vi "Autonomous Independent.vi"() -> ()   [LabVIEW 2017]
doc: "This VI is called when autonomous begins, and will automatically be terminated when autonomous ends. You can carry out timed or sensor driven robot movement independently without needing to return to the caller."
uses:
  <vilib>/Rock Robotics/WPI/Utilities/WPI_GetSetVariantRefNum.vi
  <vilib>/Rock Robotics/Network Tables/NT Read String.vi
  <vilib>/Rock Robotics/Network Tables/NT Write Numeric Array.vi
  Robot Global Data.vi
  <vilib>/Rock Robotics/WPI/Solenoid/Deprecated/WPI_SolenoidSetBool.vi
  <vilib>/addons/control/pid/pid.llb/PID (DBL).vi
  <vilib>/addons/control/pid/NI_PID_pid.lvlib
panel:
  in  "Testing":T1(array[cluster])=[{"Left In/s"=0.0, "Right In/s"=0.0, "Duration"=0.5, "SOL A"=FALSE, "SOL B"=TRUE, "Lift Up"=TRUE, "Lift Down"=FALSE, "Intake In"=FALSE, "Intake Out"=FALSE, "Left Distance"=1.0, "Right Distance"=1.0, "Encoder Reset"=TRUE, "Wrist Up"=FALSE, "Wrist Down"=FALSE, "Lift Target"=0.0, "Wrist Target"=0.0}, {"Left In/s"=-1.0, "Right In/s"=-0.975, "Duration"=5.0, "SOL A"=FALSE, "SOL B"=TRUE, "Lift Up"=FALSE, "Lift Down"=FALSE, "Intake In"=FALSE, "Intake Out"=FALSE, "Left Distance"=300.0, "Right Distance"=300.0, "Encoder Reset"=FALSE, "Wrist Up"=FALSE, "Wrist Down"=FALSE, "Lift Target"=0.0, "Wrist Target"=0.0}, {"Left In/s"=0.0, "Right In/s"=0.0, "Duration"=0.5, "SOL A"=FALSE, "SOL B"=TRUE, "Lift Up"=FALSE, "Lift Down"=FALSE, "Intake In"=FALSE, "Intake Out"=FALSE, "Left Distance"=0.0, "Right Distance"=0.0, "Encoder Reset"=TRUE, "Wrist Up"=FALSE, "Wrist Down"=FALSE, "Lift Target"=0.0, "Wrist Target"=0.0}, {"Left In/s"=1.0, "Right In/s"=-0.975, "Duration"=5.0, "SOL A"=FALSE, "SOL B"=TRUE, "Lift Up"=FALSE, "Lift Down"=FALSE, "Intake In"=FALSE, "Intake Out"=FALSE, "Left Distance"=24.0, "Right Distance"=24.0, "Encoder Reset"=FALSE, "Wrist Up"=FALSE, "Wrist Down"=FALSE, "Lift Target"=0.0, "Wrist Target"=0.0}, {"Left In/s"=0.0, "Right In/s"=0.0, "Duration"=5.0, "SOL A"=FALSE, "SOL B"=TRUE, "Lift Up"=TRUE, "Lift Down"=FALSE, "Intake In"=FALSE, "Intake Out"=FALSE, "Left Distance"=10.0, "Right Distance"=10.0, "Encoder Reset"=FALSE, "Wrist Up"=FALSE, "Wrist Down"=FALSE, "Lift Target"=0.0, "Wrist Target"=0.0}, {"Left In/s"=0.0, "Right In/s"=0.0, "Duration"=0.75, "SOL A"=FALSE, "SOL B"=TRUE, "Lift Up"=FALSE, "Lift Down"=FALSE, "Intake In"=FALSE, "Intake Out"=TRUE, "Left Distance"=10.0, "Right Distance"=10.0, "Encoder Reset"=FALSE, "Wrist Up"=FALSE, "Wrist Down"=FALSE, "Lift Target"=0.0, "Wrist Target"=0.0}]
  in  "Right LLL":T2(array[cluster])=[{"Left Joystick"=1.0, "Right Joystick"=1.0, "Duration"=5.0, "SOL A"=FALSE, "SOL B"=FALSE, "Lift Up"=FALSE, "Lift Down"=FALSE, "Intake In"=FALSE, "Intake Out"=FALSE, "Left Distance"=252.0, "Right Distance"=252.0, "Encoder Reset"=FALSE, "Wrist Up"=FALSE, "Wrist Down"=FALSE}, {"Left Joystick"=-0.75, "Right Joystick"=0.75, "Duration"=2.0, "SOL A"=FALSE, "SOL B"=FALSE, "Lift Up"=FALSE, "Lift Down"=FALSE, "Intake In"=FALSE, "Intake Out"=FALSE, "Left Distance"=31.5, "Right Distance"=31.5, "Encoder Reset"=FALSE, "Wrist Up"=FALSE, "Wrist Down"=FALSE}]
  in  "Right RLR":T2(array[cluster])=[{"Left Joystick"=1.0, "Right Joystick"=1.0, "Duration"=5.0, "SOL A"=FALSE, "SOL B"=FALSE, "Lift Up"=FALSE, "Lift Down"=FALSE, "Intake In"=FALSE, "Intake Out"=FALSE, "Left Distance"=252.0, "Right Distance"=252.0, "Encoder Reset"=FALSE, "Wrist Up"=FALSE, "Wrist Down"=FALSE}, {"Left Joystick"=-0.75, "Right Joystick"=0.75, "Duration"=2.0, "SOL A"=FALSE, "SOL B"=FALSE, "Lift Up"=FALSE, "Lift Down"=FALSE, "Intake In"=FALSE, "Intake Out"=FALSE, "Left Distance"=31.5, "Right Distance"=31.5, "Encoder Reset"=FALSE, "Wrist Up"=FALSE, "Wrist Down"=FALSE}]
  in  "Right LRL":T2(array[cluster])=[{"Left Joystick"=1.0, "Right Joystick"=1.0, "Duration"=5.0, "SOL A"=FALSE, "SOL B"=FALSE, "Lift Up"=FALSE, "Lift Down"=FALSE, "Intake In"=FALSE, "Intake Out"=FALSE, "Left Distance"=252.0, "Right Distance"=252.0, "Encoder Reset"=FALSE, "Wrist Up"=FALSE, "Wrist Down"=FALSE}, {"Left Joystick"=-0.75, "Right Joystick"=0.75, "Duration"=2.0, "SOL A"=FALSE, "SOL B"=FALSE, "Lift Up"=FALSE, "Lift Down"=FALSE, "Intake In"=FALSE, "Intake Out"=FALSE, "Left Distance"=31.5, "Right Distance"=31.5, "Encoder Reset"=FALSE, "Wrist Up"=FALSE, "Wrist Down"=FALSE}]
  in  "Right RRR":T2(array[cluster])=[{"Left Joystick"=1.0, "Right Joystick"=1.0, "Duration"=5.0, "SOL A"=FALSE, "SOL B"=FALSE, "Lift Up"=FALSE, "Lift Down"=FALSE, "Intake In"=FALSE, "Intake Out"=FALSE, "Left Distance"=252.0, "Right Distance"=252.0, "Encoder Reset"=FALSE, "Wrist Up"=FALSE, "Wrist Down"=FALSE}, {"Left Joystick"=-0.75, "Right Joystick"=0.75, "Duration"=2.0, "SOL A"=FALSE, "SOL B"=FALSE, "Lift Up"=FALSE, "Lift Down"=FALSE, "Intake In"=FALSE, "Intake Out"=FALSE, "Left Distance"=31.5, "Right Distance"=31.5, "Encoder Reset"=FALSE, "Wrist Up"=FALSE, "Wrist Down"=FALSE}]
  in  "Center LLL":T2(array[cluster])=[{"Left Joystick"=1.0, "Right Joystick"=1.0, "Duration"=5.0, "SOL A"=FALSE, "SOL B"=FALSE, "Lift Up"=FALSE, "Lift Down"=FALSE, "Intake In"=FALSE, "Intake Out"=FALSE, "Left Distance"=252.0, "Right Distance"=252.0, "Encoder Reset"=FALSE, "Wrist Up"=FALSE, "Wrist Down"=FALSE}, {"Left Joystick"=-0.75, "Right Joystick"=0.75, "Duration"=2.0, "SOL A"=FALSE, "SOL B"=FALSE, "Lift Up"=FALSE, "Lift Down"=FALSE, "Intake In"=FALSE, "Intake Out"=FALSE, "Left Distance"=31.5, "Right Distance"=31.5, "Encoder Reset"=FALSE, "Wrist Up"=FALSE, "Wrist Down"=FALSE}]
  in  "Center RLR":T2(array[cluster])=[{"Left Joystick"=1.0, "Right Joystick"=1.0, "Duration"=5.0, "SOL A"=FALSE, "SOL B"=FALSE, "Lift Up"=FALSE, "Lift Down"=FALSE, "Intake In"=FALSE, "Intake Out"=FALSE, "Left Distance"=252.0, "Right Distance"=252.0, "Encoder Reset"=FALSE, "Wrist Up"=FALSE, "Wrist Down"=FALSE}, {"Left Joystick"=-0.75, "Right Joystick"=0.75, "Duration"=2.0, "SOL A"=FALSE, "SOL B"=FALSE, "Lift Up"=FALSE, "Lift Down"=FALSE, "Intake In"=FALSE, "Intake Out"=FALSE, "Left Distance"=31.5, "Right Distance"=31.5, "Encoder Reset"=FALSE, "Wrist Up"=FALSE, "Wrist Down"=FALSE}]
  in  "Center LRL":T2(array[cluster])=[{"Left Joystick"=1.0, "Right Joystick"=1.0, "Duration"=5.0, "SOL A"=FALSE, "SOL B"=FALSE, "Lift Up"=FALSE, "Lift Down"=FALSE, "Intake In"=FALSE, "Intake Out"=FALSE, "Left Distance"=252.0, "Right Distance"=252.0, "Encoder Reset"=FALSE, "Wrist Up"=FALSE, "Wrist Down"=FALSE}, {"Left Joystick"=-0.75, "Right Joystick"=0.75, "Duration"=2.0, "SOL A"=FALSE, "SOL B"=FALSE, "Lift Up"=FALSE, "Lift Down"=FALSE, "Intake In"=FALSE, "Intake Out"=FALSE, "Left Distance"=31.5, "Right Distance"=31.5, "Encoder Reset"=FALSE, "Wrist Up"=FALSE, "Wrist Down"=FALSE}]
  in  "Center RRR":T2(array[cluster])=[{"Left Joystick"=1.0, "Right Joystick"=1.0, "Duration"=5.0, "SOL A"=FALSE, "SOL B"=FALSE, "Lift Up"=FALSE, "Lift Down"=FALSE, "Intake In"=FALSE, "Intake Out"=FALSE, "Left Distance"=252.0, "Right Distance"=252.0, "Encoder Reset"=FALSE, "Wrist Up"=FALSE, "Wrist Down"=FALSE}, {"Left Joystick"=-0.75, "Right Joystick"=0.75, "Duration"=2.0, "SOL A"=FALSE, "SOL B"=FALSE, "Lift Up"=FALSE, "Lift Down"=FALSE, "Intake In"=FALSE, "Intake Out"=FALSE, "Left Distance"=31.5, "Right Distance"=31.5, "Encoder Reset"=FALSE, "Wrist Up"=FALSE, "Wrist Down"=FALSE}]
  in  "Left RLR":T2(array[cluster])=[{"Left Joystick"=1.0, "Right Joystick"=1.0, "Duration"=5.0, "SOL A"=FALSE, "SOL B"=FALSE, "Lift Up"=FALSE, "Lift Down"=FALSE, "Intake In"=FALSE, "Intake Out"=FALSE, "Left Distance"=252.0, "Right Distance"=252.0, "Encoder Reset"=FALSE, "Wrist Up"=FALSE, "Wrist Down"=FALSE}, {"Left Joystick"=-0.75, "Right Joystick"=0.75, "Duration"=2.0, "SOL A"=FALSE, "SOL B"=FALSE, "Lift Up"=FALSE, "Lift Down"=FALSE, "Intake In"=FALSE, "Intake Out"=FALSE, "Left Distance"=31.5, "Right Distance"=31.5, "Encoder Reset"=FALSE, "Wrist Up"=FALSE, "Wrist Down"=FALSE}]
  in  "Left LRL":T2(array[cluster])=[{"Left Joystick"=1.0, "Right Joystick"=1.0, "Duration"=5.0, "SOL A"=FALSE, "SOL B"=FALSE, "Lift Up"=FALSE, "Lift Down"=FALSE, "Intake In"=FALSE, "Intake Out"=FALSE, "Left Distance"=252.0, "Right Distance"=252.0, "Encoder Reset"=FALSE, "Wrist Up"=FALSE, "Wrist Down"=FALSE}, {"Left Joystick"=-0.75, "Right Joystick"=0.75, "Duration"=2.0, "SOL A"=FALSE, "SOL B"=FALSE, "Lift Up"=FALSE, "Lift Down"=FALSE, "Intake In"=FALSE, "Intake Out"=FALSE, "Left Distance"=31.5, "Right Distance"=31.5, "Encoder Reset"=FALSE, "Wrist Up"=FALSE, "Wrist Down"=FALSE}]
  in  "Left RRR":T2(array[cluster])=[{"Left Joystick"=1.0, "Right Joystick"=1.0, "Duration"=5.0, "SOL A"=FALSE, "SOL B"=FALSE, "Lift Up"=FALSE, "Lift Down"=FALSE, "Intake In"=FALSE, "Intake Out"=FALSE, "Left Distance"=252.0, "Right Distance"=252.0, "Encoder Reset"=FALSE, "Wrist Up"=FALSE, "Wrist Down"=FALSE}, {"Left Joystick"=-0.75, "Right Joystick"=0.75, "Duration"=2.0, "SOL A"=FALSE, "SOL B"=FALSE, "Lift Up"=FALSE, "Lift Down"=FALSE, "Intake In"=FALSE, "Intake Out"=FALSE, "Left Distance"=31.5, "Right Distance"=31.5, "Encoder Reset"=FALSE, "Wrist Up"=FALSE, "Wrist Down"=FALSE}]
  in  "Left LLL":T2(array[cluster])=[{"Left Joystick"=1.0, "Right Joystick"=1.0, "Duration"=5.0, "SOL A"=FALSE, "SOL B"=FALSE, "Lift Up"=FALSE, "Lift Down"=FALSE, "Intake In"=FALSE, "Intake Out"=FALSE, "Left Distance"=60.0, "Right Distance"=60.0, "Encoder Reset"=FALSE, "Wrist Up"=FALSE, "Wrist Down"=FALSE}, {"Left Joystick"=-0.75, "Right Joystick"=0.75, "Duration"=2.0, "SOL A"=FALSE, "SOL B"=FALSE, "Lift Up"=FALSE, "Lift Down"=FALSE, "Intake In"=FALSE, "Intake Out"=FALSE, "Left Distance"=31.5, "Right Distance"=31.5, "Encoder Reset"=FALSE, "Wrist Up"=FALSE, "Wrist Down"=FALSE}]
  # "Be sure to right-click and choose Data Operations>>Make Current Value default if you want to save the array values with the VI"
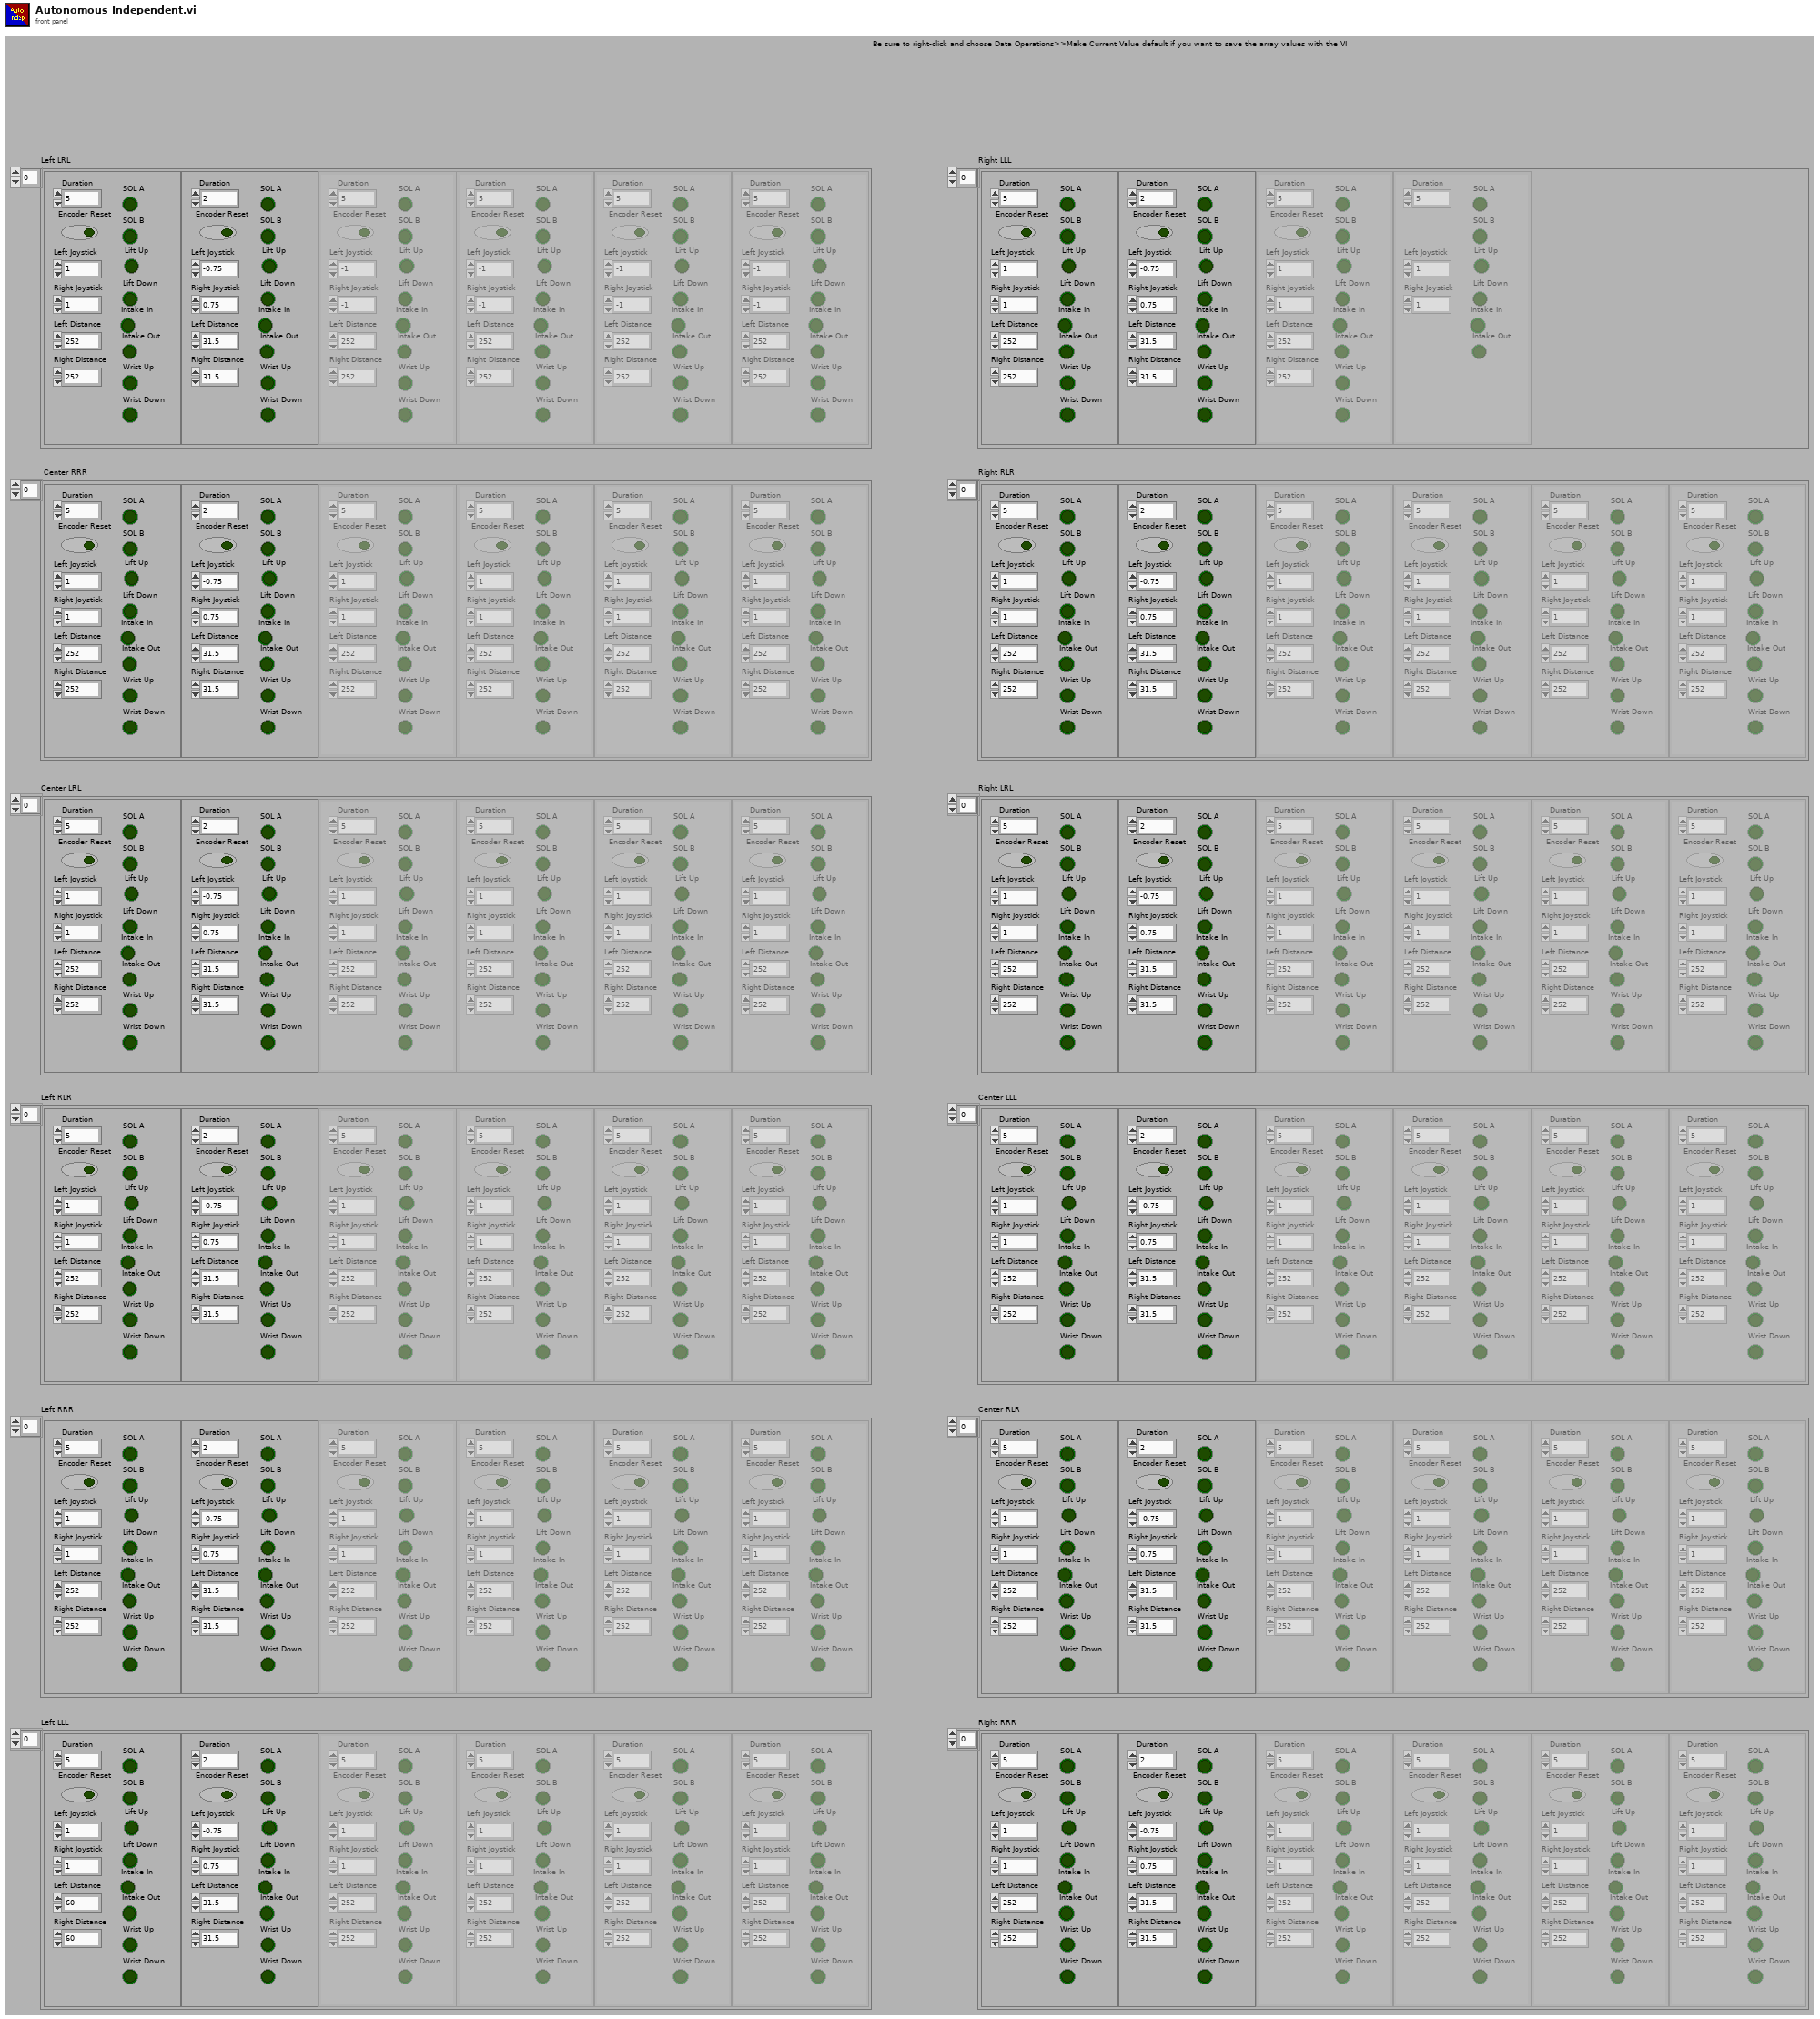
[diagram p1: front panel]
types:
  T1 = cluster{"Left In/s":dbl, "Right In/s":dbl, "Duration":dbl, "SOL A":bool, "SOL B":bool, "Lift Up":bool, "Lift Down":bool, "Intake In":bool, "Intake Out":bool, "Left Distance":dbl, "Right Distance":dbl, "Encoder Reset":bool, "Wrist Up":bool, "Wrist Down":bool, "Lift Target":dbl, "Wrist Target":dbl}[]
  T2 = cluster{"Left Joystick":dbl, "Right Joystick":dbl, "Duration":dbl, "SOL A":bool, "SOL B":bool, "Lift Up":bool, "Lift Down":bool, "Intake In":bool, "Intake Out":bool, "Left Distance":dbl, "Right Distance":dbl, "Encoder Reset":bool, "Wrist Up":bool, "Wrist Down":bool}[]
  T3 = typedef "WPI_JoystickDevRef.ctl" = cluster{"Device":T4}
  T4 = typedef "WPI_JoystickDeviceEnum.ctl" = enum16{"USB 0", "USB 1", "USB 2", "USB 3", "USB 4", "USB 5"}
  T5 = cluster{"proportional gain (Kc)":dbl, "integral time (Ti, min)":dbl, "derivative time (Td, min)":dbl}
  T6 = typedef "WPI_RobotDriveDevRef.ctl" = cluster{"DevStatus":errorcluster, "Motors[]":T7[], "Square Inputs":bool, "Max Output":dbl}
  T7 = typedef "WPI_MotorControlDeviceRef.ctl" = cluster{"DeviceStatus":errorcluster, "Type":T8, "PWM":cluster{"PWM Channel":T9, "DeadBand":T10}, "CAN":cluster{"Device Number":u8, "SetOutput VI Ref":variant, "GetOutput VI Ref":variant, "Enable VI Ref":variant, "Disable VI Ref":variant, "Data":variant}, "Invert":bool, "DIO PWM":cluster{"PWM \"Enable\" Channel":T9, "DIOChannel":T11, "PWM Rate":dbl}}
  T8 = typedef "WPI_MotorControlType.ctl" = enum16{"PWM", "CAN", "DIO PWM"}
  T9 = typedef "FPGA_DIOPWMChannel.ctl" = enum8{"PWM 0", "PWM 1", "PWM 2", "PWM 3", "PWM 4", "PWM 5", "PWM 6", "PWM 7", "PWM 8", "PWM 9", "PWM MXP 0", "PWM MXP 1", "PWM MXP 2", "PWM MXP 3", "PWM MXP 4", "PWM MXP 5", "PWM MXP 6", "PWM MXP 7", "PWM MXP 8", "PWM MXP 9", "Invalid"}
  T10 = typedef "WPI_PWMDeadband.ctl" = cluster{"Name":string, "maxPositivePwm":i32, "minPositivePwm":i32, "centerPwm":i32, "maxNegativePwm":i32, "minNegativePwm":i32, "angularRange":u16}
  T11 = typedef "FPGA_DIOChannel.ctl" = enum8{"DIO 0", "DIO 1", "DIO 2", "DIO 3", "DIO 4", "DIO 5", "DIO 6", "DIO 7", "DIO 8", "DIO 9", "DIO MXP 0", "DIO MXP 1", "DIO MXP 2", "DIO MXP 3", "DIO MXP 4", "DIO MXP 5", "DIO MXP 6", "DIO MXP 7", "DIO MXP 8", "DIO MXP 9", "DIO MXP 10", "DIO MXP 11", "DIO MXP 12", "DIO MXP 13", "DIO MXP 14", "DIO MXP 15", "SPI Port CS1", "SPI Port CS2", "SPI Port CS3", "SPI Port MISO", "SPI Port MOSI", "Invalid"}
  T12 = typedef "WPI_SolenoidDevRef.ctl" = cluster{"DevStatus":errorcluster, "Pneumatics Control Module":u8, "Forward Solenoid Channel":T13, "Reverse Solenoid Channel":T13}
  T13 = typedef "WPI_SolenoidChannel.ctl" = enum8{"Solenoid 0", "Solenoid 1", "Solenoid 2", "Solenoid 3", "Solenoid 4", "Solenoid 5", "Solenoid 6", "Solenoid 7", "Invalid"}
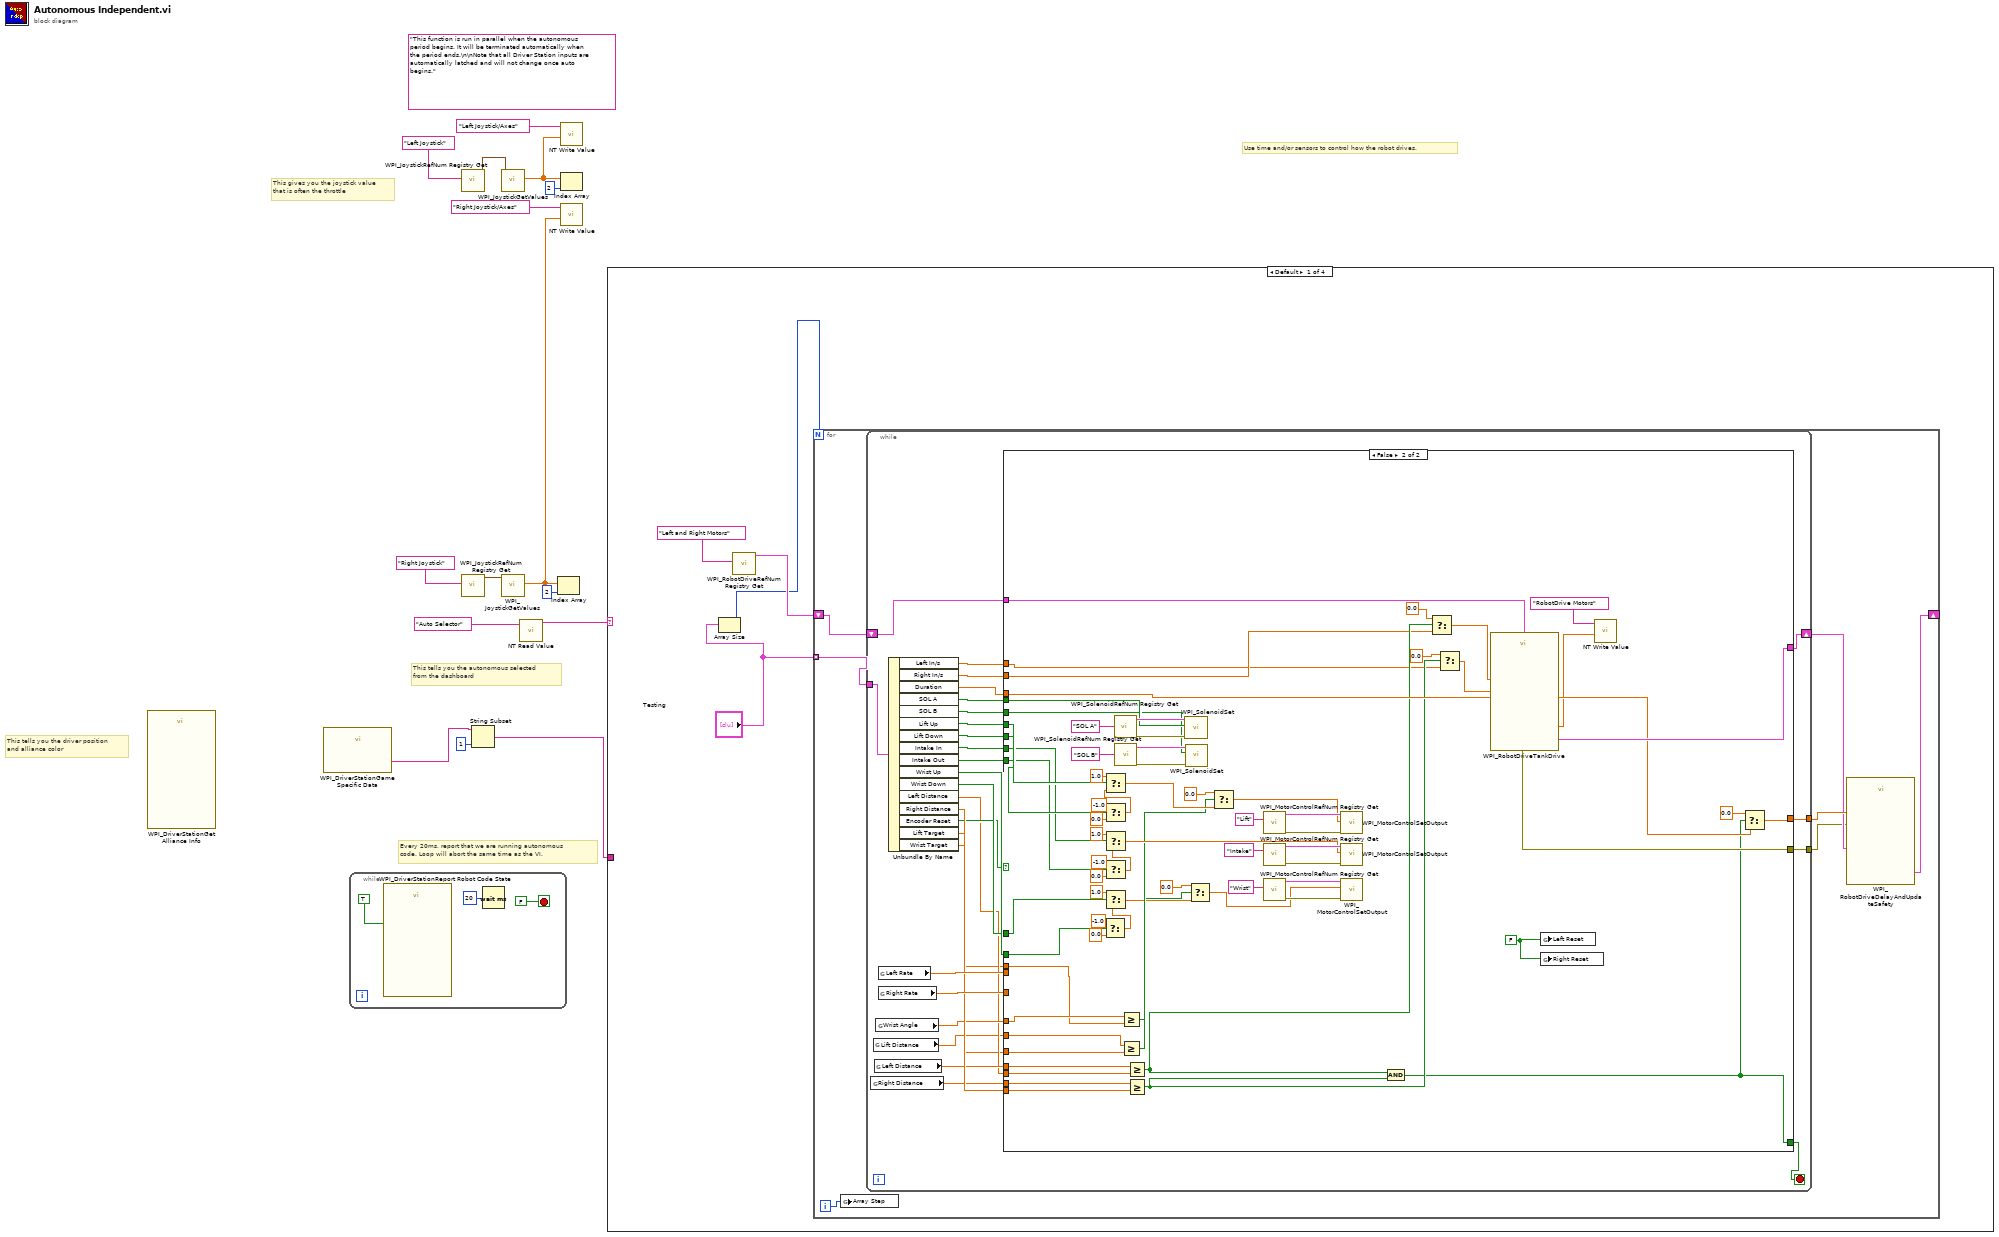
[diagram p0: block diagram]
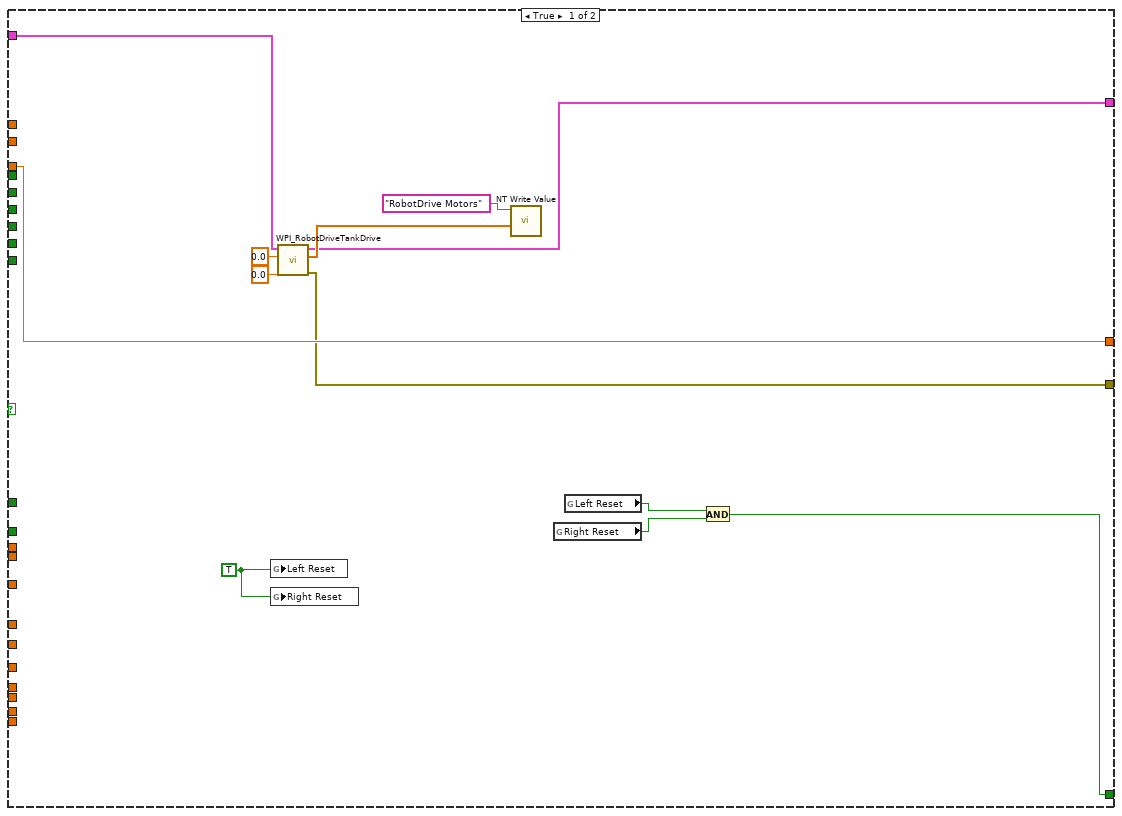
[diagram p2: hidden frame]
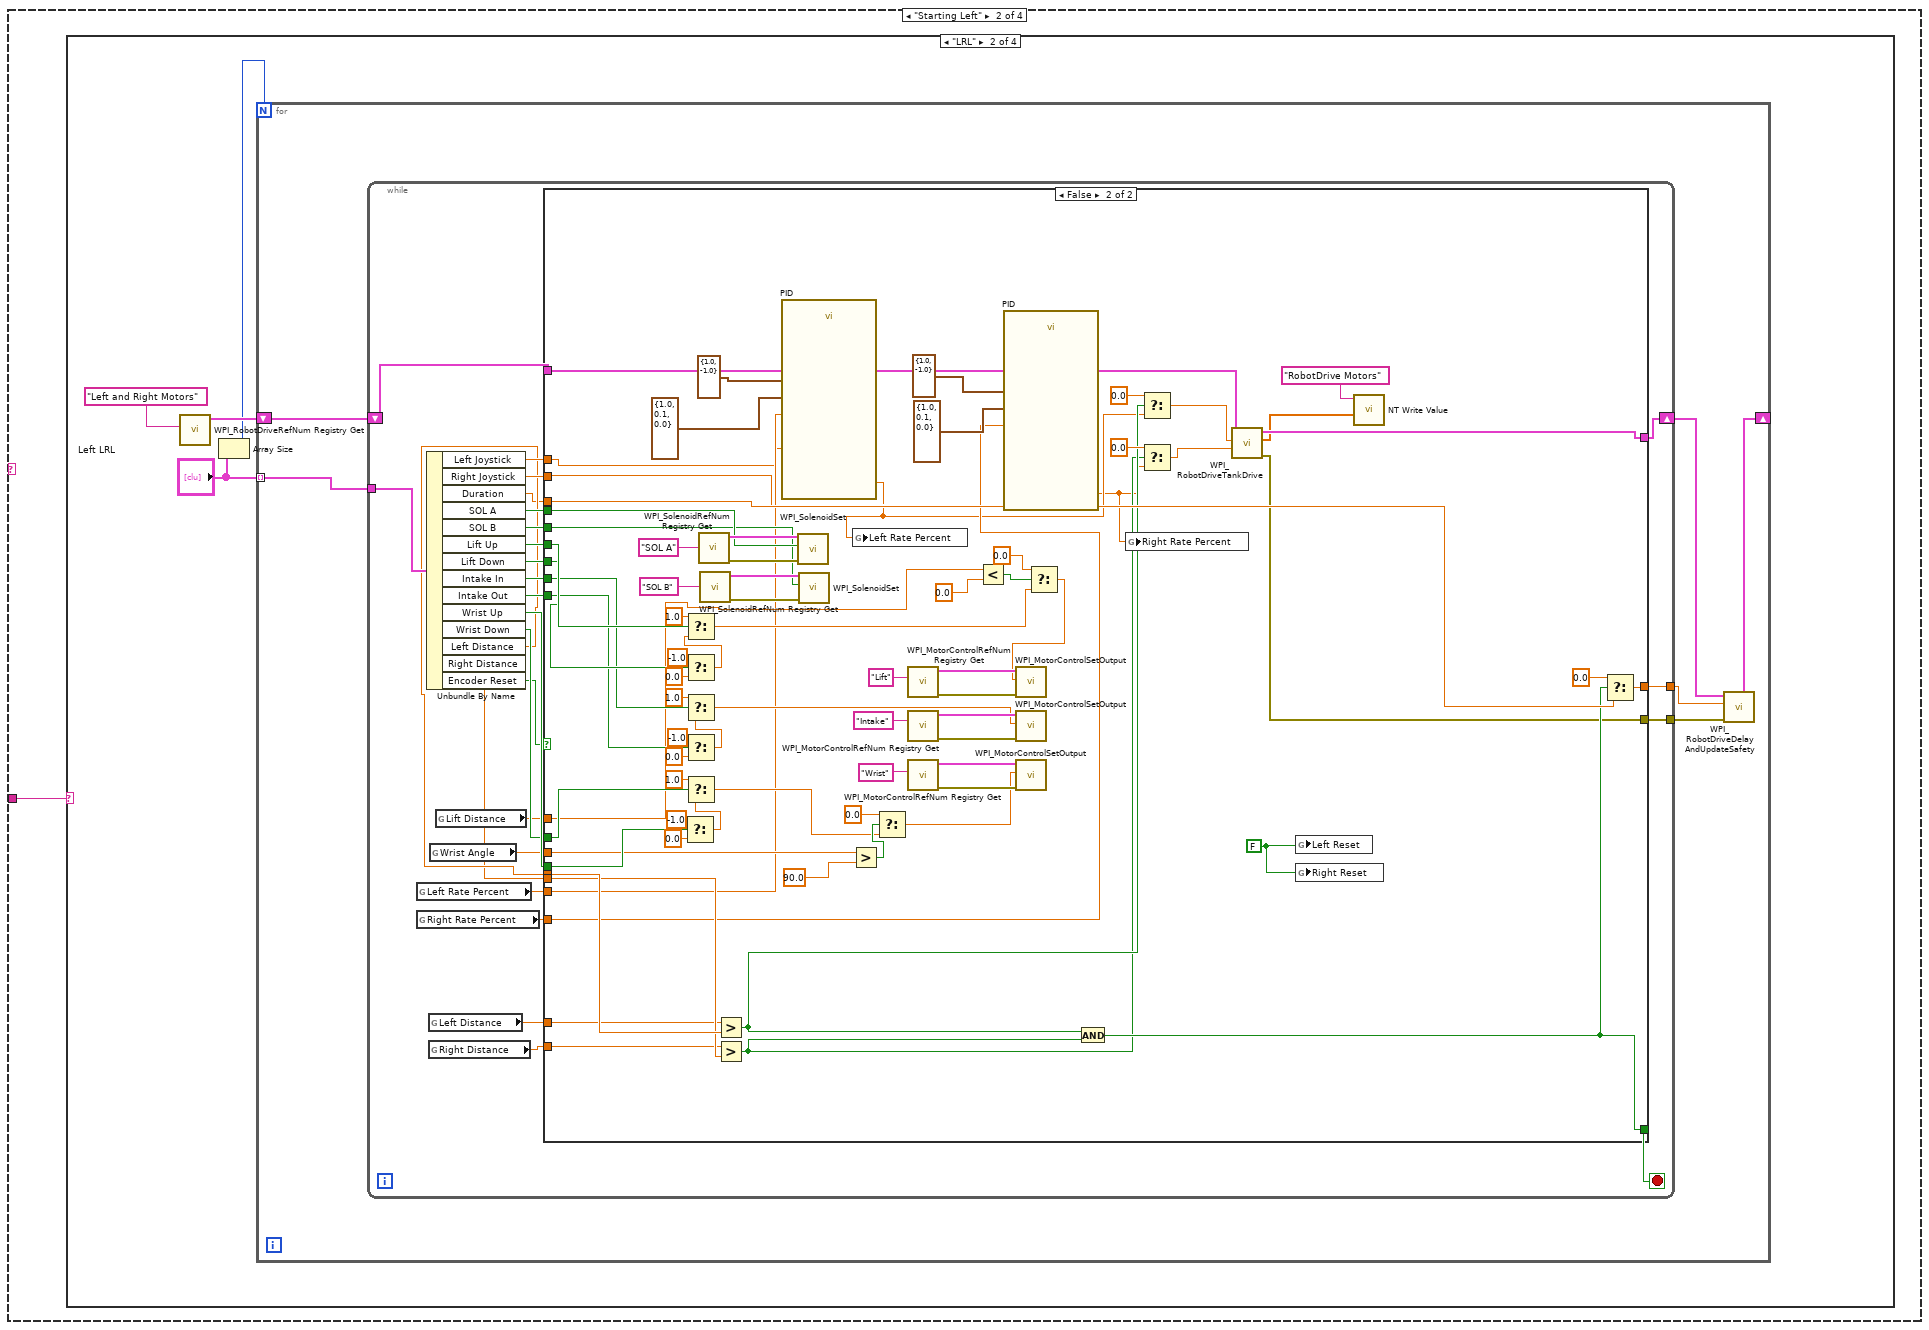
[diagram p3: hidden frame]
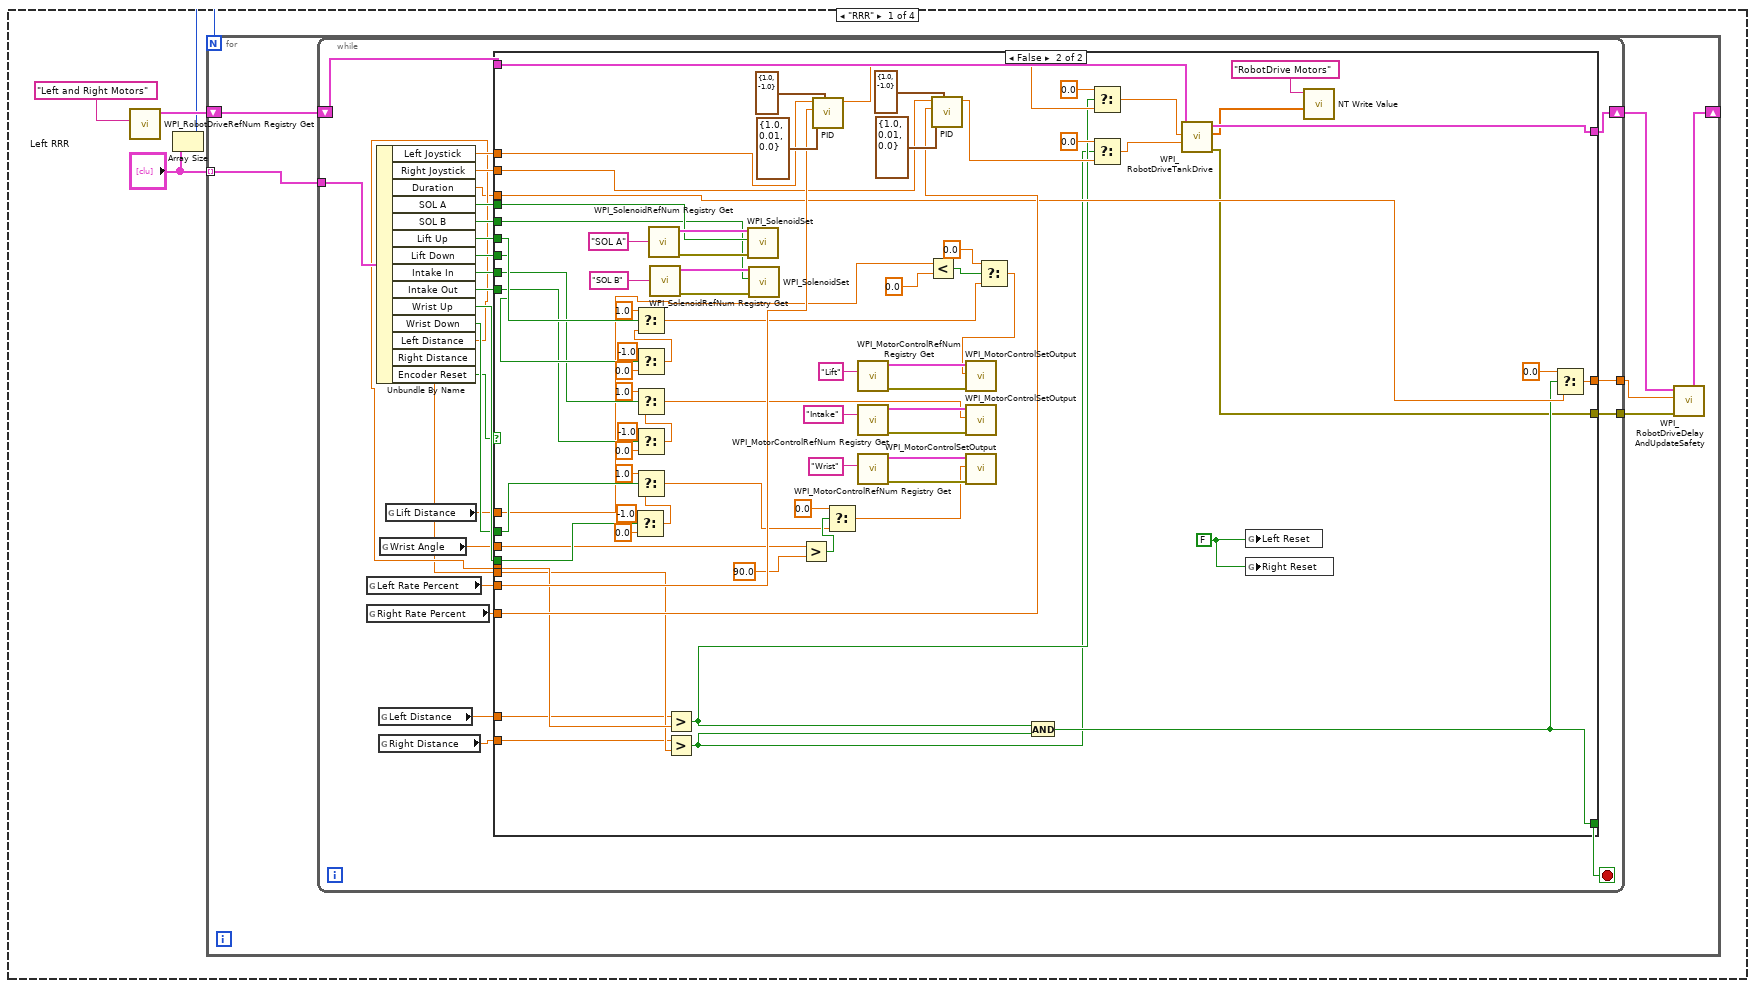
[diagram p4: hidden frame]
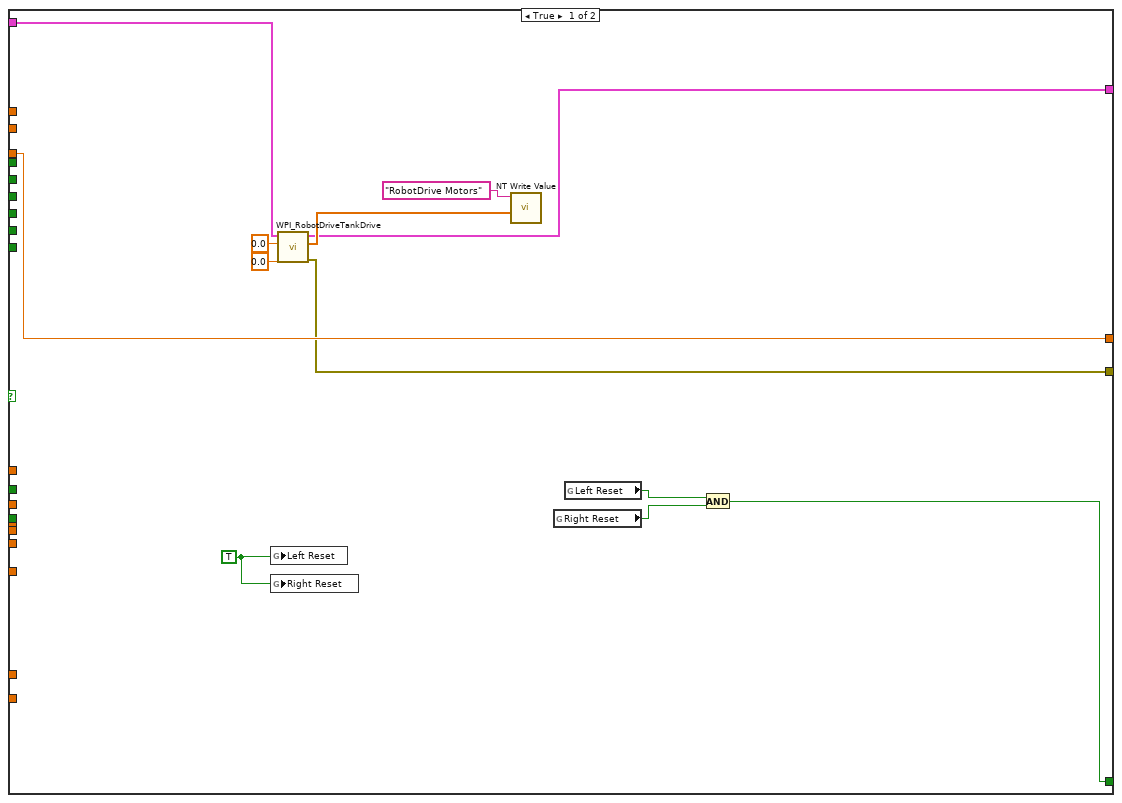
[diagram p5: hidden frame]
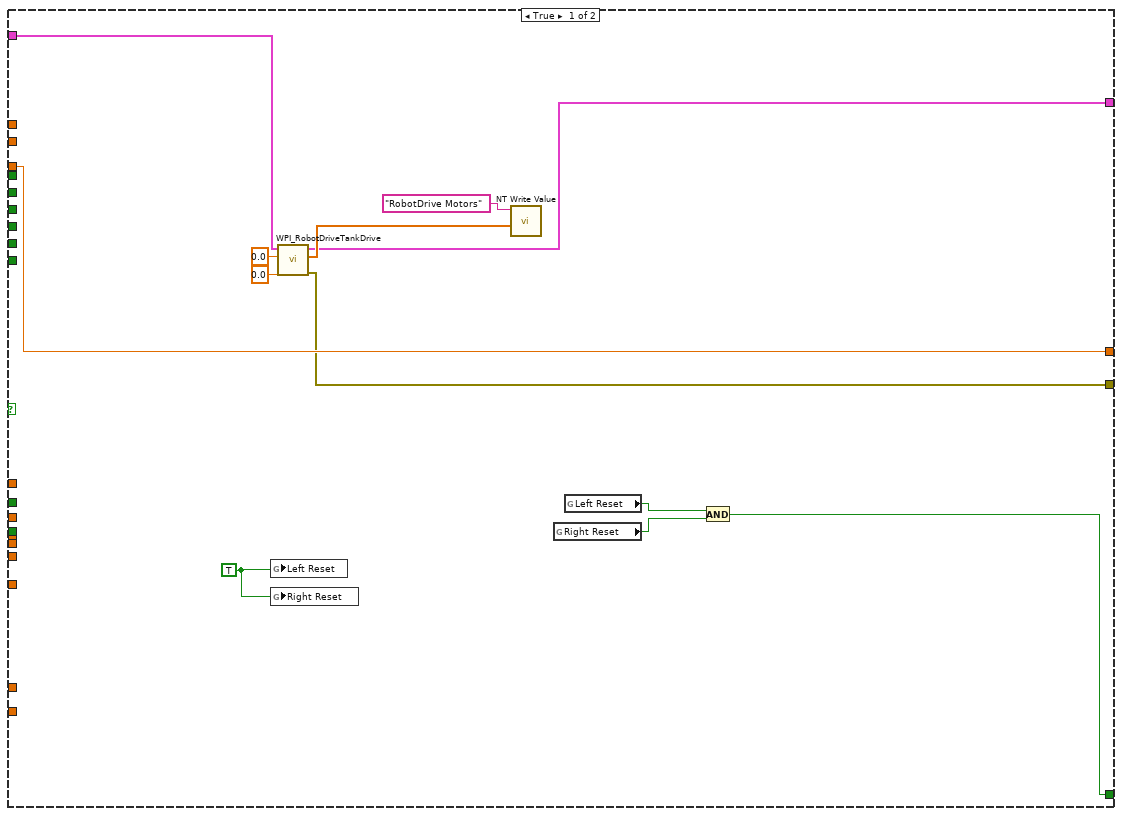
[diagram p6: hidden frame]
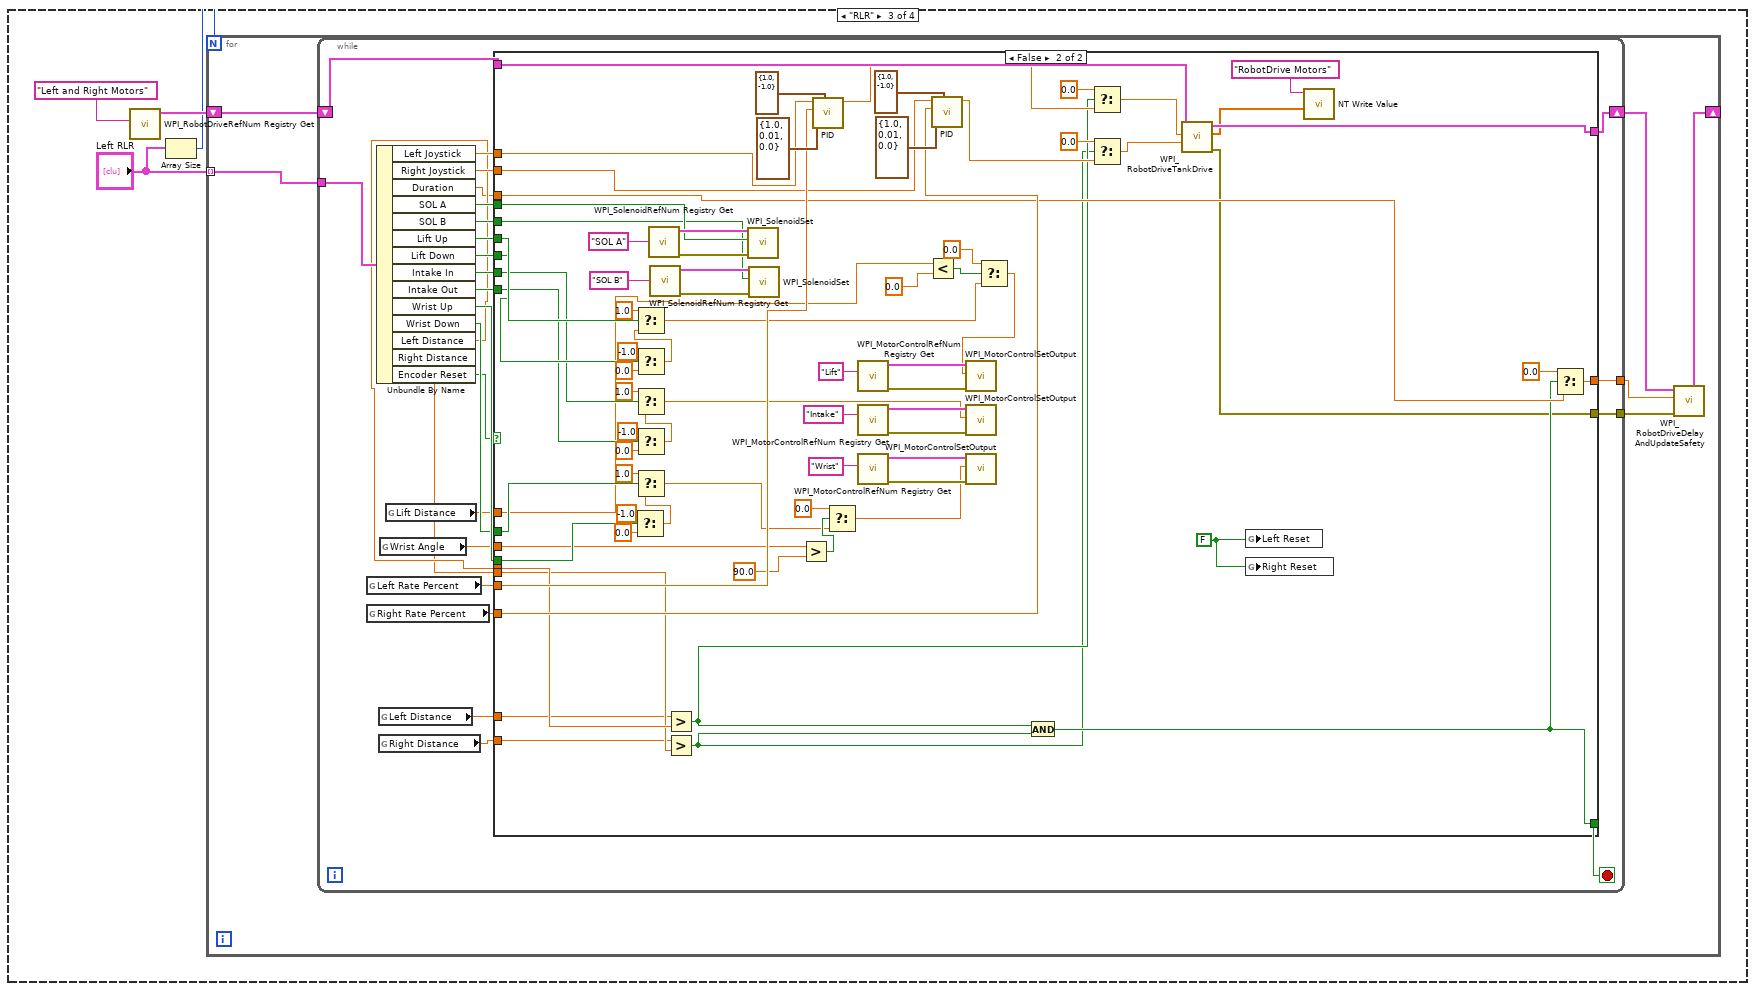
[diagram p7: hidden frame]
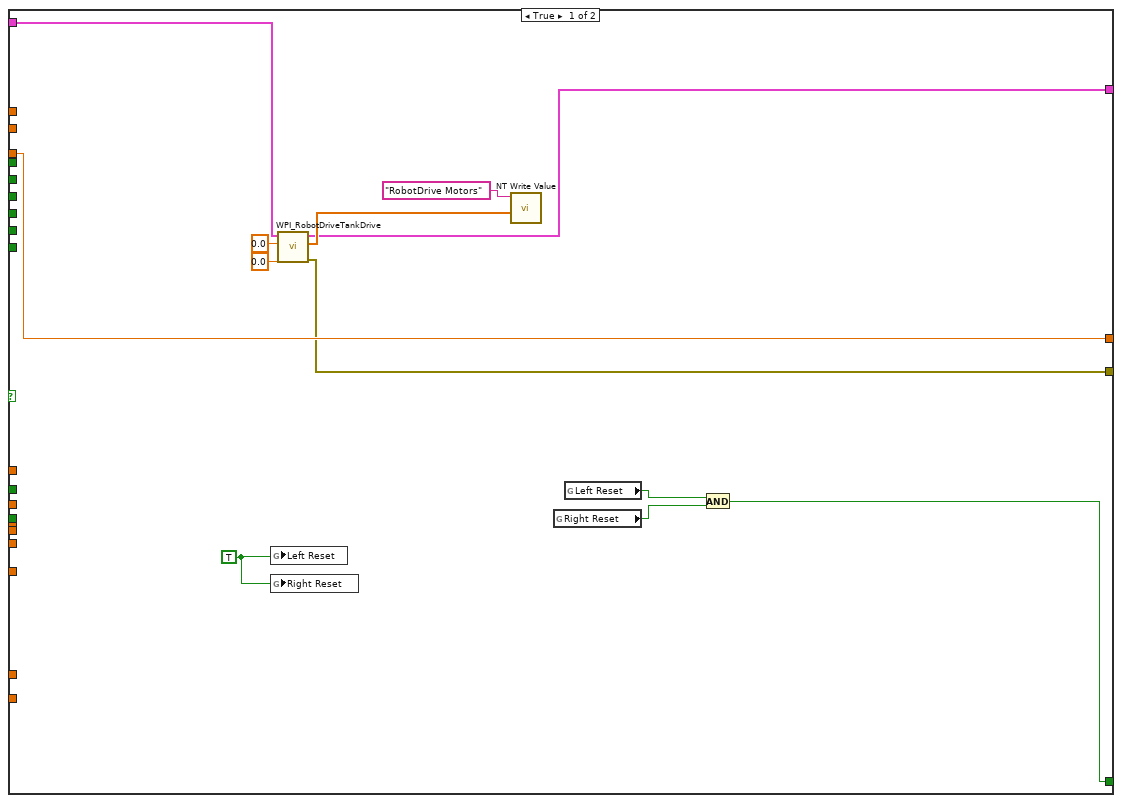
[diagram p8: hidden frame]
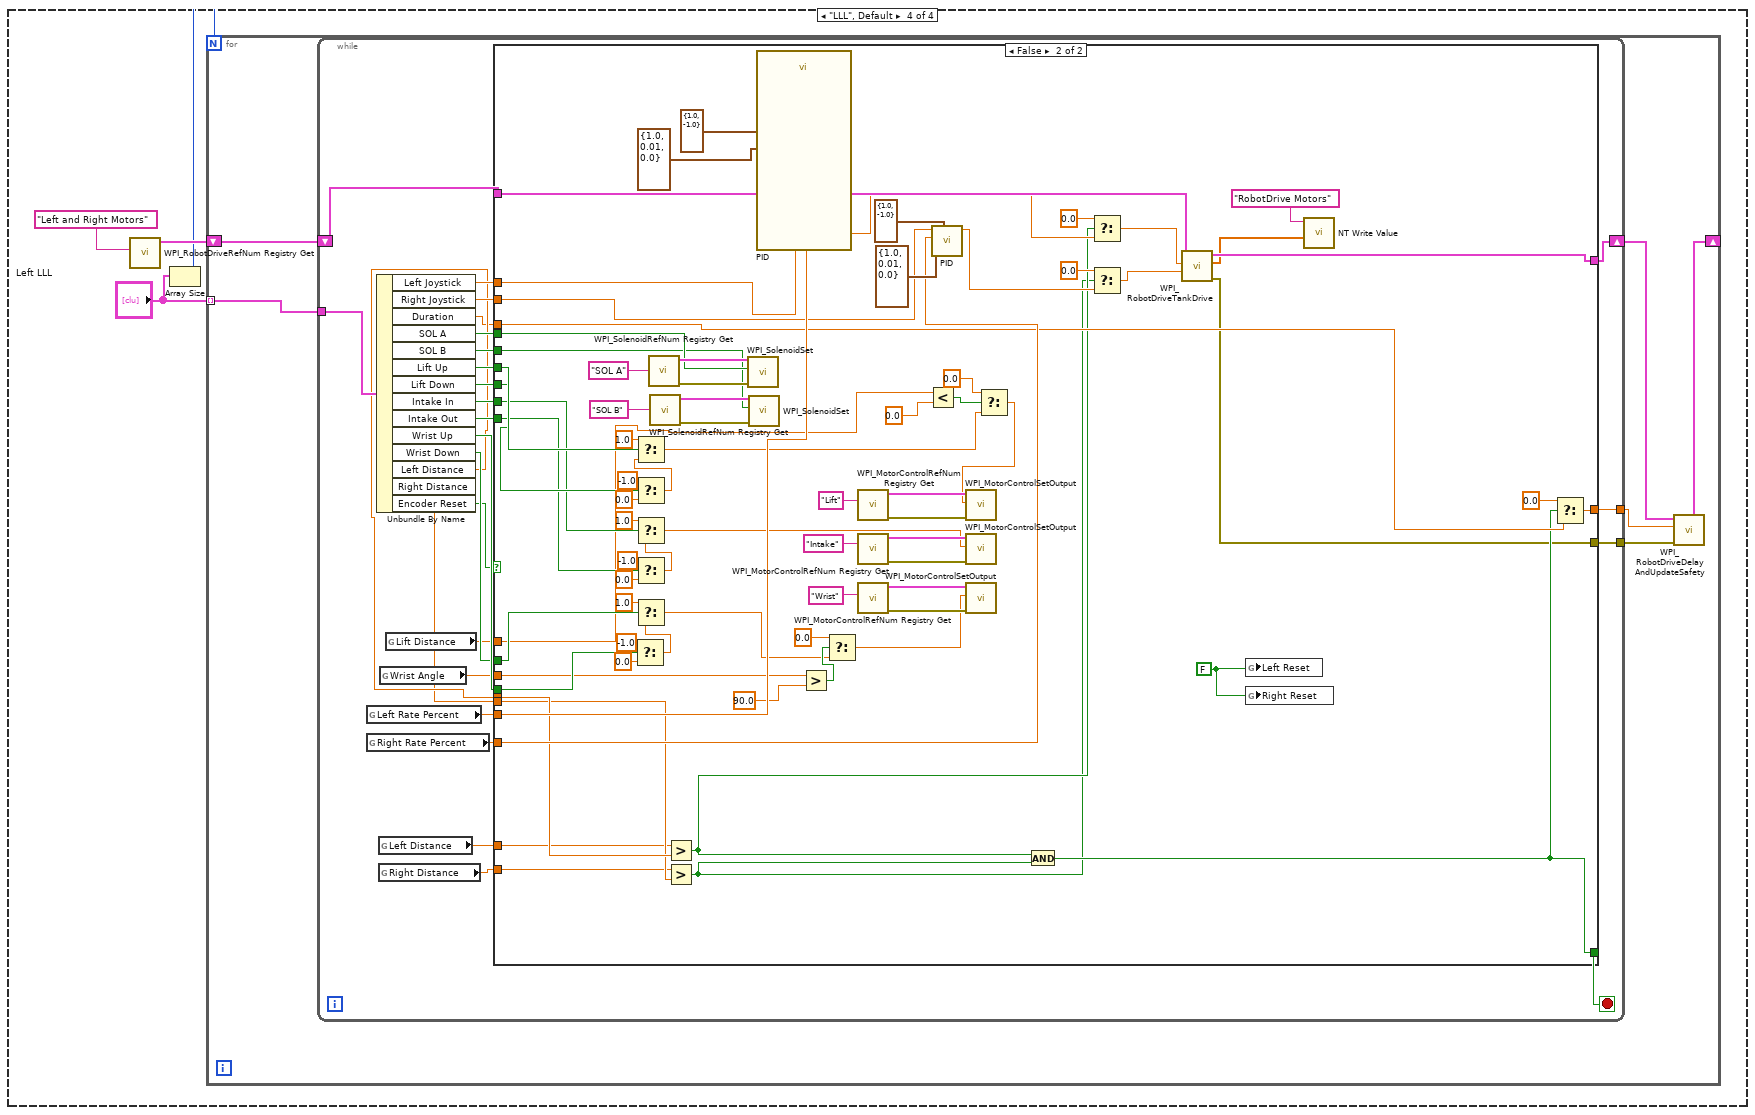
[diagram p9: hidden frame]
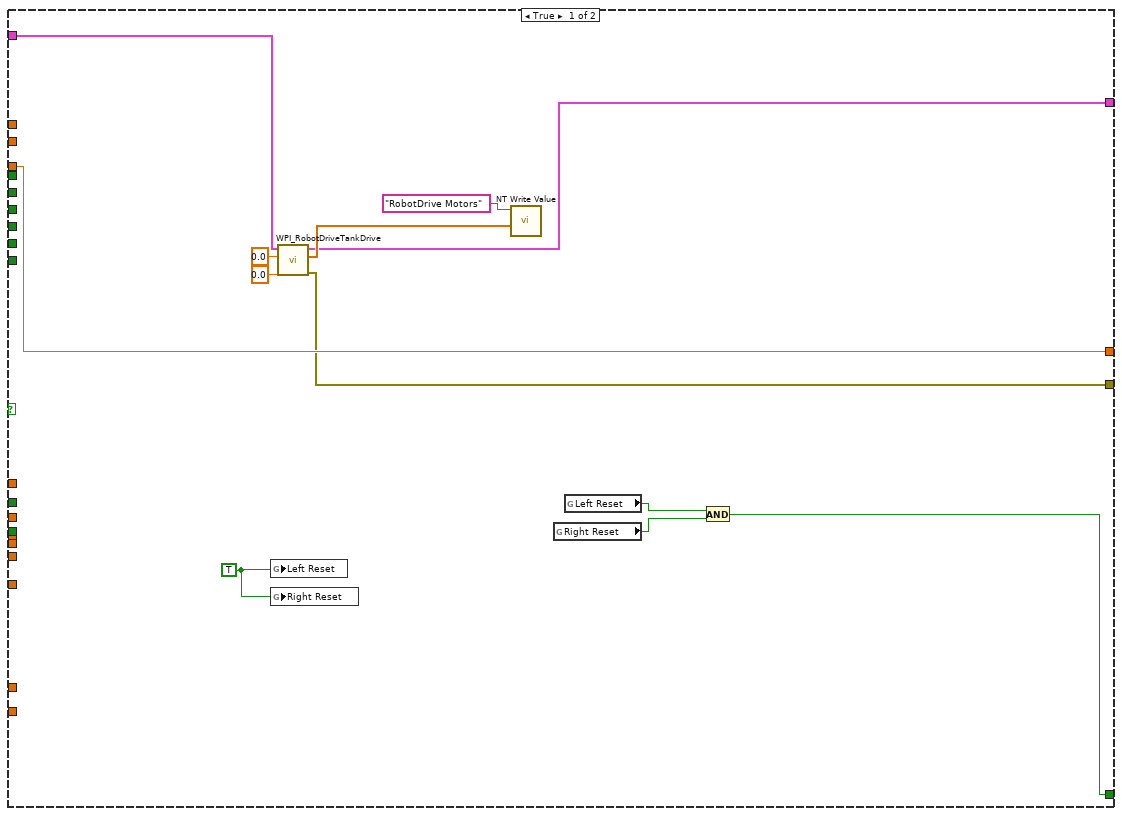
[diagram p10: hidden frame]
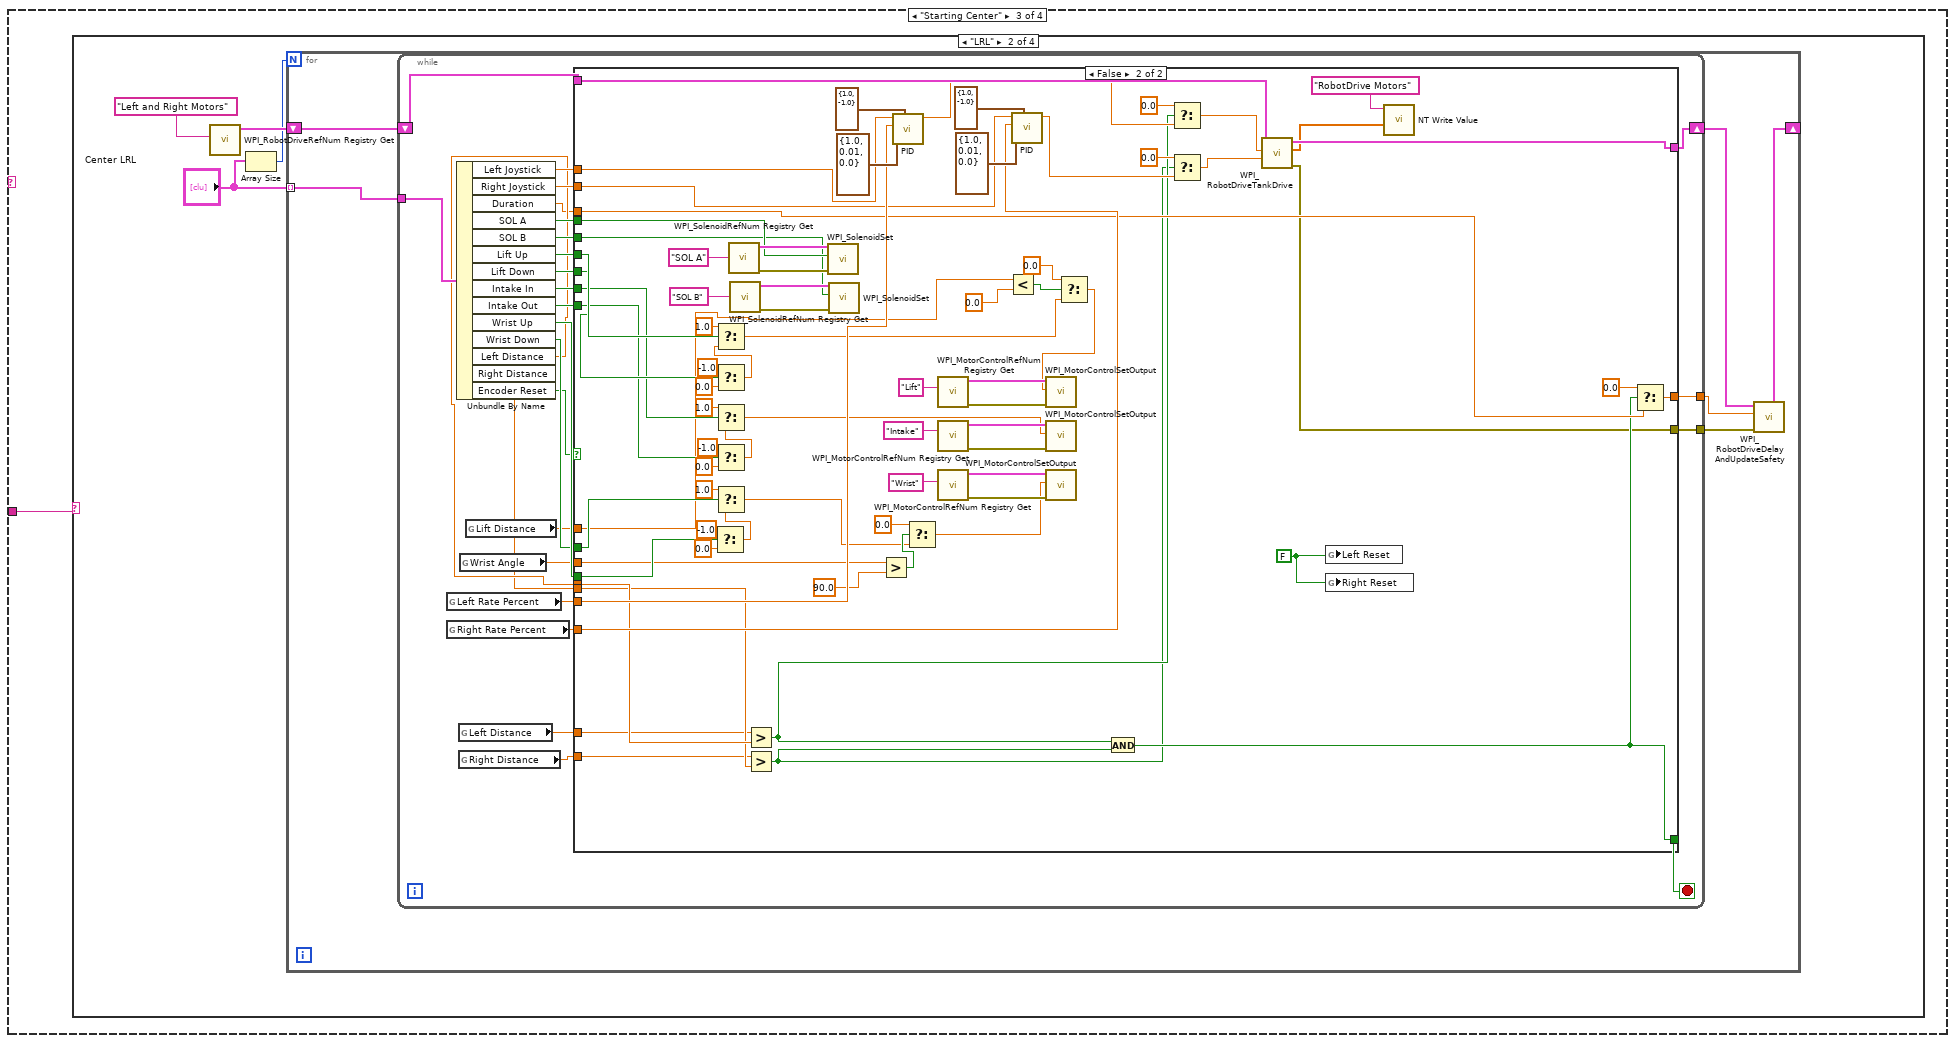
[diagram p11: hidden frame]
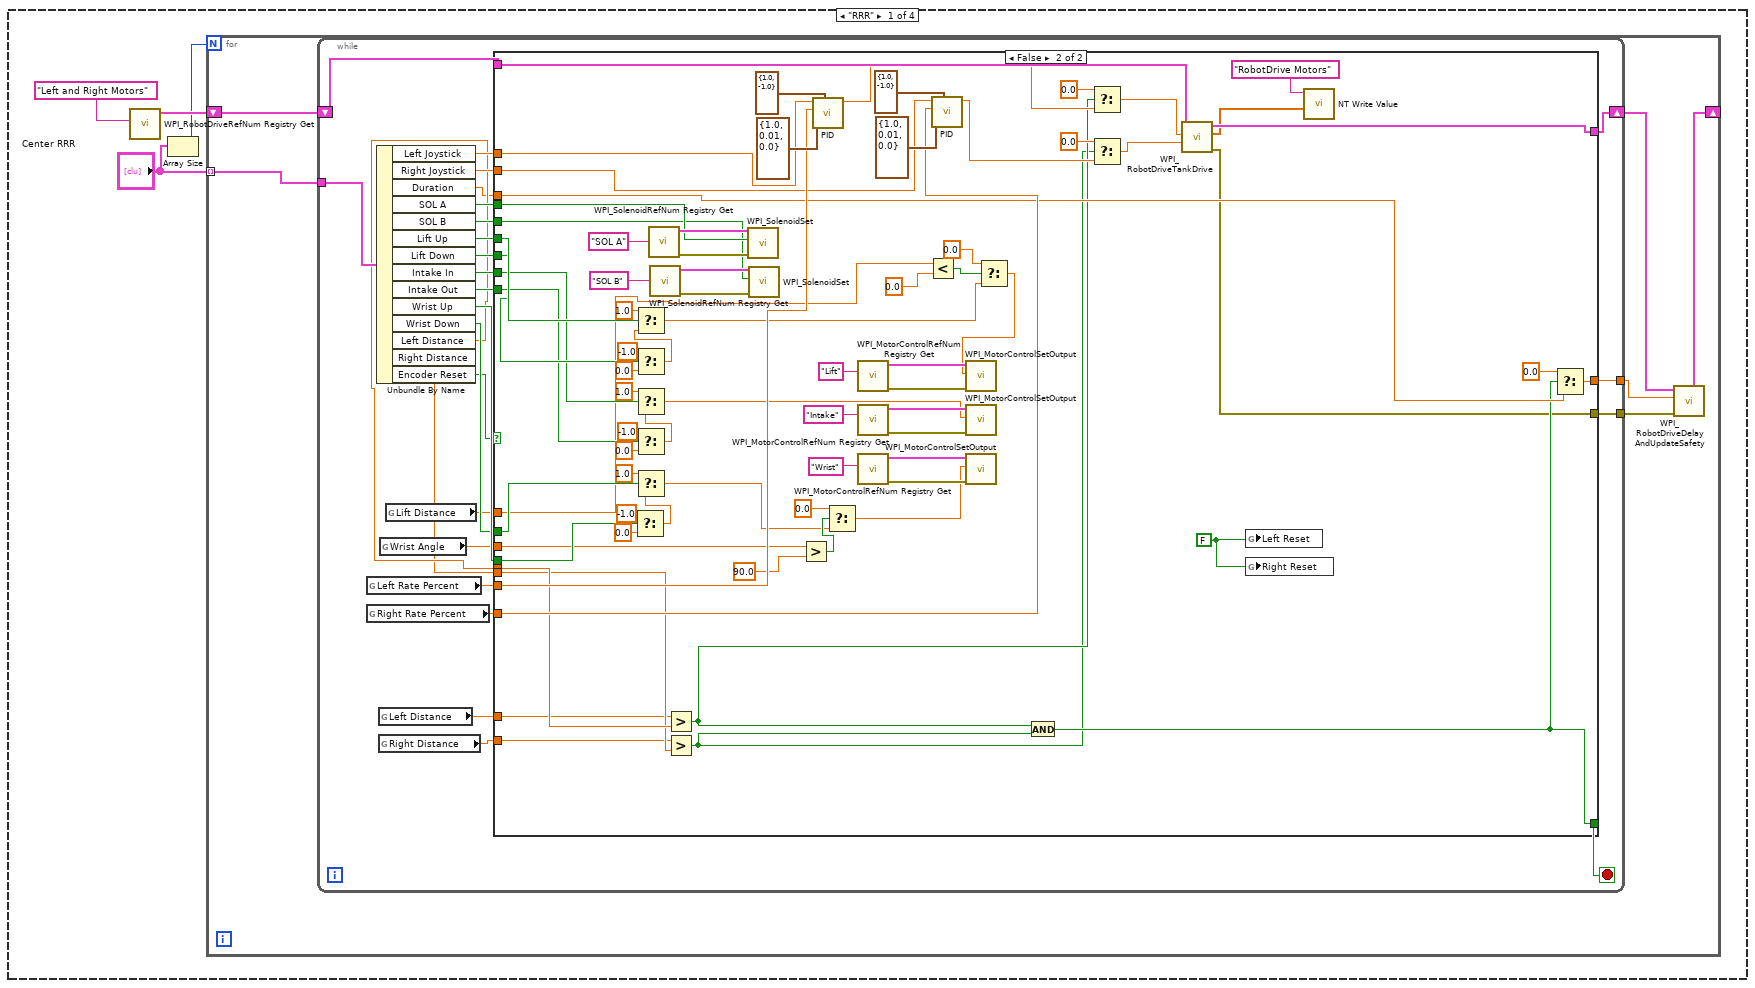
[diagram p12: hidden frame]
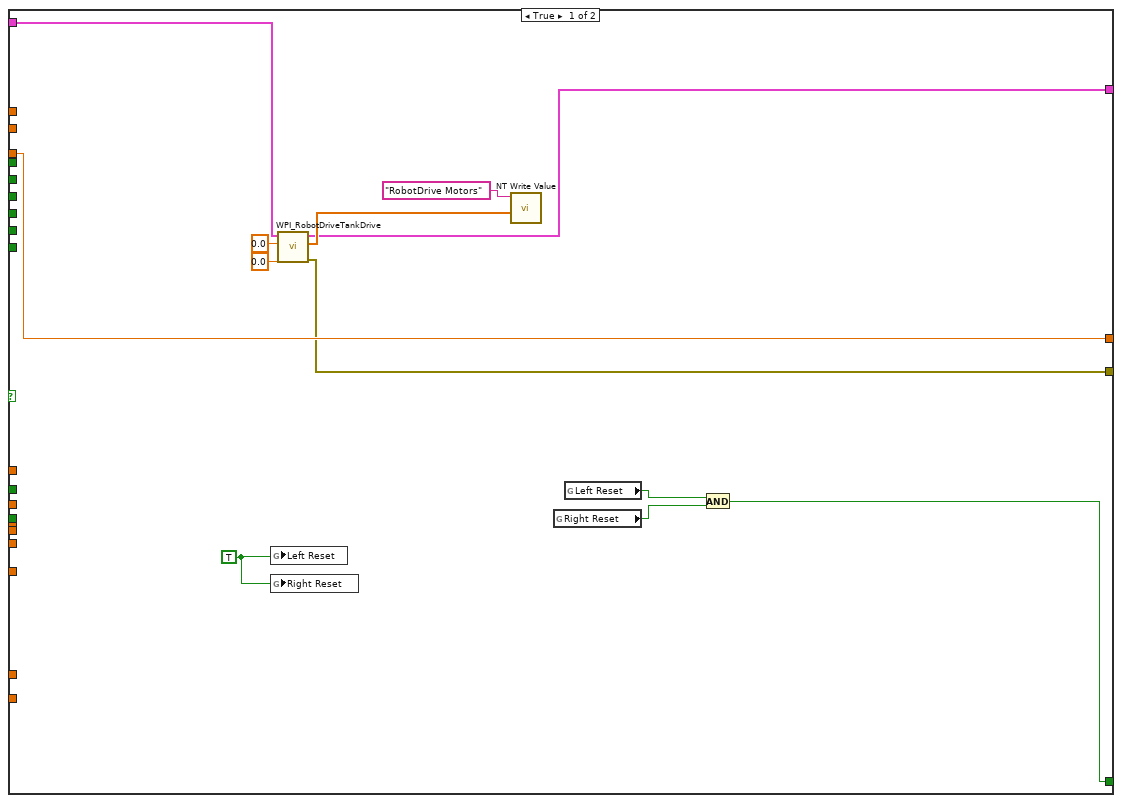
[diagram p13: hidden frame]
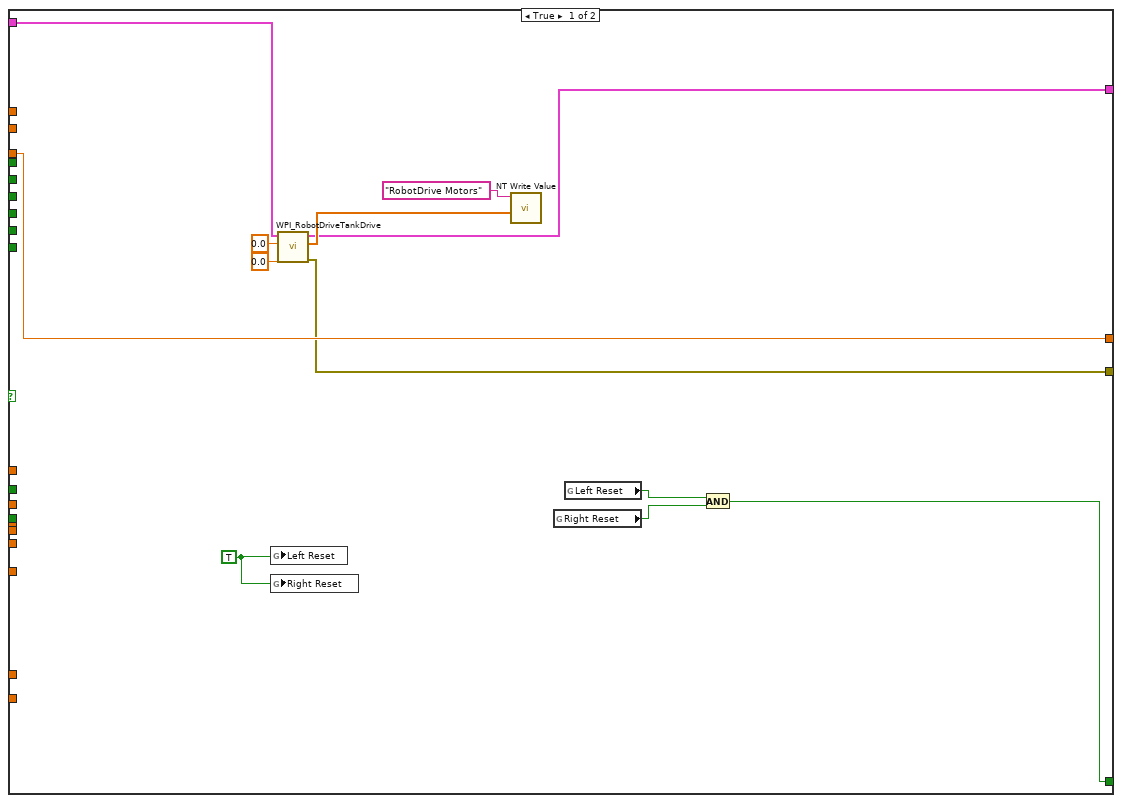
[diagram p14: hidden frame]
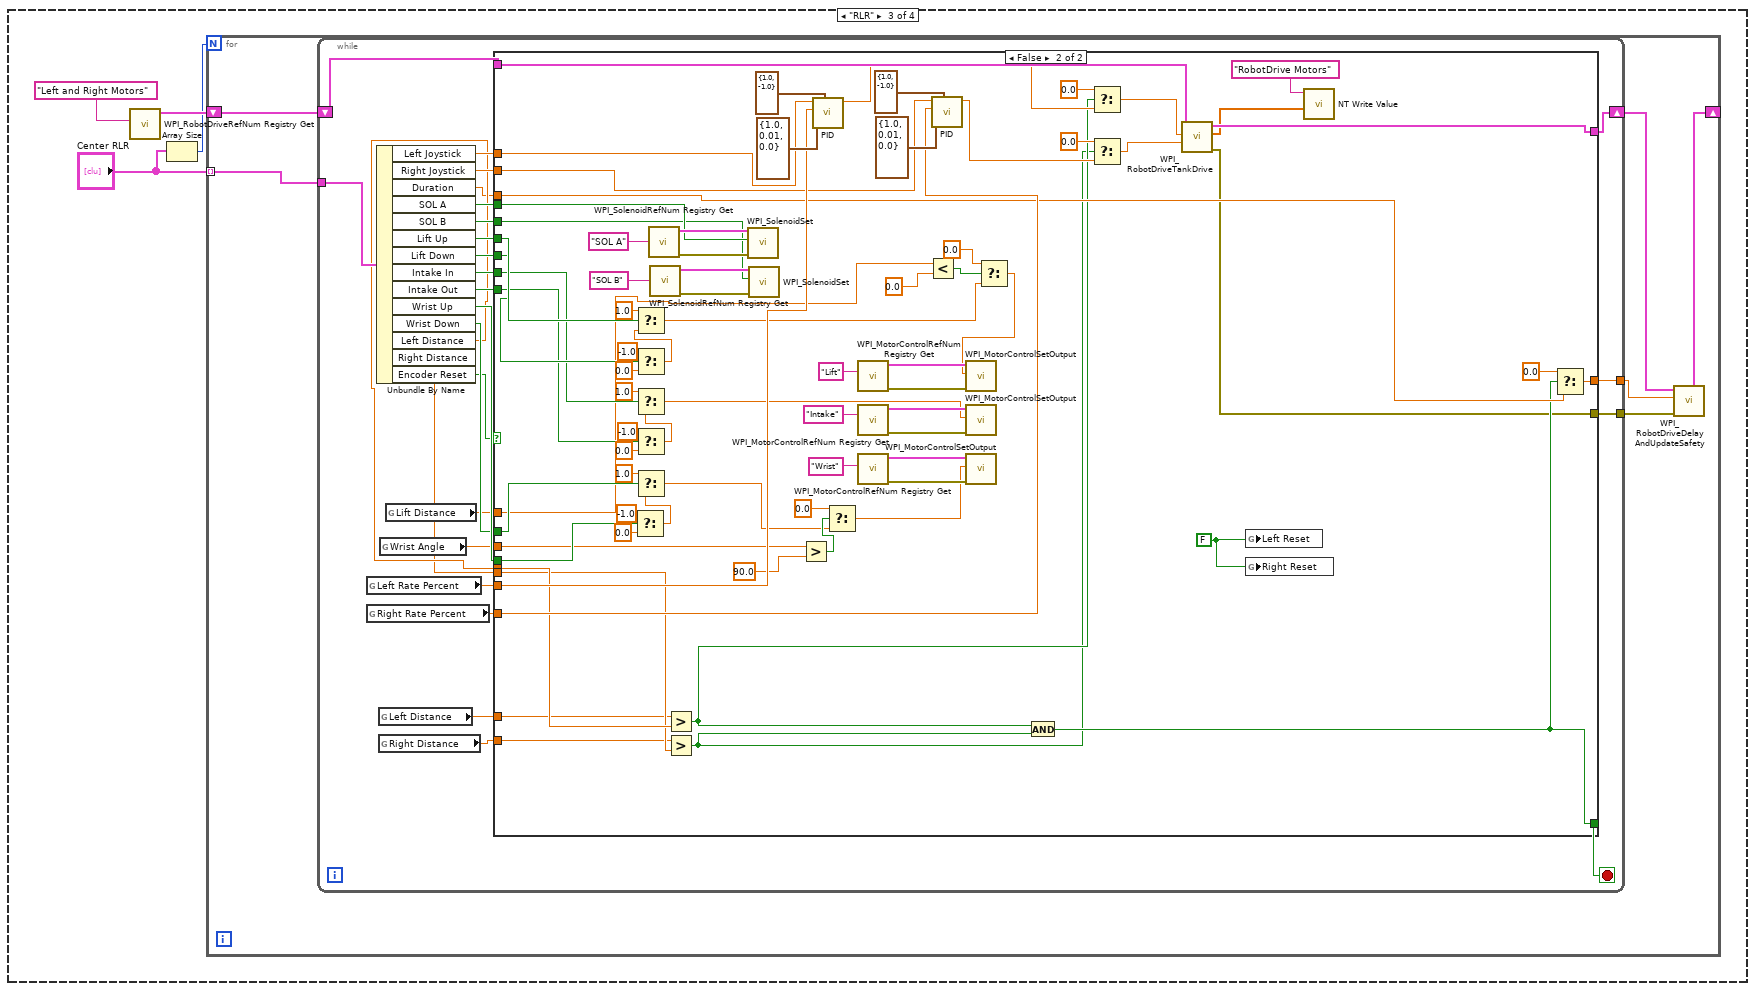
[diagram p15: hidden frame]
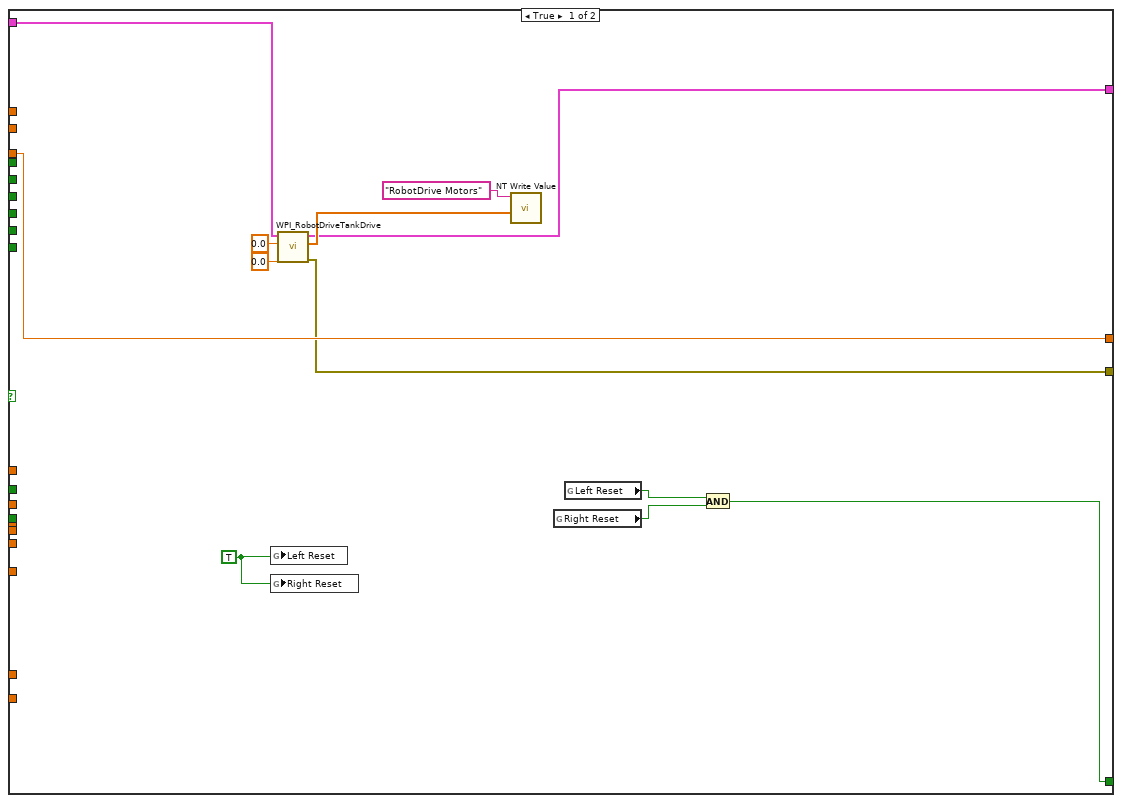
[diagram p16: hidden frame]
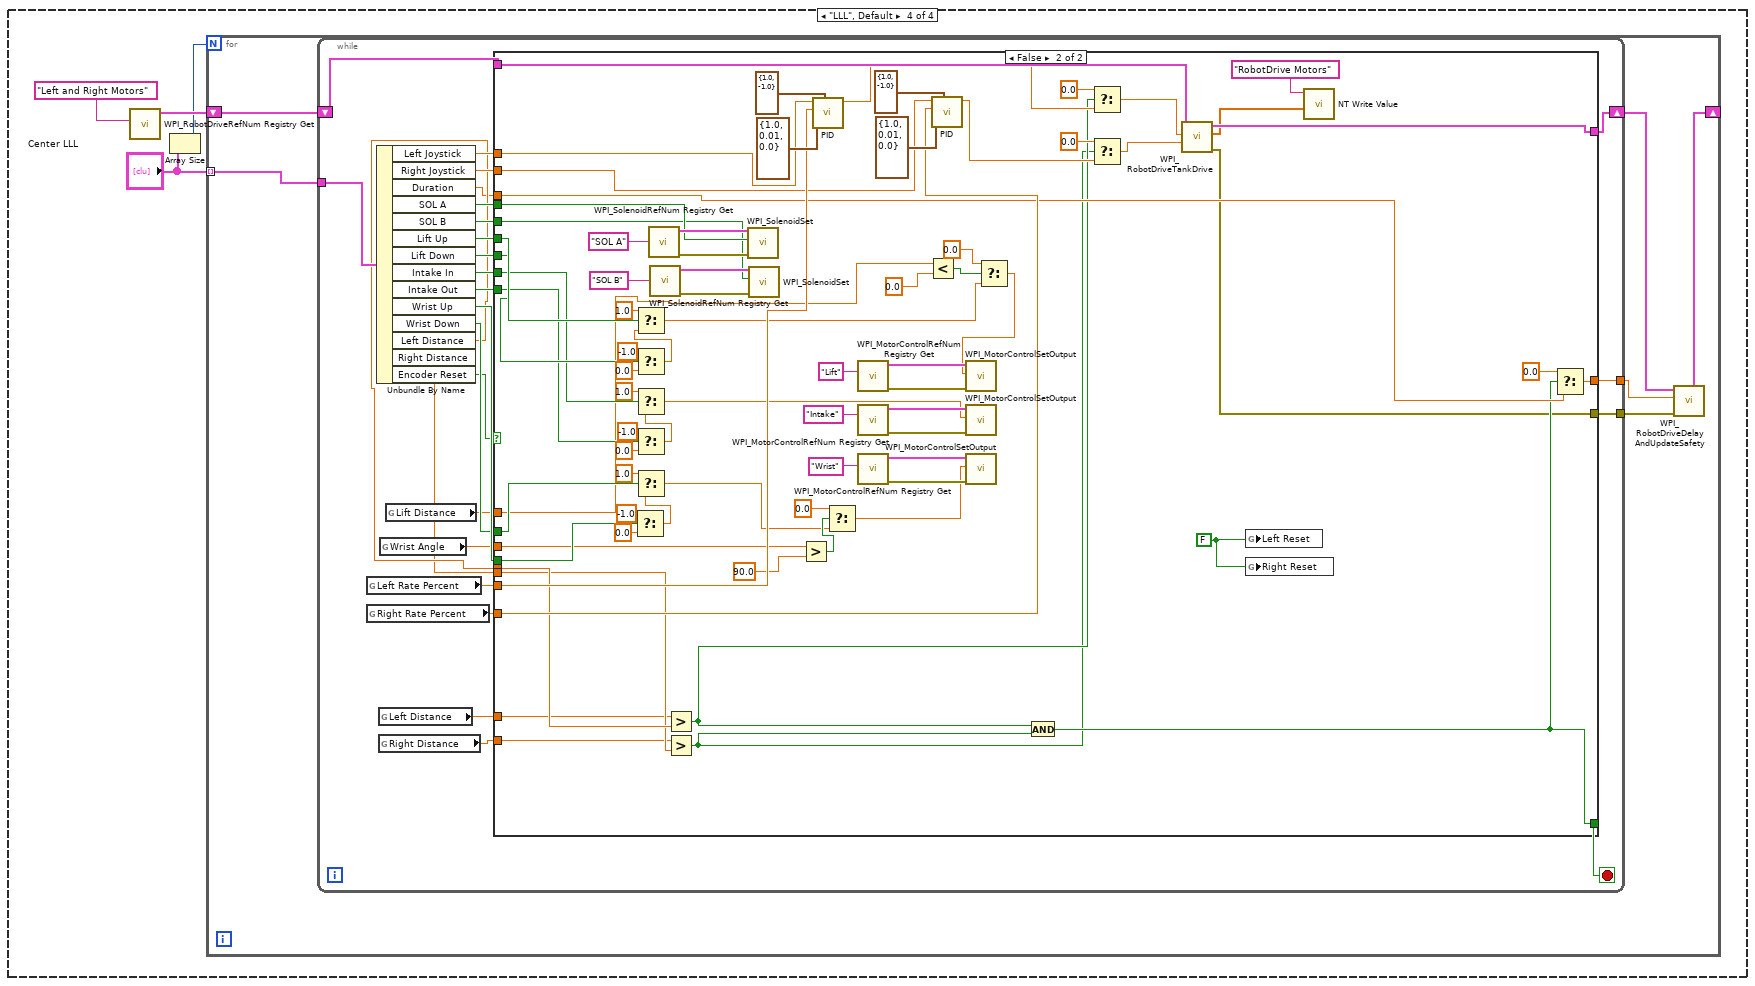
[diagram p17: hidden frame]
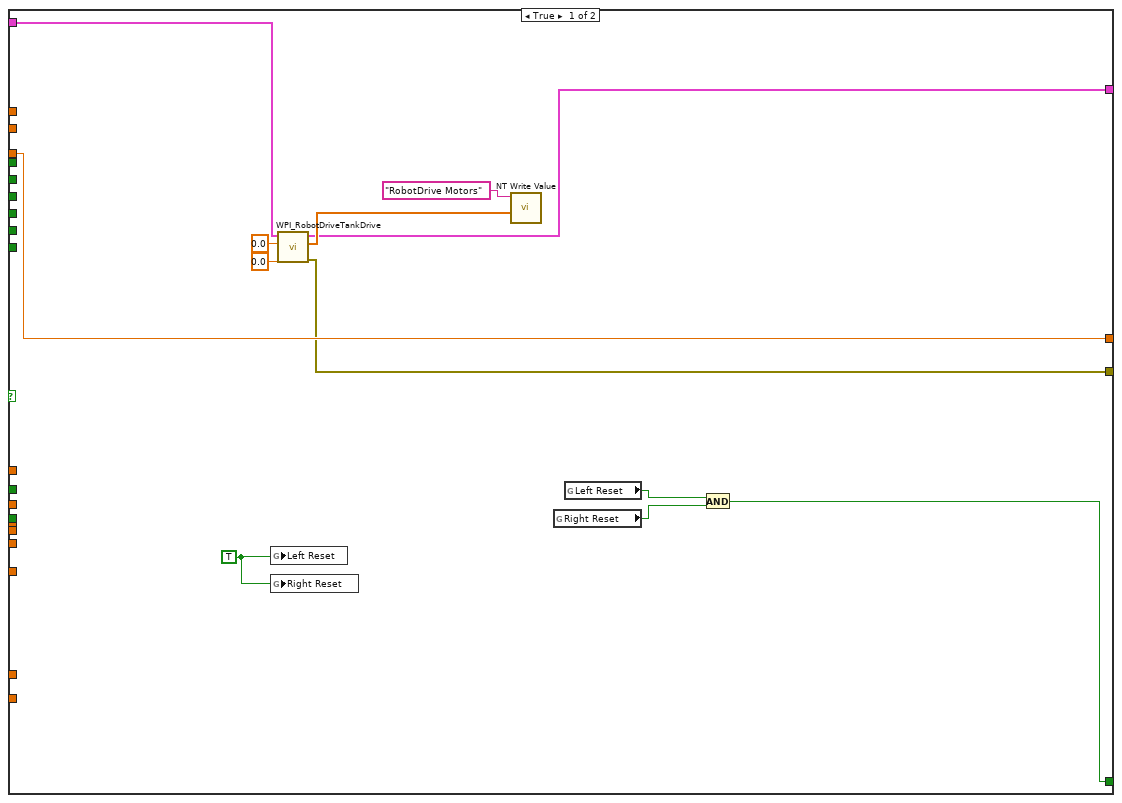
[diagram p18: hidden frame]
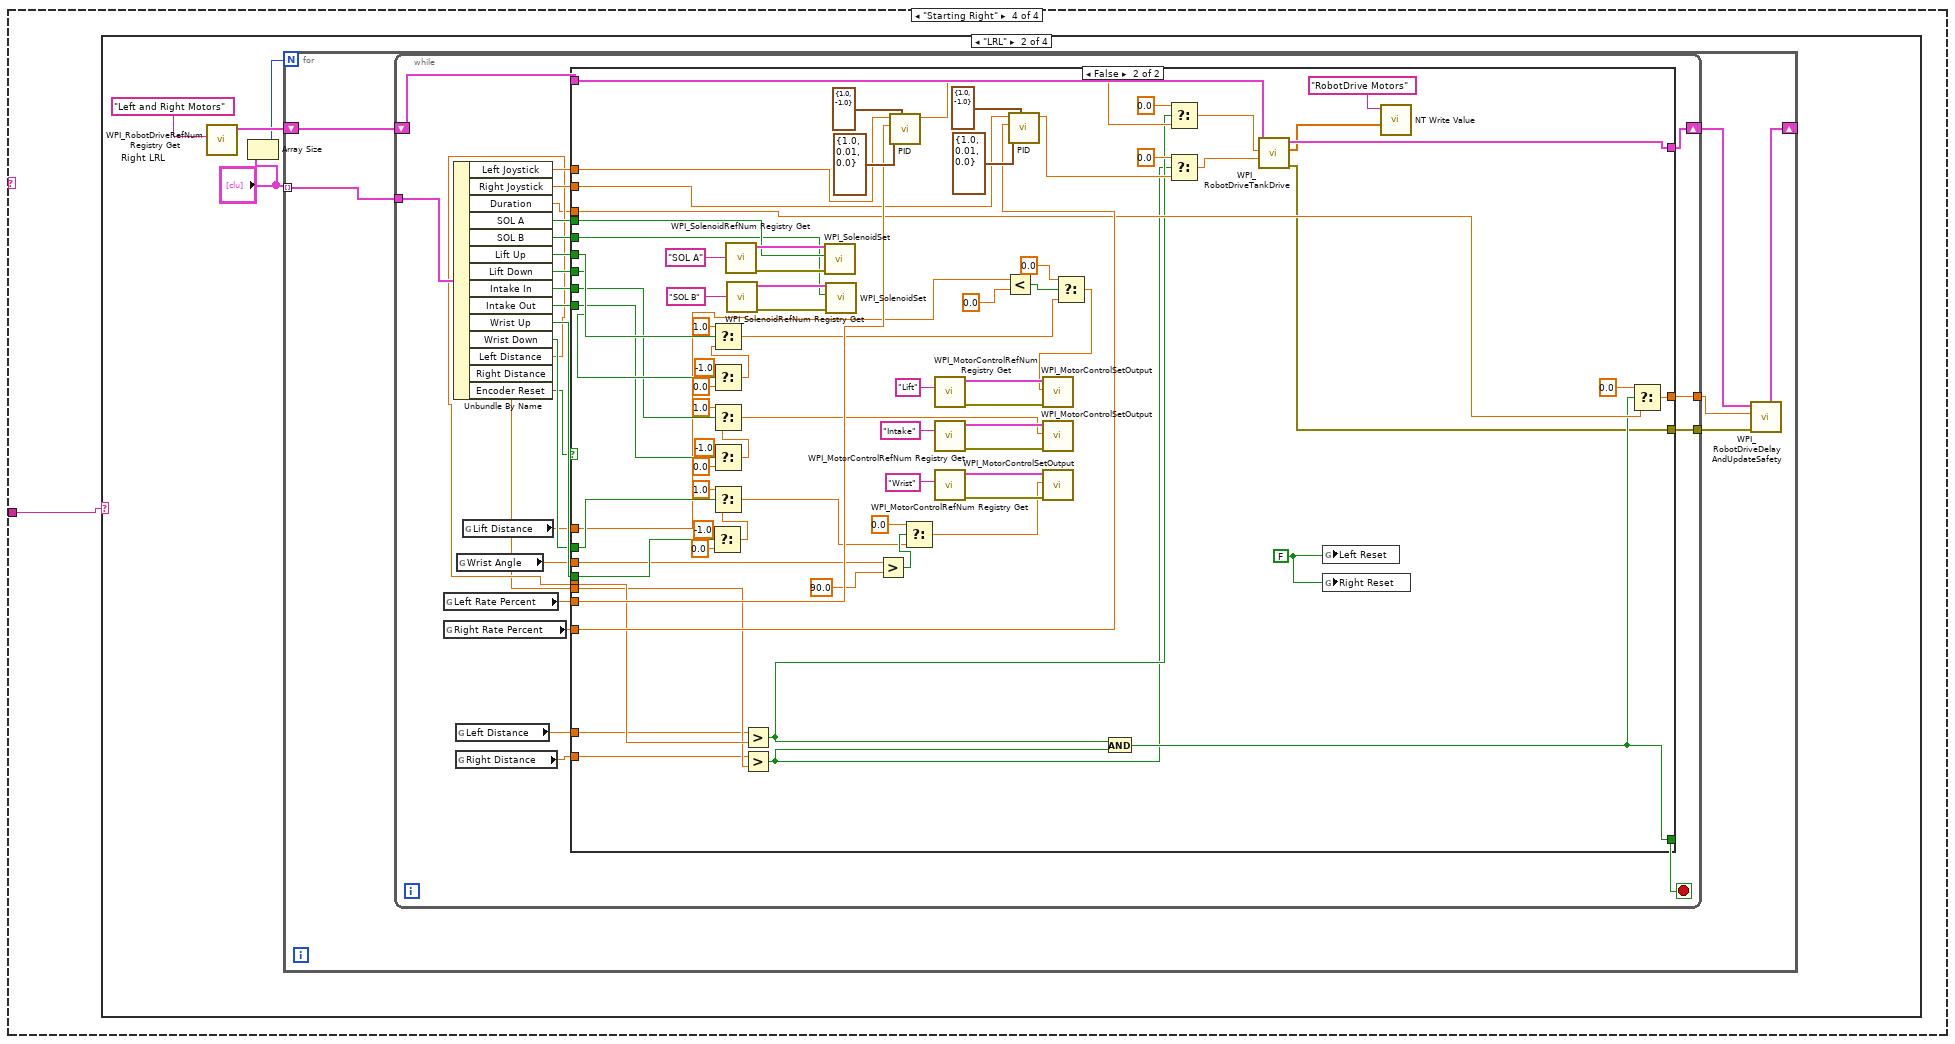
[diagram p19: hidden frame]
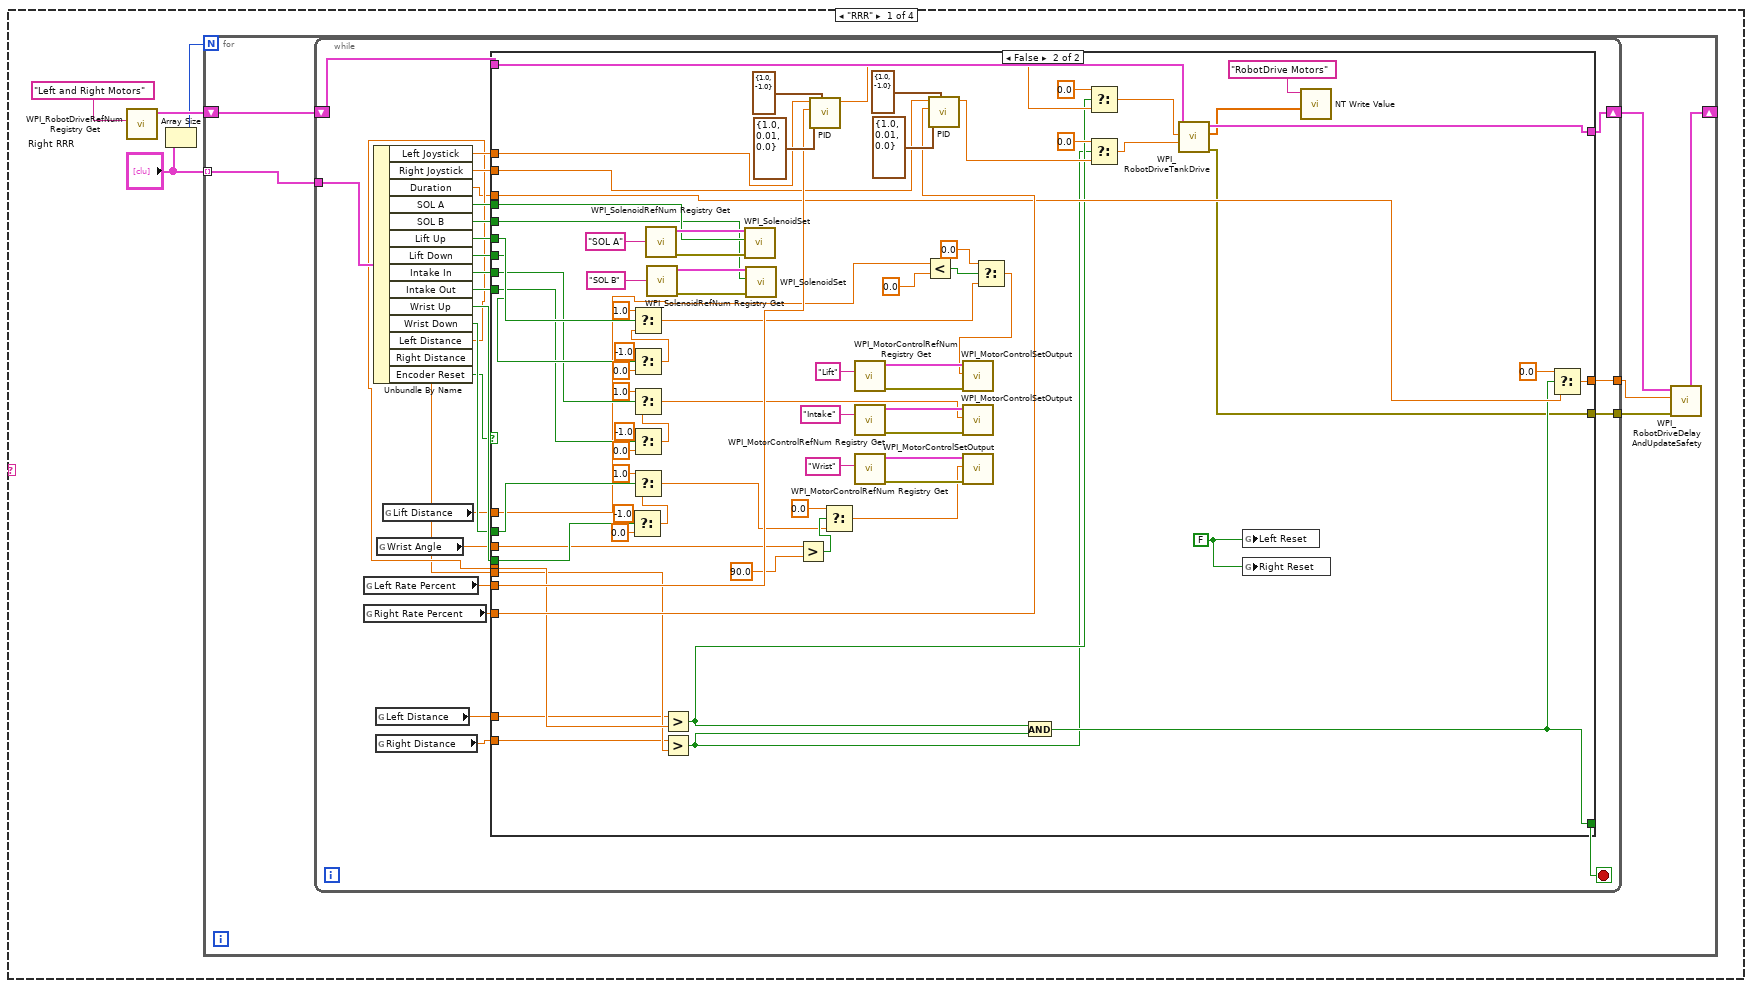
[diagram p20: hidden frame]
diagram:
  (unwired) "This function is run in parallel when the autonomous period begins. It will be terminated automatically when the period ends.\n\nNote that all Driver Station inputs are automatically latched and will not change once auto begins."
  # "This tells you the autonomous selected\nfrom the dashboard"
  # "Every 20ms, report that we are running autonomous\ncode. Loop will abort the same time as the VI."
  # "This gives you the joystick value\nthat is often the throttle"
  # "Use time and/or sensors to control how the robot drives."
  # "This tells you the driver position\nand alliance color"
  n1 = call <vilib>:"WPI_DriverStationGet Alliance Info.vi"() -> ()  [unwired: 12 out]
  n2 = call <vilib>:"WPI_DriverStationGame Specific Data.vi"() -> ("Game Specific Data"=w3:string)  [unwired: 11 in]
  n3 = while {
    stop <- FALSE stop-if-true
    n4 = call <vilib>:"WPI_DriverStationReport Robot Code State.vi"("Autonomous"=TRUE) -> ()  [unwired: 10 in, 1 out]
    n5 = Wait (ms)(milliseconds to wait=u32 20) -> ()  [unwired: 1 out]
  }
  n6 = call <vilib>:"WPI_JoystickRefNum Registry Get.vi"("refnum name"="Left Joystick") -> ("JoystickDevRef"=w14:T3)  [unwired: 1 in, 9 out]
  n7 = call <vilib>:"WPI_JoystickRefNum Registry Get.vi"("refnum name"="Right Joystick") -> ("JoystickDevRef"=w8:T3)  [unwired: 1 in, 9 out]
  n8 = String Subset(string=w3, length (rest)=1 ("length (rest)")) -> (substring=w1:string)  [unwired: 1 in]
  n9 = call <vilib>:"WPI_JoystickGetValues.vi"("JoystickDevRef"=w14) -> ("Axes"=w7:dbl[])  [unwired: 6 in, 4 out]
  n10 = call <vilib>:"WPI_JoystickGetValues.vi"("JoystickDevRef"=w8) -> ("Axes"=w4:dbl[])  [unwired: 6 in, 4 out]
  n11 = call-poly <vilib>:"NT Read Value.vi"("Name"="Auto Selector") -> ("String"=w11:string)  [unwired: 9 in, 1 out]
  n12 = Index Array(array=w4, index=2) -> ()  [unwired: 1 out]
  n13 = call-poly <vilib>:"NT Write Value.vi"("Numeric Array"=w7, "Name"="Left Joystick/Axes") -> ()  [unwired: 9 in, 1 out]
  n14 = Index Array(array=w7, index=2) -> ()  [unwired: 1 out]
  n15 = call-poly <vilib>:"NT Write Value.vi"("Numeric Array"=w4, "Name"="Right Joystick/Axes") -> ()  [unwired: 9 in, 1 out]
  n16 = case shown="Default" w11 {
    tunnel: w1 -> [_ w140 w645 w1150]
    frame Default {
      n17 = Array Size(array="Testing") -> (size(s)=w20:i32)
      n18 = call <vilib>:"WPI_RobotDriveRefNum Registry Get.vi"("refnum name"="Left and Right Motors") -> ("RobotDriveDevRef"=w21:T6)  [unwired: 1 in, 9 out]
      n19 = for {
        N: w20 -> [_]
        shift-right: [w29] -> _
        shift-left: w21 -> [w28]
        tunnel: "Testing" -> [w27] mode=indexing
        i -> [w23]
        n20 = global write "Robot Global Data.vi" "Array Step"(w23) -> ()
        n21 = while {
          shift-right: [w57] -> w25
          shift-left: w28 -> [w56]
          tunnel: w27 -> [w53]
          tunnel: [w34] -> w26
          tunnel: [w37] -> w24
          stop <- w38 stop-if-true
          n22 = global read "Robot Global Data.vi" "Right Distance"() -> (w41:dbl)
          n23 = global read "Robot Global Data.vi" "Lift Distance"() -> (w32:dbl)
          n24 = global read "Robot Global Data.vi" "Left Distance"() -> (w40:dbl)
          n25 = global read "Robot Global Data.vi" "Wrist Angle"() -> (w35:dbl)
          n26 = global read "Robot Global Data.vi" "Left Rate"() -> (w55:dbl)
          n27 = global read "Robot Global Data.vi" "Right Rate"() -> (w54:dbl)
          n28 = Unbundle By Name(w53) -> ("Left In/s"=w52:dbl, "Right In/s"=w51:dbl, "Duration"=w39:dbl, "SOL A"=w50:bool, "SOL B"=w49:bool, "Lift Up"=w48:bool, "Lift Down"=w47:bool, "Intake In"=w46:bool, "Intake Out"=w45:bool, "Wrist Up"=w44:bool, "Wrist Down"=w43:bool, "Left Distance"=w33:dbl, "Right Distance"=w42:dbl, "Encoder Reset"=w36:bool, "Lift Target"=w31:dbl, "Wrist Target"=w30:dbl)
          n29 = case shown="False" w36 {
            tunnel: [w63 w139] -> w57
            tunnel: w56 -> [w64 w138]
            tunnel: w55 -> [_ _]
            tunnel: w54 -> [_ _]
            tunnel: w52 -> [_ w82]
            tunnel: w51 -> [_ w83]
            tunnel: w50 -> [_ w121]
            tunnel: w49 -> [_ w120]
            tunnel: w48 -> [_ w95]
            tunnel: w47 -> [_ w94]
            tunnel: w46 -> [_ w93]
            tunnel: w45 -> [_ w92]
            tunnel: w44 -> [_ w90]
            tunnel: w43 -> [_ w91]
            tunnel: w33 -> [_ w87]
            tunnel: w42 -> [_ w119]
            tunnel: w41 -> [_ w118]
            tunnel: w40 -> [_ w117]
            tunnel: w39 -> [w69 w115]
            tunnel: [w69 w84] -> w34
            tunnel: [w58 w86] -> w38
            tunnel: [w62 w114] -> w37
            tunnel: w35 -> [_ w75]
            tunnel: w32 -> [_ w76]
            tunnel: w31 -> [_ w81]
            tunnel: w30 -> [_ w74]
            frame True {
              w61 = TRUE ("Left Reset")
              n30 = global write "Robot Global Data.vi" "Left Reset"(w61) -> ()
              n31 = global write "Robot Global Data.vi" "Right Reset"(w61) -> ()
              n32 = call <vilib>:"WPI_RobotDriveTankDrive.vi"("Right axis value"=0.0, "Left axis value"=0.0, "RobotDriveDevRef"=w64) -> ("error out"=w62:errorcluster, "Motor Values"=w67:dbl[], "RobotDriveDevRef"=w63:T6)  [unwired: 6 in]
              n33 = call-poly <vilib>:"NT Write Value.vi"("Numeric Array"=w67, "Name"="RobotDrive Motors") -> ()  [unwired: 9 in, 1 out]
              n34 = global read "Robot Global Data.vi" "Right Reset"() -> (w59:bool)
              n35 = global read "Robot Global Data.vi" "Left Reset"() -> (w60:bool)
              n36 = And(x=w60, y=w59) -> (x .and. y?=w58:bool)
            }
            frame False {
              w109 = FALSE ("Left Reset")
              n37 = Select(t=-1.0, s=w90, f=0.0) -> (s? t:f=w99:dbl)
              n38 = Select(t=-1.0, s=w94, f=0.0) -> (s? t:f=w97:dbl)
              n39 = Select(t=1.0, s=w95, f=w97) -> (s? t:f=w79:dbl)
              n40 = Select(t=-1.0, s=w92, f=0.0) -> (s? t:f=w98:dbl)
              n41 = Select(t=1.0, s=w93, f=w98) -> (s? t:f=w96:dbl)
              n42 = Select(t=1.0, s=w91, f=w99) -> (s? t:f=w72:dbl)
              n43 = call <vilib>:"WPI_SolenoidRefNum Registry Get.vi"("refnum name"="SOL A") -> ("error out"=w134:errorcluster, "SolenoidDevRef"=w135:T12)  [unwired: 9 in]
              n44 = call <vilib>:"WPI_SolenoidRefNum Registry Get.vi"("refnum name"="SOL B") -> ("error out"=w131:errorcluster, "SolenoidDevRef"=w132:T12)  [unwired: 9 in]
              n45 = Greater Or Equal?(x=w75, y=w74) -> (x >= y?=w71:bool)
              n46 = Greater Or Equal?(x=w76, y=w81) -> (x >= y?=w77:bool)
              n47 = Greater Or Equal?(x=w117, y=w87) -> (x >= y?=w111:bool)
              n48 = Greater Or Equal?(x=w118, y=w119) -> (x >= y?=w110:bool)
              n49 = call-poly <vilib>:"WPI_SolenoidSet.vi"("error in (no error)"=w134, "Value"=w121, "SolenoidDevRef"=w135) -> ()  [unwired: 7 in, 2 out]
              n50 = call-poly <vilib>:"WPI_SolenoidSet.vi"("error in (no error)"=w131, "Value"=w120, "SolenoidDevRef"=w132) -> ()  [unwired: 7 in, 2 out]
              n51 = Select(t=0.0, s=w71, f=w72) -> (s? t:f=w70:dbl)
              n52 = Select(t=0.0, s=w77, f=w79) -> (s? t:f=w78:dbl)
              n53 = call <vilib>:"WPI_MotorControlRefNum Registry Get.vi"("refnum name"="Lift") -> ("error out"=w129:errorcluster, "MotorControlDevRef"=w130:T7)  [unwired: 9 in]
              n54 = call <vilib>:"WPI_MotorControlRefNum Registry Get.vi"("refnum name"="Intake") -> ("error out"=w127:errorcluster, "MotorControlDevRef"=w128:T7)  [unwired: 9 in]
              n55 = call <vilib>:"WPI_MotorControlRefNum Registry Get.vi"("refnum name"="Wrist") -> ("error out"=w125:errorcluster, "MotorControlDevRef"=w126:T7)  [unwired: 9 in]
              n56 = call <vilib>:"WPI_MotorControlSetOutput.vi"("error in (no error)"=w129, "Output"=w78, "MotorControlDevRef"=w130) -> ()  [unwired: 6 in, 3 out]
              n57 = call <vilib>:"WPI_MotorControlSetOutput.vi"("error in (no error)"=w127, "Output"=w96, "MotorControlDevRef"=w128) -> ()  [unwired: 6 in, 3 out]
              n58 = call <vilib>:"WPI_MotorControlSetOutput.vi"("error in (no error)"=w125, "Output"=w70, "MotorControlDevRef"=w126) -> ()  [unwired: 6 in, 3 out]
              n59 = And(x=w111, y=w110) -> (x .and. y?=w86:bool)
              n60 = Select(t=0.0, s=w111, f=w83) -> (s? t:f=w89:dbl)
              n61 = Select(t=0.0, s=w110, f=w82) -> (s? t:f=w88:dbl)
              n62 = call <vilib>:"WPI_RobotDriveTankDrive.vi"("Right axis value"=w88, "Left axis value"=w89, "RobotDriveDevRef"=w138) -> ("error out"=w114:errorcluster, "Motor Values"=w85:dbl[], "RobotDriveDevRef"=w139:T6)  [unwired: 6 in]
              n63 = global write "Robot Global Data.vi" "Left Reset"(w109) -> ()
              n64 = global write "Robot Global Data.vi" "Right Reset"(w109) -> ()
              n65 = call-poly <vilib>:"NT Write Value.vi"("Numeric Array"=w85, "Name"="RobotDrive Motors") -> ()  [unwired: 9 in, 1 out]
              n66 = Select(t=0.0, s=w86, f=w115) -> (s? t:f=w84:dbl)
            }
          }
        }
        n67 = call <vilib>:"WPI_RobotDriveDelayAndUpdateSafety.vi"("error in (no error)"=w24, "Delay (s)"=w26, "RobotDriveDevRef"=w25) -> ("RobotDriveDevRef 2"=w29:T6)  [unwired: 7 in, 1 out]
      }
    }
    frame "Starting Left" {
      n68 = case shown="\"LRL\"" w140 {
        frame "RRR" {
          n69 = call <vilib>:"WPI_RobotDriveRefNum Registry Get.vi"("refnum name"="Left and Right Motors") -> ("RobotDriveDevRef"=w143:T6)  [unwired: 1 in, 9 out]
          n70 = Array Size(array="Left RRR") -> (size(s)=w141:i32)
          n71 = for {
            N: w141 -> [_]
            shift-right: [w148] -> _
            shift-left: w143 -> [w149]
            tunnel: "Left RRR" -> [w147] mode=indexing
            n72 = while {
              shift-right: [w176] -> w150
              shift-left: w149 -> [w175]
              tunnel: w147 -> [w172]
              tunnel: [w156] -> w146
              tunnel: [w154] -> w145
              stop <- w155 stop-if-true
              n73 = global read "Robot Global Data.vi" "Left Rate Percent"() -> (w174:dbl)
              n74 = global read "Robot Global Data.vi" "Right Rate Percent"() -> (w173:dbl)
              n75 = Unbundle By Name(w172) -> ("Left Joystick"=w171:dbl, "Right Joystick"=w170:dbl, "Duration"=w157:dbl, "SOL A"=w169:bool, "SOL B"=w168:bool, "Lift Up"=w167:bool, "Lift Down"=w166:bool, "Intake In"=w165:bool, "Intake Out"=w164:bool, "Wrist Up"=w163:bool, "Wrist Down"=w162:bool, "Left Distance"=w161:dbl, "Right Distance"=w160:dbl, "Encoder Reset"=w153:bool)
              n76 = global read "Robot Global Data.vi" "Left Distance"() -> (w158:dbl)
              n77 = global read "Robot Global Data.vi" "Right Distance"() -> (w159:dbl)
              n78 = global read "Robot Global Data.vi" "Wrist Angle"() -> (w152:dbl)
              n79 = global read "Robot Global Data.vi" "Lift Distance"() -> (w151:dbl)
              n80 = case shown="False" w153 {
                tunnel: [w182 w266] -> w176
                tunnel: w175 -> [w183 w265]
                tunnel: w174 -> [_ w243]
                tunnel: w173 -> [_ w242]
                tunnel: w171 -> [_ w241]
                tunnel: w170 -> [_ w240]
                tunnel: w169 -> [_ w239]
                tunnel: w168 -> [_ w238]
                tunnel: w167 -> [_ w208]
                tunnel: w166 -> [_ w207]
                tunnel: w165 -> [_ w206]
                tunnel: w164 -> [_ w205]
                tunnel: w163 -> [_ w203]
                tunnel: w162 -> [_ w204]
                tunnel: w161 -> [_ w237]
                tunnel: w160 -> [_ w236]
                tunnel: w159 -> [_ w235]
                tunnel: w158 -> [_ w234]
                tunnel: w157 -> [w188 w232]
                tunnel: [w188 w231] -> w156
                tunnel: [w177 w230] -> w155
                tunnel: [w181 w229] -> w154
                tunnel: w152 -> [_ w195]
                tunnel: w151 -> [_ w189]
                frame True {
                  w180 = TRUE ("Left Reset")
                  n81 = global write "Robot Global Data.vi" "Left Reset"(w180) -> ()
                  n82 = global write "Robot Global Data.vi" "Right Reset"(w180) -> ()
                  n83 = call <vilib>:"WPI_RobotDriveTankDrive.vi"("Right axis value"=0.0, "Left axis value"=0.0, "RobotDriveDevRef"=w183) -> ("error out"=w181:errorcluster, "Motor Values"=w186:dbl[], "RobotDriveDevRef"=w182:T6)  [unwired: 6 in]
                  n84 = call-poly <vilib>:"NT Write Value.vi"("Numeric Array"=w186, "Name"="RobotDrive Motors") -> ()  [unwired: 9 in, 1 out]
                  n85 = global read "Robot Global Data.vi" "Right Reset"() -> (w178:bool)
                  n86 = global read "Robot Global Data.vi" "Left Reset"() -> (w179:bool)
                  n87 = And(x=w179, y=w178) -> (x .and. y?=w177:bool)
                }
                frame False {
                  w222 = FALSE ("Left Reset")
                  n88 = Select(t=-1.0, s=w203, f=0.0) -> (s? t:f=w212:dbl)
                  n89 = Select(t=-1.0, s=w207, f=0.0) -> (s? t:f=w210:dbl)
                  n90 = Select(t=1.0, s=w208, f=w210) -> (s? t:f=w191:dbl)
                  n91 = Select(t=-1.0, s=w205, f=0.0) -> (s? t:f=w211:dbl)
                  n92 = Select(t=1.0, s=w206, f=w211) -> (s? t:f=w209:dbl)
                  n93 = Select(t=1.0, s=w204, f=w212) -> (s? t:f=w198:dbl)
                  n94 = call <vilib>:"WPI_SolenoidRefNum Registry Get.vi"("refnum name"="SOL A") -> ("error out"=w260:errorcluster, "SolenoidDevRef"=w261:T12)  [unwired: 9 in]
                  n95 = call <vilib>:"WPI_SolenoidRefNum Registry Get.vi"("refnum name"="SOL B") -> ("error out"=w257:errorcluster, "SolenoidDevRef"=w258:T12)  [unwired: 9 in]
                  n96 = Greater?(x=w234, y=w237) -> (0:w224:bool)
                  n97 = Greater?(x=w235, y=w236) -> (0:w223:bool)
                  n98 = call-poly <vilib>:"WPI_SolenoidSet.vi"("error in (no error)"=w260, "Value"=w239, "SolenoidDevRef"=w261) -> ()  [unwired: 7 in, 2 out]
                  n99 = call-poly <vilib>:"WPI_SolenoidSet.vi"("error in (no error)"=w257, "Value"=w238, "SolenoidDevRef"=w258) -> ()  [unwired: 7 in, 2 out]
                  n100 = Greater?(x=w195, y=90.0) -> (0:w199:bool)
                  n101 = call-poly <vilib>:"PID.vi"("output range"=cluster{"output high":dbl, "output low":dbl} {"output high"=1.0, "output low"=-1.0}, "PID gains"=T5 {"proportional gain (Kc)"=1.0, "integral time (Ti, min)"=0.01, "derivative time (Td, min)"=0.0}, "process variable"=w243, "setpoint"=w241) -> ("output"=w225:dbl)  [unwired: 6 in, 1 out]
                  n102 = Select(t=0.0, s=w199, f=w198) -> (s? t:f=w196:dbl)
                  n103 = call <vilib>:"WPI_MotorControlRefNum Registry Get.vi"("refnum name"="Lift") -> ("error out"=w255:errorcluster, "MotorControlDevRef"=w256:T7)  [unwired: 9 in]
                  n104 = call <vilib>:"WPI_MotorControlRefNum Registry Get.vi"("refnum name"="Intake") -> ("error out"=w253:errorcluster, "MotorControlDevRef"=w254:T7)  [unwired: 9 in]
                  n105 = call <vilib>:"WPI_MotorControlRefNum Registry Get.vi"("refnum name"="Wrist") -> ("error out"=w251:errorcluster, "MotorControlDevRef"=w252:T7)  [unwired: 9 in]
                  n106 = Less?(x=w189, y=0.0) -> (x < y?=w193:bool)
                  n107 = call-poly <vilib>:"PID.vi"("output range"=cluster{"output high":dbl, "output low":dbl} {"output high"=1.0, "output low"=-1.0}, "PID gains"=T5 {"proportional gain (Kc)"=1.0, "integral time (Ti, min)"=0.01, "derivative time (Td, min)"=0.0}, "process variable"=w242, "setpoint"=w240) -> ("output"=w226:dbl)  [unwired: 6 in, 1 out]
                  n108 = call <vilib>:"WPI_MotorControlSetOutput.vi"("error in (no error)"=w253, "Output"=w209, "MotorControlDevRef"=w254) -> ()  [unwired: 6 in, 3 out]
                  n109 = call <vilib>:"WPI_MotorControlSetOutput.vi"("error in (no error)"=w251, "Output"=w196, "MotorControlDevRef"=w252) -> ()  [unwired: 6 in, 3 out]
                  n110 = Select(t=0.0, s=w193, f=w191) -> (s? t:f=w190:dbl)
                  n111 = call <vilib>:"WPI_MotorControlSetOutput.vi"("error in (no error)"=w255, "Output"=w190, "MotorControlDevRef"=w256) -> ()  [unwired: 6 in, 3 out]
                  n112 = And(x=w224, y=w223) -> (x .and. y?=w230:bool)
                  n113 = Select(t=0.0, s=w224, f=w225) -> (s? t:f=w202:dbl)
                  n114 = Select(t=0.0, s=w223, f=w226) -> (s? t:f=w201:dbl)
                  n115 = call <vilib>:"WPI_RobotDriveTankDrive.vi"("Right axis value"=w201, "Left axis value"=w202, "RobotDriveDevRef"=w265) -> ("error out"=w229:errorcluster, "Motor Values"=w263:dbl[], "RobotDriveDevRef"=w266:T6)  [unwired: 6 in]
                  n116 = global write "Robot Global Data.vi" "Left Reset"(w222) -> ()
                  n117 = global write "Robot Global Data.vi" "Right Reset"(w222) -> ()
                  n118 = call-poly <vilib>:"NT Write Value.vi"("Numeric Array"=w263, "Name"="RobotDrive Motors") -> ()  [unwired: 9 in, 1 out]
                  n119 = Select(t=0.0, s=w230, f=w232) -> (s? t:f=w231:dbl)
                }
              }
            }
            n120 = call <vilib>:"WPI_RobotDriveDelayAndUpdateSafety.vi"("error in (no error)"=w145, "Delay (s)"=w146, "RobotDriveDevRef"=w150) -> ("RobotDriveDevRef 2"=w148:T6)  [unwired: 7 in, 1 out]
          }
        }
        frame "LRL" {
          n121 = call <vilib>:"WPI_RobotDriveRefNum Registry Get.vi"("refnum name"="Left and Right Motors") -> ("RobotDriveDevRef"=w269:T6)  [unwired: 1 in, 9 out]
          n122 = Array Size(array="Left LRL") -> (size(s)=w267:i32)
          n123 = for {
            N: w267 -> [_]
            shift-right: [w274] -> _
            shift-left: w269 -> [w275]
            tunnel: "Left LRL" -> [w273] mode=indexing
            n124 = while {
              shift-right: [w302] -> w276
              shift-left: w275 -> [w301]
              tunnel: w273 -> [w298]
              tunnel: [w282] -> w272
              tunnel: [w280] -> w271
              stop <- w281 stop-if-true
              n125 = global read "Robot Global Data.vi" "Left Rate Percent"() -> (w300:dbl)
              n126 = global read "Robot Global Data.vi" "Right Rate Percent"() -> (w299:dbl)
              n127 = Unbundle By Name(w298) -> ("Left Joystick"=w297:dbl, "Right Joystick"=w296:dbl, "Duration"=w283:dbl, "SOL A"=w295:bool, "SOL B"=w294:bool, "Lift Up"=w293:bool, "Lift Down"=w292:bool, "Intake In"=w291:bool, "Intake Out"=w290:bool, "Wrist Up"=w289:bool, "Wrist Down"=w288:bool, "Left Distance"=w287:dbl, "Right Distance"=w286:dbl, "Encoder Reset"=w279:bool)
              n128 = global read "Robot Global Data.vi" "Left Distance"() -> (w284:dbl)
              n129 = global read "Robot Global Data.vi" "Right Distance"() -> (w285:dbl)
              n130 = global read "Robot Global Data.vi" "Wrist Angle"() -> (w278:dbl)
              n131 = global read "Robot Global Data.vi" "Lift Distance"() -> (w277:dbl)
              n132 = case shown="False" w279 {
                tunnel: [w308 w392] -> w302
                tunnel: w301 -> [w309 w391]
                tunnel: w300 -> [_ w319]
                tunnel: w299 -> [_ w320]
                tunnel: w297 -> [_ w318]
                tunnel: w296 -> [_ w317]
                tunnel: w295 -> [_ w373]
                tunnel: w294 -> [_ w372]
                tunnel: w293 -> [_ w344]
                tunnel: w292 -> [_ w343]
                tunnel: w291 -> [_ w342]
                tunnel: w290 -> [_ w341]
                tunnel: w289 -> [_ w339]
                tunnel: w288 -> [_ w340]
                tunnel: w287 -> [_ w371]
                tunnel: w286 -> [_ w370]
                tunnel: w285 -> [_ w369]
                tunnel: w284 -> [_ w368]
                tunnel: w283 -> [w314 w366]
                tunnel: [w314 w365] -> w282
                tunnel: [w303 w364] -> w281
                tunnel: [w307 w363] -> w280
                tunnel: w278 -> [_ w331]
                tunnel: w277 -> [_ w325]
                frame True {
                  w306 = TRUE ("Left Reset")
                  n133 = global write "Robot Global Data.vi" "Left Reset"(w306) -> ()
                  n134 = global write "Robot Global Data.vi" "Right Reset"(w306) -> ()
                  n135 = call <vilib>:"WPI_RobotDriveTankDrive.vi"("Right axis value"=0.0, "Left axis value"=0.0, "RobotDriveDevRef"=w309) -> ("error out"=w307:errorcluster, "Motor Values"=w312:dbl[], "RobotDriveDevRef"=w308:T6)  [unwired: 6 in]
                  n136 = call-poly <vilib>:"NT Write Value.vi"("Numeric Array"=w312, "Name"="RobotDrive Motors") -> ()  [unwired: 9 in, 1 out]
                  n137 = global read "Robot Global Data.vi" "Right Reset"() -> (w304:bool)
                  n138 = global read "Robot Global Data.vi" "Left Reset"() -> (w305:bool)
                  n139 = And(x=w305, y=w304) -> (x .and. y?=w303:bool)
                }
                frame False {
                  w358 = FALSE ("Left Reset")
                  n140 = Select(t=-1.0, s=w339, f=0.0) -> (s? t:f=w348:dbl)
                  n141 = Select(t=-1.0, s=w343, f=0.0) -> (s? t:f=w346:dbl)
                  n142 = Select(t=1.0, s=w344, f=w346) -> (s? t:f=w327:dbl)
                  n143 = Select(t=-1.0, s=w341, f=0.0) -> (s? t:f=w347:dbl)
                  n144 = Select(t=1.0, s=w342, f=w347) -> (s? t:f=w345:dbl)
                  n145 = Select(t=1.0, s=w340, f=w348) -> (s? t:f=w334:dbl)
                  n146 = call <vilib>:"WPI_SolenoidRefNum Registry Get.vi"("refnum name"="SOL A") -> ("error out"=w386:errorcluster, "SolenoidDevRef"=w387:T12)  [unwired: 9 in]
                  n147 = call <vilib>:"WPI_SolenoidRefNum Registry Get.vi"("refnum name"="SOL B") -> ("error out"=w383:errorcluster, "SolenoidDevRef"=w384:T12)  [unwired: 9 in]
                  n148 = Greater?(x=w368, y=w371) -> (0:w360:bool)
                  n149 = Greater?(x=w369, y=w370) -> (0:w359:bool)
                  n150 = call-poly <vilib>:"PID.vi"("output range"=cluster{"output high":dbl, "output low":dbl} {"output high"=1.0, "output low"=-1.0}, "PID gains"=T5 {"proportional gain (Kc)"=1.0, "integral time (Ti, min)"=0.1, "derivative time (Td, min)"=0.0}, "process variable"=w319, "setpoint"=w318) -> ("output"=w316:dbl)  [unwired: 6 in, 1 out]
                  n151 = call-poly <vilib>:"WPI_SolenoidSet.vi"("error in (no error)"=w386, "Value"=w373, "SolenoidDevRef"=w387) -> ()  [unwired: 7 in, 2 out]
                  n152 = call-poly <vilib>:"WPI_SolenoidSet.vi"("error in (no error)"=w383, "Value"=w372, "SolenoidDevRef"=w384) -> ()  [unwired: 7 in, 2 out]
                  n153 = Greater?(x=w331, y=90.0) -> (0:w335:bool)
                  n154 = global write "Robot Global Data.vi" "Left Rate Percent"(w316) -> ()
                  n155 = Select(t=0.0, s=w335, f=w334) -> (s? t:f=w332:dbl)
                  n156 = call <vilib>:"WPI_MotorControlRefNum Registry Get.vi"("refnum name"="Lift") -> ("error out"=w381:errorcluster, "MotorControlDevRef"=w382:T7)  [unwired: 9 in]
                  n157 = call <vilib>:"WPI_MotorControlRefNum Registry Get.vi"("refnum name"="Intake") -> ("error out"=w379:errorcluster, "MotorControlDevRef"=w380:T7)  [unwired: 9 in]
                  n158 = call <vilib>:"WPI_MotorControlRefNum Registry Get.vi"("refnum name"="Wrist") -> ("error out"=w377:errorcluster, "MotorControlDevRef"=w378:T7)  [unwired: 9 in]
                  n159 = Less?(x=w325, y=0.0) -> (x < y?=w329:bool)
                  n160 = call-poly <vilib>:"PID.vi"("output range"=cluster{"output high":dbl, "output low":dbl} {"output high"=1.0, "output low"=-1.0}, "PID gains"=T5 {"proportional gain (Kc)"=1.0, "integral time (Ti, min)"=0.1, "derivative time (Td, min)"=0.0}, "process variable"=w320, "setpoint"=w317) -> ("output"=w315:dbl)  [unwired: 6 in, 1 out]
                  n161 = call <vilib>:"WPI_MotorControlSetOutput.vi"("error in (no error)"=w379, "Output"=w345, "MotorControlDevRef"=w380) -> ()  [unwired: 6 in, 3 out]
                  n162 = call <vilib>:"WPI_MotorControlSetOutput.vi"("error in (no error)"=w377, "Output"=w332, "MotorControlDevRef"=w378) -> ()  [unwired: 6 in, 3 out]
                  n163 = Select(t=0.0, s=w329, f=w327) -> (s? t:f=w326:dbl)
                  n164 = call <vilib>:"WPI_MotorControlSetOutput.vi"("error in (no error)"=w381, "Output"=w326, "MotorControlDevRef"=w382) -> ()  [unwired: 6 in, 3 out]
                  n165 = And(x=w360, y=w359) -> (x .and. y?=w364:bool)
                  n166 = global write "Robot Global Data.vi" "Right Rate Percent"(w315) -> ()
                  n167 = Select(t=0.0, s=w360, f=w316) -> (s? t:f=w338:dbl)
                  n168 = Select(t=0.0, s=w359, f=w315) -> (s? t:f=w337:dbl)
                  n169 = call <vilib>:"WPI_RobotDriveTankDrive.vi"("Right axis value"=w337, "Left axis value"=w338, "RobotDriveDevRef"=w391) -> ("error out"=w363:errorcluster, "Motor Values"=w389:dbl[], "RobotDriveDevRef"=w392:T6)  [unwired: 6 in]
                  n170 = global write "Robot Global Data.vi" "Left Reset"(w358) -> ()
                  n171 = global write "Robot Global Data.vi" "Right Reset"(w358) -> ()
                  n172 = call-poly <vilib>:"NT Write Value.vi"("Numeric Array"=w389, "Name"="RobotDrive Motors") -> ()  [unwired: 9 in, 1 out]
                  n173 = Select(t=0.0, s=w364, f=w366) -> (s? t:f=w365:dbl)
                }
              }
            }
            n174 = call <vilib>:"WPI_RobotDriveDelayAndUpdateSafety.vi"("error in (no error)"=w271, "Delay (s)"=w272, "RobotDriveDevRef"=w276) -> ("RobotDriveDevRef 2"=w274:T6)  [unwired: 7 in, 1 out]
          }
        }
        frame "RLR" {
          n175 = call <vilib>:"WPI_RobotDriveRefNum Registry Get.vi"("refnum name"="Left and Right Motors") -> ("RobotDriveDevRef"=w395:T6)  [unwired: 1 in, 9 out]
          n176 = Array Size(array="Left RLR") -> (size(s)=w393:i32)
          n177 = for {
            N: w393 -> [_]
            shift-right: [w400] -> _
            shift-left: w395 -> [w401]
            tunnel: "Left RLR" -> [w399] mode=indexing
            n178 = while {
              shift-right: [w428] -> w402
              shift-left: w401 -> [w427]
              tunnel: w399 -> [w424]
              tunnel: [w408] -> w398
              tunnel: [w406] -> w397
              stop <- w407 stop-if-true
              n179 = global read "Robot Global Data.vi" "Left Rate Percent"() -> (w426:dbl)
              n180 = global read "Robot Global Data.vi" "Right Rate Percent"() -> (w425:dbl)
              n181 = Unbundle By Name(w424) -> ("Left Joystick"=w423:dbl, "Right Joystick"=w422:dbl, "Duration"=w409:dbl, "SOL A"=w421:bool, "SOL B"=w420:bool, "Lift Up"=w419:bool, "Lift Down"=w418:bool, "Intake In"=w417:bool, "Intake Out"=w416:bool, "Wrist Up"=w415:bool, "Wrist Down"=w414:bool, "Left Distance"=w413:dbl, "Right Distance"=w412:dbl, "Encoder Reset"=w405:bool)
              n182 = global read "Robot Global Data.vi" "Left Distance"() -> (w410:dbl)
              n183 = global read "Robot Global Data.vi" "Right Distance"() -> (w411:dbl)
              n184 = global read "Robot Global Data.vi" "Wrist Angle"() -> (w404:dbl)
              n185 = global read "Robot Global Data.vi" "Lift Distance"() -> (w403:dbl)
              n186 = case shown="False" w405 {
                tunnel: [w434 w518] -> w428
                tunnel: w427 -> [w435 w517]
                tunnel: w426 -> [_ w495]
                tunnel: w425 -> [_ w494]
                tunnel: w423 -> [_ w493]
                tunnel: w422 -> [_ w492]
                tunnel: w421 -> [_ w491]
                tunnel: w420 -> [_ w490]
                tunnel: w419 -> [_ w460]
                tunnel: w418 -> [_ w459]
                tunnel: w417 -> [_ w458]
                tunnel: w416 -> [_ w457]
                tunnel: w415 -> [_ w455]
                tunnel: w414 -> [_ w456]
                tunnel: w413 -> [_ w489]
                tunnel: w412 -> [_ w488]
                tunnel: w411 -> [_ w487]
                tunnel: w410 -> [_ w486]
                tunnel: w409 -> [w440 w484]
                tunnel: [w440 w483] -> w408
                tunnel: [w429 w482] -> w407
                tunnel: [w433 w481] -> w406
                tunnel: w404 -> [_ w447]
                tunnel: w403 -> [_ w441]
                frame True {
                  w432 = TRUE ("Left Reset")
                  n187 = global write "Robot Global Data.vi" "Left Reset"(w432) -> ()
                  n188 = global write "Robot Global Data.vi" "Right Reset"(w432) -> ()
                  n189 = call <vilib>:"WPI_RobotDriveTankDrive.vi"("Right axis value"=0.0, "Left axis value"=0.0, "RobotDriveDevRef"=w435) -> ("error out"=w433:errorcluster, "Motor Values"=w438:dbl[], "RobotDriveDevRef"=w434:T6)  [unwired: 6 in]
                  n190 = call-poly <vilib>:"NT Write Value.vi"("Numeric Array"=w438, "Name"="RobotDrive Motors") -> ()  [unwired: 9 in, 1 out]
                  n191 = global read "Robot Global Data.vi" "Right Reset"() -> (w430:bool)
                  n192 = global read "Robot Global Data.vi" "Left Reset"() -> (w431:bool)
                  n193 = And(x=w431, y=w430) -> (x .and. y?=w429:bool)
                }
                frame False {
                  w474 = FALSE ("Left Reset")
                  n194 = Select(t=-1.0, s=w455, f=0.0) -> (s? t:f=w464:dbl)
                  n195 = Select(t=-1.0, s=w459, f=0.0) -> (s? t:f=w462:dbl)
                  n196 = Select(t=1.0, s=w460, f=w462) -> (s? t:f=w443:dbl)
                  n197 = Select(t=-1.0, s=w457, f=0.0) -> (s? t:f=w463:dbl)
                  n198 = Select(t=1.0, s=w458, f=w463) -> (s? t:f=w461:dbl)
                  n199 = Select(t=1.0, s=w456, f=w464) -> (s? t:f=w450:dbl)
                  n200 = call <vilib>:"WPI_SolenoidRefNum Registry Get.vi"("refnum name"="SOL A") -> ("error out"=w512:errorcluster, "SolenoidDevRef"=w513:T12)  [unwired: 9 in]
                  n201 = call <vilib>:"WPI_SolenoidRefNum Registry Get.vi"("refnum name"="SOL B") -> ("error out"=w509:errorcluster, "SolenoidDevRef"=w510:T12)  [unwired: 9 in]
                  n202 = Greater?(x=w486, y=w489) -> (0:w476:bool)
                  n203 = Greater?(x=w487, y=w488) -> (0:w475:bool)
                  n204 = call-poly <vilib>:"WPI_SolenoidSet.vi"("error in (no error)"=w512, "Value"=w491, "SolenoidDevRef"=w513) -> ()  [unwired: 7 in, 2 out]
                  n205 = call-poly <vilib>:"WPI_SolenoidSet.vi"("error in (no error)"=w509, "Value"=w490, "SolenoidDevRef"=w510) -> ()  [unwired: 7 in, 2 out]
                  n206 = Greater?(x=w447, y=90.0) -> (0:w451:bool)
                  n207 = call-poly <vilib>:"PID.vi"("output range"=cluster{"output high":dbl, "output low":dbl} {"output high"=1.0, "output low"=-1.0}, "PID gains"=T5 {"proportional gain (Kc)"=1.0, "integral time (Ti, min)"=0.01, "derivative time (Td, min)"=0.0}, "process variable"=w495, "setpoint"=w493) -> ("output"=w477:dbl)  [unwired: 6 in, 1 out]
                  n208 = Select(t=0.0, s=w451, f=w450) -> (s? t:f=w448:dbl)
                  n209 = call <vilib>:"WPI_MotorControlRefNum Registry Get.vi"("refnum name"="Lift") -> ("error out"=w507:errorcluster, "MotorControlDevRef"=w508:T7)  [unwired: 9 in]
                  n210 = call <vilib>:"WPI_MotorControlRefNum Registry Get.vi"("refnum name"="Intake") -> ("error out"=w505:errorcluster, "MotorControlDevRef"=w506:T7)  [unwired: 9 in]
                  n211 = call <vilib>:"WPI_MotorControlRefNum Registry Get.vi"("refnum name"="Wrist") -> ("error out"=w503:errorcluster, "MotorControlDevRef"=w504:T7)  [unwired: 9 in]
                  n212 = Less?(x=w441, y=0.0) -> (x < y?=w445:bool)
                  n213 = call-poly <vilib>:"PID.vi"("output range"=cluster{"output high":dbl, "output low":dbl} {"output high"=1.0, "output low"=-1.0}, "PID gains"=T5 {"proportional gain (Kc)"=1.0, "integral time (Ti, min)"=0.01, "derivative time (Td, min)"=0.0}, "process variable"=w494, "setpoint"=w492) -> ("output"=w478:dbl)  [unwired: 6 in, 1 out]
                  n214 = call <vilib>:"WPI_MotorControlSetOutput.vi"("error in (no error)"=w505, "Output"=w461, "MotorControlDevRef"=w506) -> ()  [unwired: 6 in, 3 out]
                  n215 = call <vilib>:"WPI_MotorControlSetOutput.vi"("error in (no error)"=w503, "Output"=w448, "MotorControlDevRef"=w504) -> ()  [unwired: 6 in, 3 out]
                  n216 = Select(t=0.0, s=w445, f=w443) -> (s? t:f=w442:dbl)
                  n217 = call <vilib>:"WPI_MotorControlSetOutput.vi"("error in (no error)"=w507, "Output"=w442, "MotorControlDevRef"=w508) -> ()  [unwired: 6 in, 3 out]
                  n218 = And(x=w476, y=w475) -> (x .and. y?=w482:bool)
                  n219 = Select(t=0.0, s=w476, f=w477) -> (s? t:f=w454:dbl)
                  n220 = Select(t=0.0, s=w475, f=w478) -> (s? t:f=w453:dbl)
                  n221 = call <vilib>:"WPI_RobotDriveTankDrive.vi"("Right axis value"=w453, "Left axis value"=w454, "RobotDriveDevRef"=w517) -> ("error out"=w481:errorcluster, "Motor Values"=w515:dbl[], "RobotDriveDevRef"=w518:T6)  [unwired: 6 in]
                  n222 = global write "Robot Global Data.vi" "Left Reset"(w474) -> ()
                  n223 = global write "Robot Global Data.vi" "Right Reset"(w474) -> ()
                  n224 = call-poly <vilib>:"NT Write Value.vi"("Numeric Array"=w515, "Name"="RobotDrive Motors") -> ()  [unwired: 9 in, 1 out]
                  n225 = Select(t=0.0, s=w482, f=w484) -> (s? t:f=w483:dbl)
                }
              }
            }
            n226 = call <vilib>:"WPI_RobotDriveDelayAndUpdateSafety.vi"("error in (no error)"=w397, "Delay (s)"=w398, "RobotDriveDevRef"=w402) -> ("RobotDriveDevRef 2"=w400:T6)  [unwired: 7 in, 1 out]
          }
        }
        frame "LLL", Default {
          n227 = call <vilib>:"WPI_RobotDriveRefNum Registry Get.vi"("refnum name"="Left and Right Motors") -> ("RobotDriveDevRef"=w521:T6)  [unwired: 1 in, 9 out]
          n228 = Array Size(array="Left LLL") -> (size(s)=w519:i32)
          n229 = for {
            N: w519 -> [_]
            shift-right: [w526] -> _
            shift-left: w521 -> [w527]
            tunnel: "Left LLL" -> [w525] mode=indexing
            n230 = while {
              shift-right: [w554] -> w528
              shift-left: w527 -> [w553]
              tunnel: w525 -> [w550]
              tunnel: [w534] -> w524
              tunnel: [w532] -> w523
              stop <- w533 stop-if-true
              n231 = global read "Robot Global Data.vi" "Left Rate Percent"() -> (w552:dbl)
              n232 = global read "Robot Global Data.vi" "Right Rate Percent"() -> (w551:dbl)
              n233 = Unbundle By Name(w550) -> ("Left Joystick"=w549:dbl, "Right Joystick"=w548:dbl, "Duration"=w535:dbl, "SOL A"=w547:bool, "SOL B"=w546:bool, "Lift Up"=w545:bool, "Lift Down"=w544:bool, "Intake In"=w543:bool, "Intake Out"=w542:bool, "Wrist Up"=w541:bool, "Wrist Down"=w540:bool, "Left Distance"=w539:dbl, "Right Distance"=w538:dbl, "Encoder Reset"=w531:bool)
              n234 = global read "Robot Global Data.vi" "Left Distance"() -> (w536:dbl)
              n235 = global read "Robot Global Data.vi" "Right Distance"() -> (w537:dbl)
              n236 = global read "Robot Global Data.vi" "Wrist Angle"() -> (w530:dbl)
              n237 = global read "Robot Global Data.vi" "Lift Distance"() -> (w529:dbl)
              n238 = case shown="False" w531 {
                tunnel: [w560 w644] -> w554
                tunnel: w553 -> [w561 w643]
                tunnel: w552 -> [_ w621]
                tunnel: w551 -> [_ w620]
                tunnel: w549 -> [_ w619]
                tunnel: w548 -> [_ w618]
                tunnel: w547 -> [_ w617]
                tunnel: w546 -> [_ w616]
                tunnel: w545 -> [_ w586]
                tunnel: w544 -> [_ w585]
                tunnel: w543 -> [_ w584]
                tunnel: w542 -> [_ w583]
                tunnel: w541 -> [_ w581]
                tunnel: w540 -> [_ w582]
                tunnel: w539 -> [_ w615]
                tunnel: w538 -> [_ w614]
                tunnel: w537 -> [_ w613]
                tunnel: w536 -> [_ w612]
                tunnel: w535 -> [w566 w610]
                tunnel: [w566 w609] -> w534
                tunnel: [w555 w608] -> w533
                tunnel: [w559 w607] -> w532
                tunnel: w530 -> [_ w573]
                tunnel: w529 -> [_ w567]
                frame True {
                  w558 = TRUE ("Left Reset")
                  n239 = global write "Robot Global Data.vi" "Left Reset"(w558) -> ()
                  n240 = global write "Robot Global Data.vi" "Right Reset"(w558) -> ()
                  n241 = call <vilib>:"WPI_RobotDriveTankDrive.vi"("Right axis value"=0.0, "Left axis value"=0.0, "RobotDriveDevRef"=w561) -> ("error out"=w559:errorcluster, "Motor Values"=w564:dbl[], "RobotDriveDevRef"=w560:T6)  [unwired: 6 in]
                  n242 = call-poly <vilib>:"NT Write Value.vi"("Numeric Array"=w564, "Name"="RobotDrive Motors") -> ()  [unwired: 9 in, 1 out]
                  n243 = global read "Robot Global Data.vi" "Right Reset"() -> (w556:bool)
                  n244 = global read "Robot Global Data.vi" "Left Reset"() -> (w557:bool)
                  n245 = And(x=w557, y=w556) -> (x .and. y?=w555:bool)
                }
                frame False {
                  w600 = FALSE ("Left Reset")
                  n246 = Select(t=-1.0, s=w581, f=0.0) -> (s? t:f=w590:dbl)
                  n247 = Select(t=-1.0, s=w585, f=0.0) -> (s? t:f=w588:dbl)
                  n248 = Select(t=1.0, s=w586, f=w588) -> (s? t:f=w569:dbl)
                  n249 = Select(t=-1.0, s=w583, f=0.0) -> (s? t:f=w589:dbl)
                  n250 = Select(t=1.0, s=w584, f=w589) -> (s? t:f=w587:dbl)
                  n251 = Select(t=1.0, s=w582, f=w590) -> (s? t:f=w576:dbl)
                  n252 = call <vilib>:"WPI_SolenoidRefNum Registry Get.vi"("refnum name"="SOL A") -> ("error out"=w638:errorcluster, "SolenoidDevRef"=w639:T12)  [unwired: 9 in]
                  n253 = call <vilib>:"WPI_SolenoidRefNum Registry Get.vi"("refnum name"="SOL B") -> ("error out"=w635:errorcluster, "SolenoidDevRef"=w636:T12)  [unwired: 9 in]
                  n254 = Greater?(x=w612, y=w615) -> (0:w602:bool)
                  n255 = Greater?(x=w613, y=w614) -> (0:w601:bool)
                  n256 = call-poly <vilib>:"WPI_SolenoidSet.vi"("error in (no error)"=w638, "Value"=w617, "SolenoidDevRef"=w639) -> ()  [unwired: 7 in, 2 out]
                  n257 = call-poly <vilib>:"WPI_SolenoidSet.vi"("error in (no error)"=w635, "Value"=w616, "SolenoidDevRef"=w636) -> ()  [unwired: 7 in, 2 out]
                  n258 = call-poly <vilib>:"PID.vi"("output range"=cluster{"output high":dbl, "output low":dbl} {"output high"=1.0, "output low"=-1.0}, "PID gains"=T5 {"proportional gain (Kc)"=1.0, "integral time (Ti, min)"=0.01, "derivative time (Td, min)"=0.0}, "process variable"=w621, "setpoint"=w619) -> ("output"=w603:dbl)  [unwired: 6 in, 1 out]
                  n259 = Greater?(x=w573, y=90.0) -> (0:w577:bool)
                  n260 = Select(t=0.0, s=w577, f=w576) -> (s? t:f=w574:dbl)
                  n261 = call <vilib>:"WPI_MotorControlRefNum Registry Get.vi"("refnum name"="Lift") -> ("error out"=w633:errorcluster, "MotorControlDevRef"=w634:T7)  [unwired: 9 in]
                  n262 = call <vilib>:"WPI_MotorControlRefNum Registry Get.vi"("refnum name"="Intake") -> ("error out"=w631:errorcluster, "MotorControlDevRef"=w632:T7)  [unwired: 9 in]
                  n263 = call <vilib>:"WPI_MotorControlRefNum Registry Get.vi"("refnum name"="Wrist") -> ("error out"=w629:errorcluster, "MotorControlDevRef"=w630:T7)  [unwired: 9 in]
                  n264 = Less?(x=w567, y=0.0) -> (x < y?=w571:bool)
                  n265 = call-poly <vilib>:"PID.vi"("output range"=cluster{"output high":dbl, "output low":dbl} {"output high"=1.0, "output low"=-1.0}, "PID gains"=T5 {"proportional gain (Kc)"=1.0, "integral time (Ti, min)"=0.01, "derivative time (Td, min)"=0.0}, "process variable"=w620, "setpoint"=w618) -> ("output"=w604:dbl)  [unwired: 6 in, 1 out]
                  n266 = call <vilib>:"WPI_MotorControlSetOutput.vi"("error in (no error)"=w631, "Output"=w587, "MotorControlDevRef"=w632) -> ()  [unwired: 6 in, 3 out]
                  n267 = call <vilib>:"WPI_MotorControlSetOutput.vi"("error in (no error)"=w629, "Output"=w574, "MotorControlDevRef"=w630) -> ()  [unwired: 6 in, 3 out]
                  n268 = Select(t=0.0, s=w571, f=w569) -> (s? t:f=w568:dbl)
                  n269 = call <vilib>:"WPI_MotorControlSetOutput.vi"("error in (no error)"=w633, "Output"=w568, "MotorControlDevRef"=w634) -> ()  [unwired: 6 in, 3 out]
                  n270 = And(x=w602, y=w601) -> (x .and. y?=w608:bool)
                  n271 = Select(t=0.0, s=w602, f=w603) -> (s? t:f=w580:dbl)
                  n272 = Select(t=0.0, s=w601, f=w604) -> (s? t:f=w579:dbl)
                  n273 = call <vilib>:"WPI_RobotDriveTankDrive.vi"("Right axis value"=w579, "Left axis value"=w580, "RobotDriveDevRef"=w643) -> ("error out"=w607:errorcluster, "Motor Values"=w641:dbl[], "RobotDriveDevRef"=w644:T6)  [unwired: 6 in]
                  n274 = global write "Robot Global Data.vi" "Left Reset"(w600) -> ()
                  n275 = global write "Robot Global Data.vi" "Right Reset"(w600) -> ()
                  n276 = call-poly <vilib>:"NT Write Value.vi"("Numeric Array"=w641, "Name"="RobotDrive Motors") -> ()  [unwired: 9 in, 1 out]
                  n277 = Select(t=0.0, s=w608, f=w610) -> (s? t:f=w609:dbl)
                }
              }
            }
            n278 = call <vilib>:"WPI_RobotDriveDelayAndUpdateSafety.vi"("error in (no error)"=w523, "Delay (s)"=w524, "RobotDriveDevRef"=w528) -> ("RobotDriveDevRef 2"=w526:T6)  [unwired: 7 in, 1 out]
          }
        }
      }
    }
    frame "Starting Center" {
      n279 = case shown="\"LRL\"" w645 {
        frame "RRR" {
          n280 = call <vilib>:"WPI_RobotDriveRefNum Registry Get.vi"("refnum name"="Left and Right Motors") -> ("RobotDriveDevRef"=w648:T6)  [unwired: 1 in, 9 out]
          n281 = Array Size(array="Center RRR") -> (size(s)=w646:i32)
          n282 = for {
            N: w646 -> [_]
            shift-right: [w653] -> _
            shift-left: w648 -> [w654]
            tunnel: "Center RRR" -> [w652] mode=indexing
            n283 = while {
              shift-right: [w681] -> w655
              shift-left: w654 -> [w680]
              tunnel: w652 -> [w677]
              tunnel: [w661] -> w651
              tunnel: [w659] -> w650
              stop <- w660 stop-if-true
              n284 = global read "Robot Global Data.vi" "Left Rate Percent"() -> (w679:dbl)
              n285 = global read "Robot Global Data.vi" "Right Rate Percent"() -> (w678:dbl)
              n286 = Unbundle By Name(w677) -> ("Left Joystick"=w676:dbl, "Right Joystick"=w675:dbl, "Duration"=w662:dbl, "SOL A"=w674:bool, "SOL B"=w673:bool, "Lift Up"=w672:bool, "Lift Down"=w671:bool, "Intake In"=w670:bool, "Intake Out"=w669:bool, "Wrist Up"=w668:bool, "Wrist Down"=w667:bool, "Left Distance"=w666:dbl, "Right Distance"=w665:dbl, "Encoder Reset"=w658:bool)
              n287 = global read "Robot Global Data.vi" "Left Distance"() -> (w663:dbl)
              n288 = global read "Robot Global Data.vi" "Right Distance"() -> (w664:dbl)
              n289 = global read "Robot Global Data.vi" "Wrist Angle"() -> (w657:dbl)
              n290 = global read "Robot Global Data.vi" "Lift Distance"() -> (w656:dbl)
              n291 = case shown="False" w658 {
                tunnel: [w687 w771] -> w681
                tunnel: w680 -> [w688 w770]
                tunnel: w679 -> [_ w748]
                tunnel: w678 -> [_ w747]
                tunnel: w676 -> [_ w746]
                tunnel: w675 -> [_ w745]
                tunnel: w674 -> [_ w744]
                tunnel: w673 -> [_ w743]
                tunnel: w672 -> [_ w713]
                tunnel: w671 -> [_ w712]
                tunnel: w670 -> [_ w711]
                tunnel: w669 -> [_ w710]
                tunnel: w668 -> [_ w708]
                tunnel: w667 -> [_ w709]
                tunnel: w666 -> [_ w742]
                tunnel: w665 -> [_ w741]
                tunnel: w664 -> [_ w740]
                tunnel: w663 -> [_ w739]
                tunnel: w662 -> [w693 w737]
                tunnel: [w693 w736] -> w661
                tunnel: [w682 w735] -> w660
                tunnel: [w686 w734] -> w659
                tunnel: w657 -> [_ w700]
                tunnel: w656 -> [_ w694]
                frame True {
                  w685 = TRUE ("Left Reset")
                  n292 = global write "Robot Global Data.vi" "Left Reset"(w685) -> ()
                  n293 = global write "Robot Global Data.vi" "Right Reset"(w685) -> ()
                  n294 = call <vilib>:"WPI_RobotDriveTankDrive.vi"("Right axis value"=0.0, "Left axis value"=0.0, "RobotDriveDevRef"=w688) -> ("error out"=w686:errorcluster, "Motor Values"=w691:dbl[], "RobotDriveDevRef"=w687:T6)  [unwired: 6 in]
                  n295 = call-poly <vilib>:"NT Write Value.vi"("Numeric Array"=w691, "Name"="RobotDrive Motors") -> ()  [unwired: 9 in, 1 out]
                  n296 = global read "Robot Global Data.vi" "Right Reset"() -> (w683:bool)
                  n297 = global read "Robot Global Data.vi" "Left Reset"() -> (w684:bool)
                  n298 = And(x=w684, y=w683) -> (x .and. y?=w682:bool)
                }
                frame False {
                  w727 = FALSE ("Left Reset")
                  n299 = Select(t=-1.0, s=w708, f=0.0) -> (s? t:f=w717:dbl)
                  n300 = Select(t=-1.0, s=w712, f=0.0) -> (s? t:f=w715:dbl)
                  n301 = Select(t=1.0, s=w713, f=w715) -> (s? t:f=w696:dbl)
                  n302 = Select(t=-1.0, s=w710, f=0.0) -> (s? t:f=w716:dbl)
                  n303 = Select(t=1.0, s=w711, f=w716) -> (s? t:f=w714:dbl)
                  n304 = Select(t=1.0, s=w709, f=w717) -> (s? t:f=w703:dbl)
                  n305 = call <vilib>:"WPI_SolenoidRefNum Registry Get.vi"("refnum name"="SOL A") -> ("error out"=w765:errorcluster, "SolenoidDevRef"=w766:T12)  [unwired: 9 in]
                  n306 = call <vilib>:"WPI_SolenoidRefNum Registry Get.vi"("refnum name"="SOL B") -> ("error out"=w762:errorcluster, "SolenoidDevRef"=w763:T12)  [unwired: 9 in]
                  n307 = Greater?(x=w739, y=w742) -> (0:w729:bool)
                  n308 = Greater?(x=w740, y=w741) -> (0:w728:bool)
                  n309 = call-poly <vilib>:"WPI_SolenoidSet.vi"("error in (no error)"=w765, "Value"=w744, "SolenoidDevRef"=w766) -> ()  [unwired: 7 in, 2 out]
                  n310 = call-poly <vilib>:"WPI_SolenoidSet.vi"("error in (no error)"=w762, "Value"=w743, "SolenoidDevRef"=w763) -> ()  [unwired: 7 in, 2 out]
                  n311 = Greater?(x=w700, y=90.0) -> (0:w704:bool)
                  n312 = call-poly <vilib>:"PID.vi"("output range"=cluster{"output high":dbl, "output low":dbl} {"output high"=1.0, "output low"=-1.0}, "PID gains"=T5 {"proportional gain (Kc)"=1.0, "integral time (Ti, min)"=0.01, "derivative time (Td, min)"=0.0}, "process variable"=w748, "setpoint"=w746) -> ("output"=w730:dbl)  [unwired: 6 in, 1 out]
                  n313 = Select(t=0.0, s=w704, f=w703) -> (s? t:f=w701:dbl)
                  n314 = call <vilib>:"WPI_MotorControlRefNum Registry Get.vi"("refnum name"="Lift") -> ("error out"=w760:errorcluster, "MotorControlDevRef"=w761:T7)  [unwired: 9 in]
                  n315 = call <vilib>:"WPI_MotorControlRefNum Registry Get.vi"("refnum name"="Intake") -> ("error out"=w758:errorcluster, "MotorControlDevRef"=w759:T7)  [unwired: 9 in]
                  n316 = call <vilib>:"WPI_MotorControlRefNum Registry Get.vi"("refnum name"="Wrist") -> ("error out"=w756:errorcluster, "MotorControlDevRef"=w757:T7)  [unwired: 9 in]
                  n317 = Less?(x=w694, y=0.0) -> (x < y?=w698:bool)
                  n318 = call-poly <vilib>:"PID.vi"("output range"=cluster{"output high":dbl, "output low":dbl} {"output high"=1.0, "output low"=-1.0}, "PID gains"=T5 {"proportional gain (Kc)"=1.0, "integral time (Ti, min)"=0.01, "derivative time (Td, min)"=0.0}, "process variable"=w747, "setpoint"=w745) -> ("output"=w731:dbl)  [unwired: 6 in, 1 out]
                  n319 = call <vilib>:"WPI_MotorControlSetOutput.vi"("error in (no error)"=w758, "Output"=w714, "MotorControlDevRef"=w759) -> ()  [unwired: 6 in, 3 out]
                  n320 = call <vilib>:"WPI_MotorControlSetOutput.vi"("error in (no error)"=w756, "Output"=w701, "MotorControlDevRef"=w757) -> ()  [unwired: 6 in, 3 out]
                  n321 = Select(t=0.0, s=w698, f=w696) -> (s? t:f=w695:dbl)
                  n322 = call <vilib>:"WPI_MotorControlSetOutput.vi"("error in (no error)"=w760, "Output"=w695, "MotorControlDevRef"=w761) -> ()  [unwired: 6 in, 3 out]
                  n323 = And(x=w729, y=w728) -> (x .and. y?=w735:bool)
                  n324 = Select(t=0.0, s=w729, f=w730) -> (s? t:f=w707:dbl)
                  n325 = Select(t=0.0, s=w728, f=w731) -> (s? t:f=w706:dbl)
                  n326 = call <vilib>:"WPI_RobotDriveTankDrive.vi"("Right axis value"=w706, "Left axis value"=w707, "RobotDriveDevRef"=w770) -> ("error out"=w734:errorcluster, "Motor Values"=w768:dbl[], "RobotDriveDevRef"=w771:T6)  [unwired: 6 in]
                  n327 = global write "Robot Global Data.vi" "Left Reset"(w727) -> ()
                  n328 = global write "Robot Global Data.vi" "Right Reset"(w727) -> ()
                  n329 = call-poly <vilib>:"NT Write Value.vi"("Numeric Array"=w768, "Name"="RobotDrive Motors") -> ()  [unwired: 9 in, 1 out]
                  n330 = Select(t=0.0, s=w735, f=w737) -> (s? t:f=w736:dbl)
                }
              }
            }
            n331 = call <vilib>:"WPI_RobotDriveDelayAndUpdateSafety.vi"("error in (no error)"=w650, "Delay (s)"=w651, "RobotDriveDevRef"=w655) -> ("RobotDriveDevRef 2"=w653:T6)  [unwired: 7 in, 1 out]
          }
        }
        frame "LRL" {
          n332 = call <vilib>:"WPI_RobotDriveRefNum Registry Get.vi"("refnum name"="Left and Right Motors") -> ("RobotDriveDevRef"=w774:T6)  [unwired: 1 in, 9 out]
          n333 = Array Size(array="Center LRL") -> (size(s)=w772:i32)
          n334 = for {
            N: w772 -> [_]
            shift-right: [w779] -> _
            shift-left: w774 -> [w780]
            tunnel: "Center LRL" -> [w778] mode=indexing
            n335 = while {
              shift-right: [w807] -> w781
              shift-left: w780 -> [w806]
              tunnel: w778 -> [w803]
              tunnel: [w787] -> w777
              tunnel: [w785] -> w776
              stop <- w786 stop-if-true
              n336 = global read "Robot Global Data.vi" "Left Rate Percent"() -> (w805:dbl)
              n337 = global read "Robot Global Data.vi" "Right Rate Percent"() -> (w804:dbl)
              n338 = Unbundle By Name(w803) -> ("Left Joystick"=w802:dbl, "Right Joystick"=w801:dbl, "Duration"=w788:dbl, "SOL A"=w800:bool, "SOL B"=w799:bool, "Lift Up"=w798:bool, "Lift Down"=w797:bool, "Intake In"=w796:bool, "Intake Out"=w795:bool, "Wrist Up"=w794:bool, "Wrist Down"=w793:bool, "Left Distance"=w792:dbl, "Right Distance"=w791:dbl, "Encoder Reset"=w784:bool)
              n339 = global read "Robot Global Data.vi" "Left Distance"() -> (w789:dbl)
              n340 = global read "Robot Global Data.vi" "Right Distance"() -> (w790:dbl)
              n341 = global read "Robot Global Data.vi" "Wrist Angle"() -> (w783:dbl)
              n342 = global read "Robot Global Data.vi" "Lift Distance"() -> (w782:dbl)
              n343 = case shown="False" w784 {
                tunnel: [w813 w897] -> w807
                tunnel: w806 -> [w814 w896]
                tunnel: w805 -> [_ w874]
                tunnel: w804 -> [_ w873]
                tunnel: w802 -> [_ w872]
                tunnel: w801 -> [_ w871]
                tunnel: w800 -> [_ w870]
                tunnel: w799 -> [_ w869]
                tunnel: w798 -> [_ w839]
                tunnel: w797 -> [_ w838]
                tunnel: w796 -> [_ w837]
                tunnel: w795 -> [_ w836]
                tunnel: w794 -> [_ w834]
                tunnel: w793 -> [_ w835]
                tunnel: w792 -> [_ w868]
                tunnel: w791 -> [_ w867]
                tunnel: w790 -> [_ w866]
                tunnel: w789 -> [_ w865]
                tunnel: w788 -> [w819 w863]
                tunnel: [w819 w862] -> w787
                tunnel: [w808 w861] -> w786
                tunnel: [w812 w860] -> w785
                tunnel: w783 -> [_ w826]
                tunnel: w782 -> [_ w820]
                frame True {
                  w811 = TRUE ("Left Reset")
                  n344 = global write "Robot Global Data.vi" "Left Reset"(w811) -> ()
                  n345 = global write "Robot Global Data.vi" "Right Reset"(w811) -> ()
                  n346 = call <vilib>:"WPI_RobotDriveTankDrive.vi"("Right axis value"=0.0, "Left axis value"=0.0, "RobotDriveDevRef"=w814) -> ("error out"=w812:errorcluster, "Motor Values"=w817:dbl[], "RobotDriveDevRef"=w813:T6)  [unwired: 6 in]
                  n347 = call-poly <vilib>:"NT Write Value.vi"("Numeric Array"=w817, "Name"="RobotDrive Motors") -> ()  [unwired: 9 in, 1 out]
                  n348 = global read "Robot Global Data.vi" "Right Reset"() -> (w809:bool)
                  n349 = global read "Robot Global Data.vi" "Left Reset"() -> (w810:bool)
                  n350 = And(x=w810, y=w809) -> (x .and. y?=w808:bool)
                }
                frame False {
                  w853 = FALSE ("Left Reset")
                  n351 = Select(t=-1.0, s=w834, f=0.0) -> (s? t:f=w843:dbl)
                  n352 = Select(t=-1.0, s=w838, f=0.0) -> (s? t:f=w841:dbl)
                  n353 = Select(t=1.0, s=w839, f=w841) -> (s? t:f=w822:dbl)
                  n354 = Select(t=-1.0, s=w836, f=0.0) -> (s? t:f=w842:dbl)
                  n355 = Select(t=1.0, s=w837, f=w842) -> (s? t:f=w840:dbl)
                  n356 = Select(t=1.0, s=w835, f=w843) -> (s? t:f=w829:dbl)
                  n357 = call <vilib>:"WPI_SolenoidRefNum Registry Get.vi"("refnum name"="SOL A") -> ("error out"=w891:errorcluster, "SolenoidDevRef"=w892:T12)  [unwired: 9 in]
                  n358 = call <vilib>:"WPI_SolenoidRefNum Registry Get.vi"("refnum name"="SOL B") -> ("error out"=w888:errorcluster, "SolenoidDevRef"=w889:T12)  [unwired: 9 in]
                  n359 = Greater?(x=w865, y=w868) -> (0:w855:bool)
                  n360 = Greater?(x=w866, y=w867) -> (0:w854:bool)
                  n361 = call-poly <vilib>:"WPI_SolenoidSet.vi"("error in (no error)"=w891, "Value"=w870, "SolenoidDevRef"=w892) -> ()  [unwired: 7 in, 2 out]
                  n362 = call-poly <vilib>:"WPI_SolenoidSet.vi"("error in (no error)"=w888, "Value"=w869, "SolenoidDevRef"=w889) -> ()  [unwired: 7 in, 2 out]
                  n363 = Greater?(x=w826, y=90.0) -> (0:w830:bool)
                  n364 = call-poly <vilib>:"PID.vi"("output range"=cluster{"output high":dbl, "output low":dbl} {"output high"=1.0, "output low"=-1.0}, "PID gains"=T5 {"proportional gain (Kc)"=1.0, "integral time (Ti, min)"=0.01, "derivative time (Td, min)"=0.0}, "process variable"=w874, "setpoint"=w872) -> ("output"=w856:dbl)  [unwired: 6 in, 1 out]
                  n365 = Select(t=0.0, s=w830, f=w829) -> (s? t:f=w827:dbl)
                  n366 = call <vilib>:"WPI_MotorControlRefNum Registry Get.vi"("refnum name"="Lift") -> ("error out"=w886:errorcluster, "MotorControlDevRef"=w887:T7)  [unwired: 9 in]
                  n367 = call <vilib>:"WPI_MotorControlRefNum Registry Get.vi"("refnum name"="Intake") -> ("error out"=w884:errorcluster, "MotorControlDevRef"=w885:T7)  [unwired: 9 in]
                  n368 = call <vilib>:"WPI_MotorControlRefNum Registry Get.vi"("refnum name"="Wrist") -> ("error out"=w882:errorcluster, "MotorControlDevRef"=w883:T7)  [unwired: 9 in]
                  n369 = Less?(x=w820, y=0.0) -> (x < y?=w824:bool)
                  n370 = call-poly <vilib>:"PID.vi"("output range"=cluster{"output high":dbl, "output low":dbl} {"output high"=1.0, "output low"=-1.0}, "PID gains"=T5 {"proportional gain (Kc)"=1.0, "integral time (Ti, min)"=0.01, "derivative time (Td, min)"=0.0}, "process variable"=w873, "setpoint"=w871) -> ("output"=w857:dbl)  [unwired: 6 in, 1 out]
                  n371 = call <vilib>:"WPI_MotorControlSetOutput.vi"("error in (no error)"=w884, "Output"=w840, "MotorControlDevRef"=w885) -> ()  [unwired: 6 in, 3 out]
                  n372 = call <vilib>:"WPI_MotorControlSetOutput.vi"("error in (no error)"=w882, "Output"=w827, "MotorControlDevRef"=w883) -> ()  [unwired: 6 in, 3 out]
                  n373 = Select(t=0.0, s=w824, f=w822) -> (s? t:f=w821:dbl)
                  n374 = call <vilib>:"WPI_MotorControlSetOutput.vi"("error in (no error)"=w886, "Output"=w821, "MotorControlDevRef"=w887) -> ()  [unwired: 6 in, 3 out]
                  n375 = And(x=w855, y=w854) -> (x .and. y?=w861:bool)
                  n376 = Select(t=0.0, s=w855, f=w856) -> (s? t:f=w833:dbl)
                  n377 = Select(t=0.0, s=w854, f=w857) -> (s? t:f=w832:dbl)
                  n378 = call <vilib>:"WPI_RobotDriveTankDrive.vi"("Right axis value"=w832, "Left axis value"=w833, "RobotDriveDevRef"=w896) -> ("error out"=w860:errorcluster, "Motor Values"=w894:dbl[], "RobotDriveDevRef"=w897:T6)  [unwired: 6 in]
                  n379 = global write "Robot Global Data.vi" "Left Reset"(w853) -> ()
                  n380 = global write "Robot Global Data.vi" "Right Reset"(w853) -> ()
                  n381 = call-poly <vilib>:"NT Write Value.vi"("Numeric Array"=w894, "Name"="RobotDrive Motors") -> ()  [unwired: 9 in, 1 out]
                  n382 = Select(t=0.0, s=w861, f=w863) -> (s? t:f=w862:dbl)
                }
              }
            }
            n383 = call <vilib>:"WPI_RobotDriveDelayAndUpdateSafety.vi"("error in (no error)"=w776, "Delay (s)"=w777, "RobotDriveDevRef"=w781) -> ("RobotDriveDevRef 2"=w779:T6)  [unwired: 7 in, 1 out]
          }
        }
        frame "RLR" {
          n384 = call <vilib>:"WPI_RobotDriveRefNum Registry Get.vi"("refnum name"="Left and Right Motors") -> ("RobotDriveDevRef"=w900:T6)  [unwired: 1 in, 9 out]
          n385 = Array Size(array="Center RLR") -> (size(s)=w898:i32)
          n386 = for {
            N: w898 -> [_]
            shift-right: [w905] -> _
            shift-left: w900 -> [w906]
            tunnel: "Center RLR" -> [w904] mode=indexing
            n387 = while {
              shift-right: [w933] -> w907
              shift-left: w906 -> [w932]
              tunnel: w904 -> [w929]
              tunnel: [w913] -> w903
              tunnel: [w911] -> w902
              stop <- w912 stop-if-true
              n388 = global read "Robot Global Data.vi" "Left Rate Percent"() -> (w931:dbl)
              n389 = global read "Robot Global Data.vi" "Right Rate Percent"() -> (w930:dbl)
              n390 = Unbundle By Name(w929) -> ("Left Joystick"=w928:dbl, "Right Joystick"=w927:dbl, "Duration"=w914:dbl, "SOL A"=w926:bool, "SOL B"=w925:bool, "Lift Up"=w924:bool, "Lift Down"=w923:bool, "Intake In"=w922:bool, "Intake Out"=w921:bool, "Wrist Up"=w920:bool, "Wrist Down"=w919:bool, "Left Distance"=w918:dbl, "Right Distance"=w917:dbl, "Encoder Reset"=w910:bool)
              n391 = global read "Robot Global Data.vi" "Left Distance"() -> (w915:dbl)
              n392 = global read "Robot Global Data.vi" "Right Distance"() -> (w916:dbl)
              n393 = global read "Robot Global Data.vi" "Wrist Angle"() -> (w909:dbl)
              n394 = global read "Robot Global Data.vi" "Lift Distance"() -> (w908:dbl)
              n395 = case shown="False" w910 {
                tunnel: [w939 w1023] -> w933
                tunnel: w932 -> [w940 w1022]
                tunnel: w931 -> [_ w1000]
                tunnel: w930 -> [_ w999]
                tunnel: w928 -> [_ w998]
                tunnel: w927 -> [_ w997]
                tunnel: w926 -> [_ w996]
                tunnel: w925 -> [_ w995]
                tunnel: w924 -> [_ w965]
                tunnel: w923 -> [_ w964]
                tunnel: w922 -> [_ w963]
                tunnel: w921 -> [_ w962]
                tunnel: w920 -> [_ w960]
                tunnel: w919 -> [_ w961]
                tunnel: w918 -> [_ w994]
                tunnel: w917 -> [_ w993]
                tunnel: w916 -> [_ w992]
                tunnel: w915 -> [_ w991]
                tunnel: w914 -> [w945 w989]
                tunnel: [w945 w988] -> w913
                tunnel: [w934 w987] -> w912
                tunnel: [w938 w986] -> w911
                tunnel: w909 -> [_ w952]
                tunnel: w908 -> [_ w946]
                frame True {
                  w937 = TRUE ("Left Reset")
                  n396 = global write "Robot Global Data.vi" "Left Reset"(w937) -> ()
                  n397 = global write "Robot Global Data.vi" "Right Reset"(w937) -> ()
                  n398 = call <vilib>:"WPI_RobotDriveTankDrive.vi"("Right axis value"=0.0, "Left axis value"=0.0, "RobotDriveDevRef"=w940) -> ("error out"=w938:errorcluster, "Motor Values"=w943:dbl[], "RobotDriveDevRef"=w939:T6)  [unwired: 6 in]
                  n399 = call-poly <vilib>:"NT Write Value.vi"("Numeric Array"=w943, "Name"="RobotDrive Motors") -> ()  [unwired: 9 in, 1 out]
                  n400 = global read "Robot Global Data.vi" "Right Reset"() -> (w935:bool)
                  n401 = global read "Robot Global Data.vi" "Left Reset"() -> (w936:bool)
                  n402 = And(x=w936, y=w935) -> (x .and. y?=w934:bool)
                }
                frame False {
                  w979 = FALSE ("Left Reset")
                  n403 = Select(t=-1.0, s=w960, f=0.0) -> (s? t:f=w969:dbl)
                  n404 = Select(t=-1.0, s=w964, f=0.0) -> (s? t:f=w967:dbl)
                  n405 = Select(t=1.0, s=w965, f=w967) -> (s? t:f=w948:dbl)
                  n406 = Select(t=-1.0, s=w962, f=0.0) -> (s? t:f=w968:dbl)
                  n407 = Select(t=1.0, s=w963, f=w968) -> (s? t:f=w966:dbl)
                  n408 = Select(t=1.0, s=w961, f=w969) -> (s? t:f=w955:dbl)
                  n409 = call <vilib>:"WPI_SolenoidRefNum Registry Get.vi"("refnum name"="SOL A") -> ("error out"=w1017:errorcluster, "SolenoidDevRef"=w1018:T12)  [unwired: 9 in]
                  n410 = call <vilib>:"WPI_SolenoidRefNum Registry Get.vi"("refnum name"="SOL B") -> ("error out"=w1014:errorcluster, "SolenoidDevRef"=w1015:T12)  [unwired: 9 in]
                  n411 = Greater?(x=w991, y=w994) -> (0:w981:bool)
                  n412 = Greater?(x=w992, y=w993) -> (0:w980:bool)
                  n413 = call-poly <vilib>:"WPI_SolenoidSet.vi"("error in (no error)"=w1017, "Value"=w996, "SolenoidDevRef"=w1018) -> ()  [unwired: 7 in, 2 out]
                  n414 = call-poly <vilib>:"WPI_SolenoidSet.vi"("error in (no error)"=w1014, "Value"=w995, "SolenoidDevRef"=w1015) -> ()  [unwired: 7 in, 2 out]
                  n415 = Greater?(x=w952, y=90.0) -> (0:w956:bool)
                  n416 = call-poly <vilib>:"PID.vi"("output range"=cluster{"output high":dbl, "output low":dbl} {"output high"=1.0, "output low"=-1.0}, "PID gains"=T5 {"proportional gain (Kc)"=1.0, "integral time (Ti, min)"=0.01, "derivative time (Td, min)"=0.0}, "process variable"=w1000, "setpoint"=w998) -> ("output"=w982:dbl)  [unwired: 6 in, 1 out]
                  n417 = Select(t=0.0, s=w956, f=w955) -> (s? t:f=w953:dbl)
                  n418 = call <vilib>:"WPI_MotorControlRefNum Registry Get.vi"("refnum name"="Lift") -> ("error out"=w1012:errorcluster, "MotorControlDevRef"=w1013:T7)  [unwired: 9 in]
                  n419 = call <vilib>:"WPI_MotorControlRefNum Registry Get.vi"("refnum name"="Intake") -> ("error out"=w1010:errorcluster, "MotorControlDevRef"=w1011:T7)  [unwired: 9 in]
                  n420 = call <vilib>:"WPI_MotorControlRefNum Registry Get.vi"("refnum name"="Wrist") -> ("error out"=w1008:errorcluster, "MotorControlDevRef"=w1009:T7)  [unwired: 9 in]
                  n421 = Less?(x=w946, y=0.0) -> (x < y?=w950:bool)
                  n422 = call-poly <vilib>:"PID.vi"("output range"=cluster{"output high":dbl, "output low":dbl} {"output high"=1.0, "output low"=-1.0}, "PID gains"=T5 {"proportional gain (Kc)"=1.0, "integral time (Ti, min)"=0.01, "derivative time (Td, min)"=0.0}, "process variable"=w999, "setpoint"=w997) -> ("output"=w983:dbl)  [unwired: 6 in, 1 out]
                  n423 = call <vilib>:"WPI_MotorControlSetOutput.vi"("error in (no error)"=w1010, "Output"=w966, "MotorControlDevRef"=w1011) -> ()  [unwired: 6 in, 3 out]
                  n424 = call <vilib>:"WPI_MotorControlSetOutput.vi"("error in (no error)"=w1008, "Output"=w953, "MotorControlDevRef"=w1009) -> ()  [unwired: 6 in, 3 out]
                  n425 = Select(t=0.0, s=w950, f=w948) -> (s? t:f=w947:dbl)
                  n426 = call <vilib>:"WPI_MotorControlSetOutput.vi"("error in (no error)"=w1012, "Output"=w947, "MotorControlDevRef"=w1013) -> ()  [unwired: 6 in, 3 out]
                  n427 = And(x=w981, y=w980) -> (x .and. y?=w987:bool)
                  n428 = Select(t=0.0, s=w981, f=w982) -> (s? t:f=w959:dbl)
                  n429 = Select(t=0.0, s=w980, f=w983) -> (s? t:f=w958:dbl)
                  n430 = call <vilib>:"WPI_RobotDriveTankDrive.vi"("Right axis value"=w958, "Left axis value"=w959, "RobotDriveDevRef"=w1022) -> ("error out"=w986:errorcluster, "Motor Values"=w1020:dbl[], "RobotDriveDevRef"=w1023:T6)  [unwired: 6 in]
                  n431 = global write "Robot Global Data.vi" "Left Reset"(w979) -> ()
                  n432 = global write "Robot Global Data.vi" "Right Reset"(w979) -> ()
                  n433 = call-poly <vilib>:"NT Write Value.vi"("Numeric Array"=w1020, "Name"="RobotDrive Motors") -> ()  [unwired: 9 in, 1 out]
                  n434 = Select(t=0.0, s=w987, f=w989) -> (s? t:f=w988:dbl)
                }
              }
            }
            n435 = call <vilib>:"WPI_RobotDriveDelayAndUpdateSafety.vi"("error in (no error)"=w902, "Delay (s)"=w903, "RobotDriveDevRef"=w907) -> ("RobotDriveDevRef 2"=w905:T6)  [unwired: 7 in, 1 out]
          }
        }
        frame "LLL", Default {
          n436 = call <vilib>:"WPI_RobotDriveRefNum Registry Get.vi"("refnum name"="Left and Right Motors") -> ("RobotDriveDevRef"=w1026:T6)  [unwired: 1 in, 9 out]
          n437 = Array Size(array="Center LLL") -> (size(s)=w1024:i32)
          n438 = for {
            N: w1024 -> [_]
            shift-right: [w1031] -> _
            shift-left: w1026 -> [w1032]
            tunnel: "Center LLL" -> [w1030] mode=indexing
            n439 = while {
              shift-right: [w1059] -> w1033
              shift-left: w1032 -> [w1058]
              tunnel: w1030 -> [w1055]
              tunnel: [w1039] -> w1029
              tunnel: [w1037] -> w1028
              stop <- w1038 stop-if-true
              n440 = global read "Robot Global Data.vi" "Left Rate Percent"() -> (w1057:dbl)
              n441 = global read "Robot Global Data.vi" "Right Rate Percent"() -> (w1056:dbl)
              n442 = Unbundle By Name(w1055) -> ("Left Joystick"=w1054:dbl, "Right Joystick"=w1053:dbl, "Duration"=w1040:dbl, "SOL A"=w1052:bool, "SOL B"=w1051:bool, "Lift Up"=w1050:bool, "Lift Down"=w1049:bool, "Intake In"=w1048:bool, "Intake Out"=w1047:bool, "Wrist Up"=w1046:bool, "Wrist Down"=w1045:bool, "Left Distance"=w1044:dbl, "Right Distance"=w1043:dbl, "Encoder Reset"=w1036:bool)
              n443 = global read "Robot Global Data.vi" "Left Distance"() -> (w1041:dbl)
              n444 = global read "Robot Global Data.vi" "Right Distance"() -> (w1042:dbl)
              n445 = global read "Robot Global Data.vi" "Wrist Angle"() -> (w1035:dbl)
              n446 = global read "Robot Global Data.vi" "Lift Distance"() -> (w1034:dbl)
              n447 = case shown="False" w1036 {
                tunnel: [w1065 w1149] -> w1059
                tunnel: w1058 -> [w1066 w1148]
                tunnel: w1057 -> [_ w1126]
                tunnel: w1056 -> [_ w1125]
                tunnel: w1054 -> [_ w1124]
                tunnel: w1053 -> [_ w1123]
                tunnel: w1052 -> [_ w1122]
                tunnel: w1051 -> [_ w1121]
                tunnel: w1050 -> [_ w1091]
                tunnel: w1049 -> [_ w1090]
                tunnel: w1048 -> [_ w1089]
                tunnel: w1047 -> [_ w1088]
                tunnel: w1046 -> [_ w1086]
                tunnel: w1045 -> [_ w1087]
                tunnel: w1044 -> [_ w1120]
                tunnel: w1043 -> [_ w1119]
                tunnel: w1042 -> [_ w1118]
                tunnel: w1041 -> [_ w1117]
                tunnel: w1040 -> [w1071 w1115]
                tunnel: [w1071 w1114] -> w1039
                tunnel: [w1060 w1113] -> w1038
                tunnel: [w1064 w1112] -> w1037
                tunnel: w1035 -> [_ w1078]
                tunnel: w1034 -> [_ w1072]
                frame True {
                  w1063 = TRUE ("Left Reset")
                  n448 = global write "Robot Global Data.vi" "Left Reset"(w1063) -> ()
                  n449 = global write "Robot Global Data.vi" "Right Reset"(w1063) -> ()
                  n450 = call <vilib>:"WPI_RobotDriveTankDrive.vi"("Right axis value"=0.0, "Left axis value"=0.0, "RobotDriveDevRef"=w1066) -> ("error out"=w1064:errorcluster, "Motor Values"=w1069:dbl[], "RobotDriveDevRef"=w1065:T6)  [unwired: 6 in]
                  n451 = call-poly <vilib>:"NT Write Value.vi"("Numeric Array"=w1069, "Name"="RobotDrive Motors") -> ()  [unwired: 9 in, 1 out]
                  n452 = global read "Robot Global Data.vi" "Right Reset"() -> (w1061:bool)
                  n453 = global read "Robot Global Data.vi" "Left Reset"() -> (w1062:bool)
                  n454 = And(x=w1062, y=w1061) -> (x .and. y?=w1060:bool)
                }
                frame False {
                  w1105 = FALSE ("Left Reset")
                  n455 = Select(t=-1.0, s=w1086, f=0.0) -> (s? t:f=w1095:dbl)
                  n456 = Select(t=-1.0, s=w1090, f=0.0) -> (s? t:f=w1093:dbl)
                  n457 = Select(t=1.0, s=w1091, f=w1093) -> (s? t:f=w1074:dbl)
                  n458 = Select(t=-1.0, s=w1088, f=0.0) -> (s? t:f=w1094:dbl)
                  n459 = Select(t=1.0, s=w1089, f=w1094) -> (s? t:f=w1092:dbl)
                  n460 = Select(t=1.0, s=w1087, f=w1095) -> (s? t:f=w1081:dbl)
                  n461 = call <vilib>:"WPI_SolenoidRefNum Registry Get.vi"("refnum name"="SOL A") -> ("error out"=w1143:errorcluster, "SolenoidDevRef"=w1144:T12)  [unwired: 9 in]
                  n462 = call <vilib>:"WPI_SolenoidRefNum Registry Get.vi"("refnum name"="SOL B") -> ("error out"=w1140:errorcluster, "SolenoidDevRef"=w1141:T12)  [unwired: 9 in]
                  n463 = Greater?(x=w1117, y=w1120) -> (0:w1107:bool)
                  n464 = Greater?(x=w1118, y=w1119) -> (0:w1106:bool)
                  n465 = call-poly <vilib>:"WPI_SolenoidSet.vi"("error in (no error)"=w1143, "Value"=w1122, "SolenoidDevRef"=w1144) -> ()  [unwired: 7 in, 2 out]
                  n466 = call-poly <vilib>:"WPI_SolenoidSet.vi"("error in (no error)"=w1140, "Value"=w1121, "SolenoidDevRef"=w1141) -> ()  [unwired: 7 in, 2 out]
                  n467 = Greater?(x=w1078, y=90.0) -> (0:w1082:bool)
                  n468 = call-poly <vilib>:"PID.vi"("output range"=cluster{"output high":dbl, "output low":dbl} {"output high"=1.0, "output low"=-1.0}, "PID gains"=T5 {"proportional gain (Kc)"=1.0, "integral time (Ti, min)"=0.01, "derivative time (Td, min)"=0.0}, "process variable"=w1126, "setpoint"=w1124) -> ("output"=w1108:dbl)  [unwired: 6 in, 1 out]
                  n469 = Select(t=0.0, s=w1082, f=w1081) -> (s? t:f=w1079:dbl)
                  n470 = call <vilib>:"WPI_MotorControlRefNum Registry Get.vi"("refnum name"="Lift") -> ("error out"=w1138:errorcluster, "MotorControlDevRef"=w1139:T7)  [unwired: 9 in]
                  n471 = call <vilib>:"WPI_MotorControlRefNum Registry Get.vi"("refnum name"="Intake") -> ("error out"=w1136:errorcluster, "MotorControlDevRef"=w1137:T7)  [unwired: 9 in]
                  n472 = call <vilib>:"WPI_MotorControlRefNum Registry Get.vi"("refnum name"="Wrist") -> ("error out"=w1134:errorcluster, "MotorControlDevRef"=w1135:T7)  [unwired: 9 in]
                  n473 = Less?(x=w1072, y=0.0) -> (x < y?=w1076:bool)
                  n474 = call-poly <vilib>:"PID.vi"("output range"=cluster{"output high":dbl, "output low":dbl} {"output high"=1.0, "output low"=-1.0}, "PID gains"=T5 {"proportional gain (Kc)"=1.0, "integral time (Ti, min)"=0.01, "derivative time (Td, min)"=0.0}, "process variable"=w1125, "setpoint"=w1123) -> ("output"=w1109:dbl)  [unwired: 6 in, 1 out]
                  n475 = call <vilib>:"WPI_MotorControlSetOutput.vi"("error in (no error)"=w1136, "Output"=w1092, "MotorControlDevRef"=w1137) -> ()  [unwired: 6 in, 3 out]
                  n476 = call <vilib>:"WPI_MotorControlSetOutput.vi"("error in (no error)"=w1134, "Output"=w1079, "MotorControlDevRef"=w1135) -> ()  [unwired: 6 in, 3 out]
                  n477 = Select(t=0.0, s=w1076, f=w1074) -> (s? t:f=w1073:dbl)
                  n478 = call <vilib>:"WPI_MotorControlSetOutput.vi"("error in (no error)"=w1138, "Output"=w1073, "MotorControlDevRef"=w1139) -> ()  [unwired: 6 in, 3 out]
                  n479 = And(x=w1107, y=w1106) -> (x .and. y?=w1113:bool)
                  n480 = Select(t=0.0, s=w1107, f=w1108) -> (s? t:f=w1085:dbl)
                  n481 = Select(t=0.0, s=w1106, f=w1109) -> (s? t:f=w1084:dbl)
                  n482 = call <vilib>:"WPI_RobotDriveTankDrive.vi"("Right axis value"=w1084, "Left axis value"=w1085, "RobotDriveDevRef"=w1148) -> ("error out"=w1112:errorcluster, "Motor Values"=w1146:dbl[], "RobotDriveDevRef"=w1149:T6)  [unwired: 6 in]
                  n483 = global write "Robot Global Data.vi" "Left Reset"(w1105) -> ()
                  n484 = global write "Robot Global Data.vi" "Right Reset"(w1105) -> ()
                  n485 = call-poly <vilib>:"NT Write Value.vi"("Numeric Array"=w1146, "Name"="RobotDrive Motors") -> ()  [unwired: 9 in, 1 out]
                  n486 = Select(t=0.0, s=w1113, f=w1115) -> (s? t:f=w1114:dbl)
                }
              }
            }
            n487 = call <vilib>:"WPI_RobotDriveDelayAndUpdateSafety.vi"("error in (no error)"=w1028, "Delay (s)"=w1029, "RobotDriveDevRef"=w1033) -> ("RobotDriveDevRef 2"=w1031:T6)  [unwired: 7 in, 1 out]
          }
        }
      }
    }
    frame "Starting Right" {
      n488 = case shown="\"LRL\"" w1150 {
        frame "RRR" {
          n489 = call <vilib>:"WPI_RobotDriveRefNum Registry Get.vi"("refnum name"="Left and Right Motors") -> ("RobotDriveDevRef"=w1153:T6)  [unwired: 1 in, 9 out]
          n490 = Array Size(array="Right RRR") -> (size(s)=w1151:i32)
          n491 = for {
            N: w1151 -> [_]
            shift-right: [w1158] -> _
            shift-left: w1153 -> [w1159]
            tunnel: "Right RRR" -> [w1157] mode=indexing
            n492 = while {
              shift-right: [w1186] -> w1160
              shift-left: w1159 -> [w1185]
              tunnel: w1157 -> [w1182]
              tunnel: [w1166] -> w1156
              tunnel: [w1164] -> w1155
              stop <- w1165 stop-if-true
              n493 = global read "Robot Global Data.vi" "Left Rate Percent"() -> (w1184:dbl)
              n494 = global read "Robot Global Data.vi" "Right Rate Percent"() -> (w1183:dbl)
              n495 = Unbundle By Name(w1182) -> ("Left Joystick"=w1181:dbl, "Right Joystick"=w1180:dbl, "Duration"=w1167:dbl, "SOL A"=w1179:bool, "SOL B"=w1178:bool, "Lift Up"=w1177:bool, "Lift Down"=w1176:bool, "Intake In"=w1175:bool, "Intake Out"=w1174:bool, "Wrist Up"=w1173:bool, "Wrist Down"=w1172:bool, "Left Distance"=w1171:dbl, "Right Distance"=w1170:dbl, "Encoder Reset"=w1163:bool)
              n496 = global read "Robot Global Data.vi" "Left Distance"() -> (w1168:dbl)
              n497 = global read "Robot Global Data.vi" "Right Distance"() -> (w1169:dbl)
              n498 = global read "Robot Global Data.vi" "Wrist Angle"() -> (w1162:dbl)
              n499 = global read "Robot Global Data.vi" "Lift Distance"() -> (w1161:dbl)
              n500 = case shown="False" w1163 {
                tunnel: [w1192 w1276] -> w1186
                tunnel: w1185 -> [w1193 w1275]
                tunnel: w1184 -> [_ w1253]
                tunnel: w1183 -> [_ w1252]
                tunnel: w1181 -> [_ w1251]
                tunnel: w1180 -> [_ w1250]
                tunnel: w1179 -> [_ w1249]
                tunnel: w1178 -> [_ w1248]
                tunnel: w1177 -> [_ w1218]
                tunnel: w1176 -> [_ w1217]
                tunnel: w1175 -> [_ w1216]
                tunnel: w1174 -> [_ w1215]
                tunnel: w1173 -> [_ w1213]
                tunnel: w1172 -> [_ w1214]
                tunnel: w1171 -> [_ w1247]
                tunnel: w1170 -> [_ w1246]
                tunnel: w1169 -> [_ w1245]
                tunnel: w1168 -> [_ w1244]
                tunnel: w1167 -> [w1198 w1242]
                tunnel: [w1198 w1241] -> w1166
                tunnel: [w1187 w1240] -> w1165
                tunnel: [w1191 w1239] -> w1164
                tunnel: w1162 -> [_ w1205]
                tunnel: w1161 -> [_ w1199]
                frame True {
                  w1190 = TRUE ("Left Reset")
                  n501 = global write "Robot Global Data.vi" "Left Reset"(w1190) -> ()
                  n502 = global write "Robot Global Data.vi" "Right Reset"(w1190) -> ()
                  n503 = call <vilib>:"WPI_RobotDriveTankDrive.vi"("Right axis value"=0.0, "Left axis value"=0.0, "RobotDriveDevRef"=w1193) -> ("error out"=w1191:errorcluster, "Motor Values"=w1196:dbl[], "RobotDriveDevRef"=w1192:T6)  [unwired: 6 in]
                  n504 = call-poly <vilib>:"NT Write Value.vi"("Numeric Array"=w1196, "Name"="RobotDrive Motors") -> ()  [unwired: 9 in, 1 out]
                  n505 = global read "Robot Global Data.vi" "Right Reset"() -> (w1188:bool)
                  n506 = global read "Robot Global Data.vi" "Left Reset"() -> (w1189:bool)
                  n507 = And(x=w1189, y=w1188) -> (x .and. y?=w1187:bool)
                }
                frame False {
                  w1232 = FALSE ("Left Reset")
                  n508 = Select(t=-1.0, s=w1213, f=0.0) -> (s? t:f=w1222:dbl)
                  n509 = Select(t=-1.0, s=w1217, f=0.0) -> (s? t:f=w1220:dbl)
                  n510 = Select(t=1.0, s=w1218, f=w1220) -> (s? t:f=w1201:dbl)
                  n511 = Select(t=-1.0, s=w1215, f=0.0) -> (s? t:f=w1221:dbl)
                  n512 = Select(t=1.0, s=w1216, f=w1221) -> (s? t:f=w1219:dbl)
                  n513 = Select(t=1.0, s=w1214, f=w1222) -> (s? t:f=w1208:dbl)
                  n514 = call <vilib>:"WPI_SolenoidRefNum Registry Get.vi"("refnum name"="SOL A") -> ("error out"=w1270:errorcluster, "SolenoidDevRef"=w1271:T12)  [unwired: 9 in]
                  n515 = call <vilib>:"WPI_SolenoidRefNum Registry Get.vi"("refnum name"="SOL B") -> ("error out"=w1267:errorcluster, "SolenoidDevRef"=w1268:T12)  [unwired: 9 in]
                  n516 = Greater?(x=w1244, y=w1247) -> (0:w1234:bool)
                  n517 = Greater?(x=w1245, y=w1246) -> (0:w1233:bool)
                  n518 = call-poly <vilib>:"WPI_SolenoidSet.vi"("error in (no error)"=w1270, "Value"=w1249, "SolenoidDevRef"=w1271) -> ()  [unwired: 7 in, 2 out]
                  n519 = call-poly <vilib>:"WPI_SolenoidSet.vi"("error in (no error)"=w1267, "Value"=w1248, "SolenoidDevRef"=w1268) -> ()  [unwired: 7 in, 2 out]
                  n520 = Greater?(x=w1205, y=90.0) -> (0:w1209:bool)
                  n521 = call-poly <vilib>:"PID.vi"("output range"=cluster{"output high":dbl, "output low":dbl} {"output high"=1.0, "output low"=-1.0}, "PID gains"=T5 {"proportional gain (Kc)"=1.0, "integral time (Ti, min)"=0.01, "derivative time (Td, min)"=0.0}, "process variable"=w1253, "setpoint"=w1251) -> ("output"=w1235:dbl)  [unwired: 6 in, 1 out]
                  n522 = Select(t=0.0, s=w1209, f=w1208) -> (s? t:f=w1206:dbl)
                  n523 = call <vilib>:"WPI_MotorControlRefNum Registry Get.vi"("refnum name"="Lift") -> ("error out"=w1265:errorcluster, "MotorControlDevRef"=w1266:T7)  [unwired: 9 in]
                  n524 = call <vilib>:"WPI_MotorControlRefNum Registry Get.vi"("refnum name"="Intake") -> ("error out"=w1263:errorcluster, "MotorControlDevRef"=w1264:T7)  [unwired: 9 in]
                  n525 = call <vilib>:"WPI_MotorControlRefNum Registry Get.vi"("refnum name"="Wrist") -> ("error out"=w1261:errorcluster, "MotorControlDevRef"=w1262:T7)  [unwired: 9 in]
                  n526 = Less?(x=w1199, y=0.0) -> (x < y?=w1203:bool)
                  n527 = call-poly <vilib>:"PID.vi"("output range"=cluster{"output high":dbl, "output low":dbl} {"output high"=1.0, "output low"=-1.0}, "PID gains"=T5 {"proportional gain (Kc)"=1.0, "integral time (Ti, min)"=0.01, "derivative time (Td, min)"=0.0}, "process variable"=w1252, "setpoint"=w1250) -> ("output"=w1236:dbl)  [unwired: 6 in, 1 out]
                  n528 = call <vilib>:"WPI_MotorControlSetOutput.vi"("error in (no error)"=w1263, "Output"=w1219, "MotorControlDevRef"=w1264) -> ()  [unwired: 6 in, 3 out]
                  n529 = call <vilib>:"WPI_MotorControlSetOutput.vi"("error in (no error)"=w1261, "Output"=w1206, "MotorControlDevRef"=w1262) -> ()  [unwired: 6 in, 3 out]
                  n530 = Select(t=0.0, s=w1203, f=w1201) -> (s? t:f=w1200:dbl)
                  n531 = call <vilib>:"WPI_MotorControlSetOutput.vi"("error in (no error)"=w1265, "Output"=w1200, "MotorControlDevRef"=w1266) -> ()  [unwired: 6 in, 3 out]
                  n532 = And(x=w1234, y=w1233) -> (x .and. y?=w1240:bool)
                  n533 = Select(t=0.0, s=w1234, f=w1235) -> (s? t:f=w1212:dbl)
                  n534 = Select(t=0.0, s=w1233, f=w1236) -> (s? t:f=w1211:dbl)
                  n535 = call <vilib>:"WPI_RobotDriveTankDrive.vi"("Right axis value"=w1211, "Left axis value"=w1212, "RobotDriveDevRef"=w1275) -> ("error out"=w1239:errorcluster, "Motor Values"=w1273:dbl[], "RobotDriveDevRef"=w1276:T6)  [unwired: 6 in]
                  n536 = global write "Robot Global Data.vi" "Left Reset"(w1232) -> ()
                  n537 = global write "Robot Global Data.vi" "Right Reset"(w1232) -> ()
                  n538 = call-poly <vilib>:"NT Write Value.vi"("Numeric Array"=w1273, "Name"="RobotDrive Motors") -> ()  [unwired: 9 in, 1 out]
                  n539 = Select(t=0.0, s=w1240, f=w1242) -> (s? t:f=w1241:dbl)
                }
              }
            }
            n540 = call <vilib>:"WPI_RobotDriveDelayAndUpdateSafety.vi"("error in (no error)"=w1155, "Delay (s)"=w1156, "RobotDriveDevRef"=w1160) -> ("RobotDriveDevRef 2"=w1158:T6)  [unwired: 7 in, 1 out]
          }
        }
        frame "LRL" {
          n541 = call <vilib>:"WPI_RobotDriveRefNum Registry Get.vi"("refnum name"="Left and Right Motors") -> ("RobotDriveDevRef"=w1279:T6)  [unwired: 1 in, 9 out]
          n542 = Array Size(array="Right LRL") -> (size(s)=w1277:i32)
          n543 = for {
            N: w1277 -> [_]
            shift-right: [w1284] -> _
            shift-left: w1279 -> [w1285]
            tunnel: "Right LRL" -> [w1283] mode=indexing
            n544 = while {
              shift-right: [w1312] -> w1286
              shift-left: w1285 -> [w1311]
              tunnel: w1283 -> [w1308]
              tunnel: [w1292] -> w1282
              tunnel: [w1290] -> w1281
              stop <- w1291 stop-if-true
              n545 = global read "Robot Global Data.vi" "Left Rate Percent"() -> (w1310:dbl)
              n546 = global read "Robot Global Data.vi" "Right Rate Percent"() -> (w1309:dbl)
              n547 = Unbundle By Name(w1308) -> ("Left Joystick"=w1307:dbl, "Right Joystick"=w1306:dbl, "Duration"=w1293:dbl, "SOL A"=w1305:bool, "SOL B"=w1304:bool, "Lift Up"=w1303:bool, "Lift Down"=w1302:bool, "Intake In"=w1301:bool, "Intake Out"=w1300:bool, "Wrist Up"=w1299:bool, "Wrist Down"=w1298:bool, "Left Distance"=w1297:dbl, "Right Distance"=w1296:dbl, "Encoder Reset"=w1289:bool)
              n548 = global read "Robot Global Data.vi" "Left Distance"() -> (w1294:dbl)
              n549 = global read "Robot Global Data.vi" "Right Distance"() -> (w1295:dbl)
              n550 = global read "Robot Global Data.vi" "Wrist Angle"() -> (w1288:dbl)
              n551 = global read "Robot Global Data.vi" "Lift Distance"() -> (w1287:dbl)
              n552 = case shown="False" w1289 {
                tunnel: [w1318 w1402] -> w1312
                tunnel: w1311 -> [w1319 w1401]
                tunnel: w1310 -> [_ w1379]
                tunnel: w1309 -> [_ w1378]
                tunnel: w1307 -> [_ w1377]
                tunnel: w1306 -> [_ w1376]
                tunnel: w1305 -> [_ w1375]
                tunnel: w1304 -> [_ w1374]
                tunnel: w1303 -> [_ w1344]
                tunnel: w1302 -> [_ w1343]
                tunnel: w1301 -> [_ w1342]
                tunnel: w1300 -> [_ w1341]
                tunnel: w1299 -> [_ w1339]
                tunnel: w1298 -> [_ w1340]
                tunnel: w1297 -> [_ w1373]
                tunnel: w1296 -> [_ w1372]
                tunnel: w1295 -> [_ w1371]
                tunnel: w1294 -> [_ w1370]
                tunnel: w1293 -> [w1324 w1368]
                tunnel: [w1324 w1367] -> w1292
                tunnel: [w1313 w1366] -> w1291
                tunnel: [w1317 w1365] -> w1290
                tunnel: w1288 -> [_ w1331]
                tunnel: w1287 -> [_ w1325]
                frame True {
                  w1316 = TRUE ("Left Reset")
                  n553 = global write "Robot Global Data.vi" "Left Reset"(w1316) -> ()
                  n554 = global write "Robot Global Data.vi" "Right Reset"(w1316) -> ()
                  n555 = call <vilib>:"WPI_RobotDriveTankDrive.vi"("Right axis value"=0.0, "Left axis value"=0.0, "RobotDriveDevRef"=w1319) -> ("error out"=w1317:errorcluster, "Motor Values"=w1322:dbl[], "RobotDriveDevRef"=w1318:T6)  [unwired: 6 in]
                  n556 = call-poly <vilib>:"NT Write Value.vi"("Numeric Array"=w1322, "Name"="RobotDrive Motors") -> ()  [unwired: 9 in, 1 out]
                  n557 = global read "Robot Global Data.vi" "Right Reset"() -> (w1314:bool)
                  n558 = global read "Robot Global Data.vi" "Left Reset"() -> (w1315:bool)
                  n559 = And(x=w1315, y=w1314) -> (x .and. y?=w1313:bool)
                }
                frame False {
                  w1358 = FALSE ("Left Reset")
                  n560 = Select(t=-1.0, s=w1339, f=0.0) -> (s? t:f=w1348:dbl)
                  n561 = Select(t=-1.0, s=w1343, f=0.0) -> (s? t:f=w1346:dbl)
                  n562 = Select(t=1.0, s=w1344, f=w1346) -> (s? t:f=w1327:dbl)
                  n563 = Select(t=-1.0, s=w1341, f=0.0) -> (s? t:f=w1347:dbl)
                  n564 = Select(t=1.0, s=w1342, f=w1347) -> (s? t:f=w1345:dbl)
                  n565 = Select(t=1.0, s=w1340, f=w1348) -> (s? t:f=w1334:dbl)
                  n566 = call <vilib>:"WPI_SolenoidRefNum Registry Get.vi"("refnum name"="SOL A") -> ("error out"=w1396:errorcluster, "SolenoidDevRef"=w1397:T12)  [unwired: 9 in]
                  n567 = call <vilib>:"WPI_SolenoidRefNum Registry Get.vi"("refnum name"="SOL B") -> ("error out"=w1393:errorcluster, "SolenoidDevRef"=w1394:T12)  [unwired: 9 in]
                  n568 = Greater?(x=w1370, y=w1373) -> (0:w1360:bool)
                  n569 = Greater?(x=w1371, y=w1372) -> (0:w1359:bool)
                  n570 = call-poly <vilib>:"WPI_SolenoidSet.vi"("error in (no error)"=w1396, "Value"=w1375, "SolenoidDevRef"=w1397) -> ()  [unwired: 7 in, 2 out]
                  n571 = call-poly <vilib>:"WPI_SolenoidSet.vi"("error in (no error)"=w1393, "Value"=w1374, "SolenoidDevRef"=w1394) -> ()  [unwired: 7 in, 2 out]
                  n572 = Greater?(x=w1331, y=90.0) -> (0:w1335:bool)
                  n573 = call-poly <vilib>:"PID.vi"("output range"=cluster{"output high":dbl, "output low":dbl} {"output high"=1.0, "output low"=-1.0}, "PID gains"=T5 {"proportional gain (Kc)"=1.0, "integral time (Ti, min)"=0.01, "derivative time (Td, min)"=0.0}, "process variable"=w1379, "setpoint"=w1377) -> ("output"=w1361:dbl)  [unwired: 6 in, 1 out]
                  n574 = Select(t=0.0, s=w1335, f=w1334) -> (s? t:f=w1332:dbl)
                  n575 = call <vilib>:"WPI_MotorControlRefNum Registry Get.vi"("refnum name"="Lift") -> ("error out"=w1391:errorcluster, "MotorControlDevRef"=w1392:T7)  [unwired: 9 in]
                  n576 = call <vilib>:"WPI_MotorControlRefNum Registry Get.vi"("refnum name"="Intake") -> ("error out"=w1389:errorcluster, "MotorControlDevRef"=w1390:T7)  [unwired: 9 in]
                  n577 = call <vilib>:"WPI_MotorControlRefNum Registry Get.vi"("refnum name"="Wrist") -> ("error out"=w1387:errorcluster, "MotorControlDevRef"=w1388:T7)  [unwired: 9 in]
                  n578 = Less?(x=w1325, y=0.0) -> (x < y?=w1329:bool)
                  n579 = call-poly <vilib>:"PID.vi"("output range"=cluster{"output high":dbl, "output low":dbl} {"output high"=1.0, "output low"=-1.0}, "PID gains"=T5 {"proportional gain (Kc)"=1.0, "integral time (Ti, min)"=0.01, "derivative time (Td, min)"=0.0}, "process variable"=w1378, "setpoint"=w1376) -> ("output"=w1362:dbl)  [unwired: 6 in, 1 out]
                  n580 = call <vilib>:"WPI_MotorControlSetOutput.vi"("error in (no error)"=w1389, "Output"=w1345, "MotorControlDevRef"=w1390) -> ()  [unwired: 6 in, 3 out]
                  n581 = call <vilib>:"WPI_MotorControlSetOutput.vi"("error in (no error)"=w1387, "Output"=w1332, "MotorControlDevRef"=w1388) -> ()  [unwired: 6 in, 3 out]
                  n582 = Select(t=0.0, s=w1329, f=w1327) -> (s? t:f=w1326:dbl)
                  n583 = call <vilib>:"WPI_MotorControlSetOutput.vi"("error in (no error)"=w1391, "Output"=w1326, "MotorControlDevRef"=w1392) -> ()  [unwired: 6 in, 3 out]
                  n584 = And(x=w1360, y=w1359) -> (x .and. y?=w1366:bool)
                  n585 = Select(t=0.0, s=w1360, f=w1361) -> (s? t:f=w1338:dbl)
                  n586 = Select(t=0.0, s=w1359, f=w1362) -> (s? t:f=w1337:dbl)
                  n587 = call <vilib>:"WPI_RobotDriveTankDrive.vi"("Right axis value"=w1337, "Left axis value"=w1338, "RobotDriveDevRef"=w1401) -> ("error out"=w1365:errorcluster, "Motor Values"=w1399:dbl[], "RobotDriveDevRef"=w1402:T6)  [unwired: 6 in]
                  n588 = global write "Robot Global Data.vi" "Left Reset"(w1358) -> ()
                  n589 = global write "Robot Global Data.vi" "Right Reset"(w1358) -> ()
                  n590 = call-poly <vilib>:"NT Write Value.vi"("Numeric Array"=w1399, "Name"="RobotDrive Motors") -> ()  [unwired: 9 in, 1 out]
                  n591 = Select(t=0.0, s=w1366, f=w1368) -> (s? t:f=w1367:dbl)
                }
              }
            }
            n592 = call <vilib>:"WPI_RobotDriveDelayAndUpdateSafety.vi"("error in (no error)"=w1281, "Delay (s)"=w1282, "RobotDriveDevRef"=w1286) -> ("RobotDriveDevRef 2"=w1284:T6)  [unwired: 7 in, 1 out]
          }
        }
        frame "RLR" {
          n593 = call <vilib>:"WPI_RobotDriveRefNum Registry Get.vi"("refnum name"="Left and Right Motors") -> ("RobotDriveDevRef"=w1405:T6)  [unwired: 1 in, 9 out]
          n594 = Array Size(array="Right RLR") -> (size(s)=w1403:i32)
          n595 = for {
            N: w1403 -> [_]
            shift-right: [w1410] -> _
            shift-left: w1405 -> [w1411]
            tunnel: "Right RLR" -> [w1409] mode=indexing
            n596 = while {
              shift-right: [w1438] -> w1412
              shift-left: w1411 -> [w1437]
              tunnel: w1409 -> [w1434]
              tunnel: [w1418] -> w1408
              tunnel: [w1416] -> w1407
              stop <- w1417 stop-if-true
              n597 = global read "Robot Global Data.vi" "Left Rate Percent"() -> (w1436:dbl)
              n598 = global read "Robot Global Data.vi" "Right Rate Percent"() -> (w1435:dbl)
              n599 = Unbundle By Name(w1434) -> ("Left Joystick"=w1433:dbl, "Right Joystick"=w1432:dbl, "Duration"=w1419:dbl, "SOL A"=w1431:bool, "SOL B"=w1430:bool, "Lift Up"=w1429:bool, "Lift Down"=w1428:bool, "Intake In"=w1427:bool, "Intake Out"=w1426:bool, "Wrist Up"=w1425:bool, "Wrist Down"=w1424:bool, "Left Distance"=w1423:dbl, "Right Distance"=w1422:dbl, "Encoder Reset"=w1415:bool)
              n600 = global read "Robot Global Data.vi" "Left Distance"() -> (w1420:dbl)
              n601 = global read "Robot Global Data.vi" "Right Distance"() -> (w1421:dbl)
              n602 = global read "Robot Global Data.vi" "Wrist Angle"() -> (w1414:dbl)
              n603 = global read "Robot Global Data.vi" "Lift Distance"() -> (w1413:dbl)
              n604 = case shown="False" w1415 {
                tunnel: [w1444 w1528] -> w1438
                tunnel: w1437 -> [w1445 w1527]
                tunnel: w1436 -> [_ w1505]
                tunnel: w1435 -> [_ w1504]
                tunnel: w1433 -> [_ w1503]
                tunnel: w1432 -> [_ w1502]
                tunnel: w1431 -> [_ w1501]
                tunnel: w1430 -> [_ w1500]
                tunnel: w1429 -> [_ w1470]
                tunnel: w1428 -> [_ w1469]
                tunnel: w1427 -> [_ w1468]
                tunnel: w1426 -> [_ w1467]
                tunnel: w1425 -> [_ w1465]
                tunnel: w1424 -> [_ w1466]
                tunnel: w1423 -> [_ w1499]
                tunnel: w1422 -> [_ w1498]
                tunnel: w1421 -> [_ w1497]
                tunnel: w1420 -> [_ w1496]
                tunnel: w1419 -> [w1450 w1494]
                tunnel: [w1450 w1493] -> w1418
                tunnel: [w1439 w1492] -> w1417
                tunnel: [w1443 w1491] -> w1416
                tunnel: w1414 -> [_ w1457]
                tunnel: w1413 -> [_ w1451]
                frame True {
                  w1442 = TRUE ("Left Reset")
                  n605 = global write "Robot Global Data.vi" "Left Reset"(w1442) -> ()
                  n606 = global write "Robot Global Data.vi" "Right Reset"(w1442) -> ()
                  n607 = call <vilib>:"WPI_RobotDriveTankDrive.vi"("Right axis value"=0.0, "Left axis value"=0.0, "RobotDriveDevRef"=w1445) -> ("error out"=w1443:errorcluster, "Motor Values"=w1448:dbl[], "RobotDriveDevRef"=w1444:T6)  [unwired: 6 in]
                  n608 = call-poly <vilib>:"NT Write Value.vi"("Numeric Array"=w1448, "Name"="RobotDrive Motors") -> ()  [unwired: 9 in, 1 out]
                  n609 = global read "Robot Global Data.vi" "Right Reset"() -> (w1440:bool)
                  n610 = global read "Robot Global Data.vi" "Left Reset"() -> (w1441:bool)
                  n611 = And(x=w1441, y=w1440) -> (x .and. y?=w1439:bool)
                }
                frame False {
                  w1484 = FALSE ("Left Reset")
                  n612 = Select(t=-1.0, s=w1465, f=0.0) -> (s? t:f=w1474:dbl)
                  n613 = Select(t=-1.0, s=w1469, f=0.0) -> (s? t:f=w1472:dbl)
                  n614 = Select(t=1.0, s=w1470, f=w1472) -> (s? t:f=w1453:dbl)
                  n615 = Select(t=-1.0, s=w1467, f=0.0) -> (s? t:f=w1473:dbl)
                  n616 = Select(t=1.0, s=w1468, f=w1473) -> (s? t:f=w1471:dbl)
                  n617 = Select(t=1.0, s=w1466, f=w1474) -> (s? t:f=w1460:dbl)
                  n618 = call <vilib>:"WPI_SolenoidRefNum Registry Get.vi"("refnum name"="SOL A") -> ("error out"=w1522:errorcluster, "SolenoidDevRef"=w1523:T12)  [unwired: 9 in]
                  n619 = call <vilib>:"WPI_SolenoidRefNum Registry Get.vi"("refnum name"="SOL B") -> ("error out"=w1519:errorcluster, "SolenoidDevRef"=w1520:T12)  [unwired: 9 in]
                  n620 = Greater?(x=w1496, y=w1499) -> (0:w1486:bool)
                  n621 = Greater?(x=w1497, y=w1498) -> (0:w1485:bool)
                  n622 = call-poly <vilib>:"WPI_SolenoidSet.vi"("error in (no error)"=w1522, "Value"=w1501, "SolenoidDevRef"=w1523) -> ()  [unwired: 7 in, 2 out]
                  n623 = call-poly <vilib>:"WPI_SolenoidSet.vi"("error in (no error)"=w1519, "Value"=w1500, "SolenoidDevRef"=w1520) -> ()  [unwired: 7 in, 2 out]
                  n624 = Greater?(x=w1457, y=90.0) -> (0:w1461:bool)
                  n625 = call-poly <vilib>:"PID.vi"("output range"=cluster{"output high":dbl, "output low":dbl} {"output high"=1.0, "output low"=-1.0}, "PID gains"=T5 {"proportional gain (Kc)"=1.0, "integral time (Ti, min)"=0.01, "derivative time (Td, min)"=0.0}, "process variable"=w1505, "setpoint"=w1503) -> ("output"=w1487:dbl)  [unwired: 6 in, 1 out]
                  n626 = Select(t=0.0, s=w1461, f=w1460) -> (s? t:f=w1458:dbl)
                  n627 = call <vilib>:"WPI_MotorControlRefNum Registry Get.vi"("refnum name"="Lift") -> ("error out"=w1517:errorcluster, "MotorControlDevRef"=w1518:T7)  [unwired: 9 in]
                  n628 = call <vilib>:"WPI_MotorControlRefNum Registry Get.vi"("refnum name"="Intake") -> ("error out"=w1515:errorcluster, "MotorControlDevRef"=w1516:T7)  [unwired: 9 in]
                  n629 = call <vilib>:"WPI_MotorControlRefNum Registry Get.vi"("refnum name"="Wrist") -> ("error out"=w1513:errorcluster, "MotorControlDevRef"=w1514:T7)  [unwired: 9 in]
                  n630 = Less?(x=w1451, y=0.0) -> (x < y?=w1455:bool)
                  n631 = call-poly <vilib>:"PID.vi"("output range"=cluster{"output high":dbl, "output low":dbl} {"output high"=1.0, "output low"=-1.0}, "PID gains"=T5 {"proportional gain (Kc)"=1.0, "integral time (Ti, min)"=0.01, "derivative time (Td, min)"=0.0}, "process variable"=w1504, "setpoint"=w1502) -> ("output"=w1488:dbl)  [unwired: 6 in, 1 out]
                  n632 = call <vilib>:"WPI_MotorControlSetOutput.vi"("error in (no error)"=w1515, "Output"=w1471, "MotorControlDevRef"=w1516) -> ()  [unwired: 6 in, 3 out]
                  n633 = call <vilib>:"WPI_MotorControlSetOutput.vi"("error in (no error)"=w1513, "Output"=w1458, "MotorControlDevRef"=w1514) -> ()  [unwired: 6 in, 3 out]
                  n634 = Select(t=0.0, s=w1455, f=w1453) -> (s? t:f=w1452:dbl)
                  n635 = call <vilib>:"WPI_MotorControlSetOutput.vi"("error in (no error)"=w1517, "Output"=w1452, "MotorControlDevRef"=w1518) -> ()  [unwired: 6 in, 3 out]
                  n636 = And(x=w1486, y=w1485) -> (x .and. y?=w1492:bool)
                  n637 = Select(t=0.0, s=w1486, f=w1487) -> (s? t:f=w1464:dbl)
                  n638 = Select(t=0.0, s=w1485, f=w1488) -> (s? t:f=w1463:dbl)
                  n639 = call <vilib>:"WPI_RobotDriveTankDrive.vi"("Right axis value"=w1463, "Left axis value"=w1464, "RobotDriveDevRef"=w1527) -> ("error out"=w1491:errorcluster, "Motor Values"=w1525:dbl[], "RobotDriveDevRef"=w1528:T6)  [unwired: 6 in]
                  n640 = global write "Robot Global Data.vi" "Left Reset"(w1484) -> ()
                  n641 = global write "Robot Global Data.vi" "Right Reset"(w1484) -> ()
                  n642 = call-poly <vilib>:"NT Write Value.vi"("Numeric Array"=w1525, "Name"="RobotDrive Motors") -> ()  [unwired: 9 in, 1 out]
                  n643 = Select(t=0.0, s=w1492, f=w1494) -> (s? t:f=w1493:dbl)
                }
              }
            }
            n644 = call <vilib>:"WPI_RobotDriveDelayAndUpdateSafety.vi"("error in (no error)"=w1407, "Delay (s)"=w1408, "RobotDriveDevRef"=w1412) -> ("RobotDriveDevRef 2"=w1410:T6)  [unwired: 7 in, 1 out]
          }
        }
        frame "LLL", Default {
          n645 = call <vilib>:"WPI_RobotDriveRefNum Registry Get.vi"("refnum name"="Left and Right Motors") -> ("RobotDriveDevRef"=w1531:T6)  [unwired: 1 in, 9 out]
          n646 = Array Size(array="Right LLL") -> (size(s)=w1529:i32)
          n647 = for {
            N: w1529 -> [_]
            shift-right: [w1536] -> _
            shift-left: w1531 -> [w1537]
            tunnel: "Right LLL" -> [w1535] mode=indexing
            n648 = while {
              shift-right: [w1564] -> w1538
              shift-left: w1537 -> [w1563]
              tunnel: w1535 -> [w1560]
              tunnel: [w1544] -> w1534
              tunnel: [w1542] -> w1533
              stop <- w1543 stop-if-true
              n649 = global read "Robot Global Data.vi" "Left Rate Percent"() -> (w1562:dbl)
              n650 = global read "Robot Global Data.vi" "Right Rate Percent"() -> (w1561:dbl)
              n651 = Unbundle By Name(w1560) -> ("Left Joystick"=w1559:dbl, "Right Joystick"=w1558:dbl, "Duration"=w1545:dbl, "SOL A"=w1557:bool, "SOL B"=w1556:bool, "Lift Up"=w1555:bool, "Lift Down"=w1554:bool, "Intake In"=w1553:bool, "Intake Out"=w1552:bool, "Wrist Up"=w1551:bool, "Wrist Down"=w1550:bool, "Left Distance"=w1549:dbl, "Right Distance"=w1548:dbl, "Encoder Reset"=w1541:bool)
              n652 = global read "Robot Global Data.vi" "Left Distance"() -> (w1546:dbl)
              n653 = global read "Robot Global Data.vi" "Right Distance"() -> (w1547:dbl)
              n654 = global read "Robot Global Data.vi" "Wrist Angle"() -> (w1540:dbl)
              n655 = global read "Robot Global Data.vi" "Lift Distance"() -> (w1539:dbl)
              n656 = case shown="False" w1541 {
                tunnel: [w1570 w1654] -> w1564
                tunnel: w1563 -> [w1571 w1653]
                tunnel: w1562 -> [_ w1631]
                tunnel: w1561 -> [_ w1630]
                tunnel: w1559 -> [_ w1629]
                tunnel: w1558 -> [_ w1628]
                tunnel: w1557 -> [_ w1577]
                tunnel: w1556 -> [_ w1627]
                tunnel: w1555 -> [_ w1597]
                tunnel: w1554 -> [_ w1596]
                tunnel: w1553 -> [_ w1595]
                tunnel: w1552 -> [_ w1594]
                tunnel: w1551 -> [_ w1592]
                tunnel: w1550 -> [_ w1593]
                tunnel: w1549 -> [_ w1626]
                tunnel: w1548 -> [_ w1625]
                tunnel: w1547 -> [_ w1624]
                tunnel: w1546 -> [_ w1623]
                tunnel: w1545 -> [w1576 w1621]
                tunnel: [w1576 w1620] -> w1544
                tunnel: [w1565 w1619] -> w1543
                tunnel: [w1569 w1618] -> w1542
                tunnel: w1540 -> [_ w1584]
                tunnel: w1539 -> [_ w1578]
                frame True {
                  w1568 = TRUE ("Left Reset")
                  n657 = global write "Robot Global Data.vi" "Left Reset"(w1568) -> ()
                  n658 = global write "Robot Global Data.vi" "Right Reset"(w1568) -> ()
                  n659 = call <vilib>:"WPI_RobotDriveTankDrive.vi"("Right axis value"=0.0, "Left axis value"=0.0, "RobotDriveDevRef"=w1571) -> ("error out"=w1569:errorcluster, "Motor Values"=w1574:dbl[], "RobotDriveDevRef"=w1570:T6)  [unwired: 6 in]
                  n660 = call-poly <vilib>:"NT Write Value.vi"("Numeric Array"=w1574, "Name"="RobotDrive Motors") -> ()  [unwired: 9 in, 1 out]
                  n661 = global read "Robot Global Data.vi" "Right Reset"() -> (w1566:bool)
                  n662 = global read "Robot Global Data.vi" "Left Reset"() -> (w1567:bool)
                  n663 = And(x=w1567, y=w1566) -> (x .and. y?=w1565:bool)
                }
                frame False {
                  w1611 = FALSE ("Left Reset")
                  n664 = Select(t=-1.0, s=w1592, f=0.0) -> (s? t:f=w1601:dbl)
                  n665 = Select(t=-1.0, s=w1596, f=0.0) -> (s? t:f=w1599:dbl)
                  n666 = Select(t=1.0, s=w1597, f=w1599) -> (s? t:f=w1580:dbl)
                  n667 = Select(t=-1.0, s=w1594, f=0.0) -> (s? t:f=w1600:dbl)
                  n668 = Select(t=1.0, s=w1595, f=w1600) -> (s? t:f=w1598:dbl)
                  n669 = Select(t=1.0, s=w1593, f=w1601) -> (s? t:f=w1587:dbl)
                  n670 = call <vilib>:"WPI_SolenoidRefNum Registry Get.vi"("refnum name"="SOL A") -> ("error out"=w1648:errorcluster, "SolenoidDevRef"=w1649:T12)  [unwired: 9 in]
                  n671 = call <vilib>:"WPI_SolenoidRefNum Registry Get.vi"("refnum name"="SOL B") -> ("error out"=w1645:errorcluster, "SolenoidDevRef"=w1646:T12)  [unwired: 9 in]
                  n672 = Greater?(x=w1623, y=w1626) -> (0:w1613:bool)
                  n673 = Greater?(x=w1624, y=w1625) -> (0:w1612:bool)
                  n674 = call-poly <vilib>:"WPI_SolenoidSet.vi"("error in (no error)"=w1648, "Value"=w1577, "SolenoidDevRef"=w1649) -> ()  [unwired: 7 in, 2 out]
                  n675 = call-poly <vilib>:"WPI_SolenoidSet.vi"("error in (no error)"=w1645, "Value"=w1627, "SolenoidDevRef"=w1646) -> ()  [unwired: 7 in, 2 out]
                  n676 = Greater?(x=w1584, y=90.0) -> (0:w1588:bool)
                  n677 = global write "Robot Global Data.vi" "Low gear - high gear"(w1577) -> ()
                  n678 = call-poly <vilib>:"PID.vi"("output range"=cluster{"output high":dbl, "output low":dbl} {"output high"=1.0, "output low"=-1.0}, "PID gains"=T5 {"proportional gain (Kc)"=1.0, "integral time (Ti, min)"=0.01, "derivative time (Td, min)"=0.0}, "process variable"=w1631, "setpoint"=w1629) -> ("output"=w1614:dbl)  [unwired: 6 in, 1 out]
                  n679 = Select(t=0.0, s=w1588, f=w1587) -> (s? t:f=w1585:dbl)
                  n680 = call <vilib>:"WPI_MotorControlRefNum Registry Get.vi"("refnum name"="Lift") -> ("error out"=w1643:errorcluster, "MotorControlDevRef"=w1644:T7)  [unwired: 9 in]
                  n681 = call <vilib>:"WPI_MotorControlRefNum Registry Get.vi"("refnum name"="Intake") -> ("error out"=w1641:errorcluster, "MotorControlDevRef"=w1642:T7)  [unwired: 9 in]
                  n682 = call <vilib>:"WPI_MotorControlRefNum Registry Get.vi"("refnum name"="Wrist") -> ("error out"=w1639:errorcluster, "MotorControlDevRef"=w1640:T7)  [unwired: 9 in]
                  n683 = Less?(x=w1578, y=0.0) -> (x < y?=w1582:bool)
                  n684 = call-poly <vilib>:"PID.vi"("output range"=cluster{"output high":dbl, "output low":dbl} {"output high"=1.0, "output low"=-1.0}, "PID gains"=T5 {"proportional gain (Kc)"=1.0, "integral time (Ti, min)"=0.01, "derivative time (Td, min)"=0.0}, "process variable"=w1630, "setpoint"=w1628) -> ("output"=w1615:dbl)  [unwired: 6 in, 1 out]
                  n685 = call <vilib>:"WPI_MotorControlSetOutput.vi"("error in (no error)"=w1641, "Output"=w1598, "MotorControlDevRef"=w1642) -> ()  [unwired: 6 in, 3 out]
                  n686 = call <vilib>:"WPI_MotorControlSetOutput.vi"("error in (no error)"=w1639, "Output"=w1585, "MotorControlDevRef"=w1640) -> ()  [unwired: 6 in, 3 out]
                  n687 = Select(t=0.0, s=w1582, f=w1580) -> (s? t:f=w1579:dbl)
                  n688 = call <vilib>:"WPI_MotorControlSetOutput.vi"("error in (no error)"=w1643, "Output"=w1579, "MotorControlDevRef"=w1644) -> ()  [unwired: 6 in, 3 out]
                  n689 = And(x=w1613, y=w1612) -> (x .and. y?=w1619:bool)
                  n690 = Select(t=0.0, s=w1613, f=w1614) -> (s? t:f=w1591:dbl)
                  n691 = Select(t=0.0, s=w1612, f=w1615) -> (s? t:f=w1590:dbl)
                  n692 = call <vilib>:"WPI_RobotDriveTankDrive.vi"("Right axis value"=w1590, "Left axis value"=w1591, "RobotDriveDevRef"=w1653) -> ("error out"=w1618:errorcluster, "Motor Values"=w1651:dbl[], "RobotDriveDevRef"=w1654:T6)  [unwired: 6 in]
                  n693 = global write "Robot Global Data.vi" "Left Reset"(w1611) -> ()
                  n694 = global write "Robot Global Data.vi" "Right Reset"(w1611) -> ()
                  n695 = call-poly <vilib>:"NT Write Value.vi"("Numeric Array"=w1651, "Name"="RobotDrive Motors") -> ()  [unwired: 9 in, 1 out]
                  n696 = Select(t=0.0, s=w1619, f=w1621) -> (s? t:f=w1620:dbl)
                }
              }
            }
            n697 = call <vilib>:"WPI_RobotDriveDelayAndUpdateSafety.vi"("error in (no error)"=w1533, "Delay (s)"=w1534, "RobotDriveDevRef"=w1538) -> ("RobotDriveDevRef 2"=w1536:T6)  [unwired: 7 in, 1 out]
          }
        }
      }
    }
  }
